vi "Core_Chem_User_Interface_v3.2.vi"() -> ()   [LabVIEW 2014]
uses:
  <vilib>/dex/Stream Element Allocation Mode.ctl
  C:/Program Files (x86)/National Instruments/LabVIEW 2014/examples/Data Communication/Network Streams/Simple Network Streams/support/Network Stream Command.ctl
  <vilib>/Platform/TimedLoop/XDataNode/timing_clust.ctl
  <vilib>/Platform/TimedLoop/XDataNode/nitl_modes.ctl
  <vilib>/Platform/TimedLoop/XDataNode/wakeup.ctl
  <vilib>/Utility/tcp.llb/UDP Multicast Read-Only Open.vi
  <vilib>/platform/TimedLoop/XDataNode/XDataNode.xnode
  <vilib>/Platform/TimedLoop/XDataNode/XDNodeRunTimeDep.lvlib
  <vilib>/FTP/NI_FTP.lvlib
panel:
  out "Create folder error out 3":errorcluster
  out "Network disconnected":bool
  out "cRIO connection status":bool
  out "Network Check error out":errorcluster
  out "SO2 Zeroing (Inflight)\nTime Remain (sec)":u32
  in  "eV6 User set time \n(Inflight) (sec)":i32=120
  in  "SO2 Inflight \nZeroing":bool
  out "Create folder error out 2":errorcluster
  out "Create folder error out":errorcluster
  in  "Confirm Flight Number":bool
  out "PRTAFT_UDP_In":string
  out "TWBOZO01":string
  out "CABOZO01":string
  out "TEIOZO01":string
  out "CHTSOO01":string
  out "CHFGGA01":string
  out "AL52CO01":string
  in  "Flight Number":string
  in  "Tab Control":T1(tab)
  out "FGGA preflight Des 17":string="Preflight - Start minimum 2 hours before take-off\n\n1. Ensure no bags/jackets are stowed on seat backs and behind seats in front of core chemistry rack at all times.\n\n2. Remove inlet covers if applicable.\n\n3. Connect Lilliput mini TFT/LCD VGA cable to FGGA VIDEO (back panel) and PS2 Keyboard/Mouse cables to FGGA Connectors (back panel). TFT/LCD screen kept in WAS/GAS rack Zargers Box. Keyboard/Mouse kept bottom of chemistry rack. (DO NOT disconnect PS2 cable). Connect TFT/LCD AC/DC PSU to 6026-8-98 Amphenol (SSP9) and make 230 Vac CB.\n\n4. Ensure all circuit breakers are pushed in, except 230Vac and 28Vdc, UPS switch off (down) and AL5002 CO Plasma Lamp switch off (down), WoW key to normal (horizontal).\n\n5. Wait for ALL network switches on the aircraft to be up and running before start-up. On the Flight Manager's Interface on the Flight Manager laptop, check SSP icons status (top row) should be all green.  \n\n6. Check AboutTime has synchronised laptop clock to aircraft timeservers (Filiberto/Gaston).\n\nClick the PowerUp Tab."
  out "FGGA preflight Des 16":string="PowerUp\n\n1.\tSSP9 forward face\tMake 3 CBs\n\n2.\tPWRDIST \t\tMake 230Vac CB \n                     Switch UPS On \t[UP]\n                     Make 28Vdc CB\n                     Check 28VDC OK Green Light comes on\n\n3.\tCore Chemistry e-Log\nComplete Core Chemistry e-Log in WordPad (Bnnn_CoreChemLog_v2.2), save on Flight Manager's laptop (192.168.101.180/      flt_folders/Bnnn); Fill in header with date, flight number and your name/initials.\n\n4. Wait for MFM flow rate to display non zero value.\n\n5.\tSAMPUMP\t\t\n - Switch WoW override key (vertical) to check pump starts, and MFM flowrate increase (>20 LPM) on the right hand plot. \n - Switch off WoW override\t\t\t\t [NORM, key horizontal]\n\nClick the 2B Ozone tab if operated, otherwise, click the UDP tab.\n\n\n"
  out "MFM":dbl(graph)
  in  "Ambient = OFF\nCabin = ON":bool
  out "FGGA preflight Des 15":string="2B Ozone Preflight\n\n1.\tSelect either Ambient or Cabin Air mode (default should be OFF for Ambient air mode).\n\n2. Check flowrate is greater than 2000 sccm on the right hand plot.\n\nClick the UDP tab."
  out "2B Ozone concentration":dbl(graph)
  out "2B Ozone flow rate":dbl(graph)
  out "2BOzone Event error out":errorcluster
  out "2BOzone command sender error out":errorcluster
  out "FGGA preflight Des 20":string="4. Check derived parameters in DECADES (192.168.101.110 & 192.168.101.108). 574 Ozone TEi49C; 588 CO AL5002; 611 SO2 TEi43i; 903 - 905 FGGA; 910 / 920 Ozone 2B."
  out "FGGA preflight Des 14":string="UDP Preflight\n1. Check all UDP packets are updating.  Unix time increasing by 1 sec (3rd parameter).\n2. Check flight number is correct.\n3. Confirm flight number and check it appears in the UDP packet (6th parameter). "
  in  "name":string="239.1.4.6"
  in  "Port":u16=50001
  out "FGGA":string
  out "CO":string
  out "TEi49 Ozone":string
  out "2B Cabin Ozone":string
  out "2B Ambient Ozone":string
  out "SO2":string
  in  "Ozone Zeroing Abort":bool
  out "Ozone Zeroing\nTime Remain (sec)":u32
  in  "Ozone Zeroing":bool
  out "TEI49 Sample Flow B":dbl(graph)
  out "TEi49 Concentration":dbl(graph)
  out "TEI49 Sample Flow A":dbl(graph)
  out "FGGA preflight Des 13":string="TEi49 Ozone PRE-FLIGHT - LAST ACTIONS BEFORE SEAT-BELTING DOWN (PRIOR TO ENGINES START)\n\n1. Ozone monitor zeroing\t\t[10 min minimum]\n\n\n2. Check TEi49 zero value and note down value in e-Log. \n"
  out "FGGA preflight Des 12":string="TEi49 Ozone Preflight\n\n1. Check nominal sample flowrate on both channels is ~0.7 LPM."
  out "Ozone Event error out":errorcluster
  out "Ozone command sender error out":errorcluster
  in  "Ozone UDP Time Offset":i32=1
  in  "eV8 span\n(sec)":i32=120
  in  "eV9 span\nflush (sec)":i32=60
  in  "SO2 Span Calibration":bool
  in  "eV9 zero\nflush (sec)":i32=15
  in  "SO2 Zero Calibration":bool
  in  "eV8 zero\n(sec)":i32=30
  in  "SO2 Calibration Abort":bool
  out "SO2 react pressure":dbl(graph)
  in  "Prepare SO2 Zero Gas":bool
  in  "Prepare SO2 Span Gas":bool
  in  "Auto Zeroing \ninterval (sec)":i32=600
  out "Next Auto Zero\nStarts in (sec)":u32
  out "Auto Zero\nIndicator":string="Auto Zero Inactive; Manual Zero Allow"
  out "SO2 Resume Zeroing\nCount down timer (sec)":u32
  in  "SO2 Pause\nAuto Zeroing":bool
  out "TEi43i Concentration scaled / raw":cluster{dbl, dbl}(graph)
  in  "SO2 Auto Zeroing":bool
  out "mean zero\ncal status":bool
  out "SO2 Sensitivity":dbl format="%.2g"
  out "SO2 Zero":dbl format="%.2g"
  in  "eV9 Flush User\nset time (sec)":i32=15
  in  "MFC_3 User Set Value":dbl=2.0
  in  "MFC_2 User Set Value":dbl=2.5
  in  "eV6 User\nset time (sec)":i32=600
  out "SO2 Flush\nTime Remain (sec)":u32
  out "TEI43i MFC3 Sample Flow":dbl(graph)
  out "TEI43C Sample Flow":dbl(graph)
  out "TEI43i MFC2 Cal Flow":dbl(graph)
  out "SO2 Zero CAL\nTime Remain (sec)":u32
  out "SO2 Zero CAL Flush\nTime Remain (sec)":u32
  in  "SO2 Zero CAL":bool
  out "FGGA preflight Des 11":string="TEi43 SO2 Inflight Zero Calibration"
  in  "SO2 GND Zeroing":bool
  out "SO2 Zeroing\nTime Remain (sec)":u32
  out "FGGA preflight Des 10":string="TEi43 SO2 PRE-FLIGHT - LAST ACTIONS BEFORE SEAT-BELTING DOWN (PRIOR TO ENGINES START)\n\n1. SO2 monitors zeroing\t\t[10 min minimum]\n\n2. Check TEi43i or TEi43C zero value and note down value in e-Log.\n\n3. Enable SO2 auto zeroing (if required) and check zeroing interval. "
  in  "SO2 Flush":bool
  out "FGGA preflight Des 9":string="TEi43 SO2 Preflight\n\n1. Check nominal sample flowrate is (2.0 LPM / 1.5 LPM) on the (TEi43i / TEi43c) right hand plot.\n\nSPAN GAS\n1. Connect SO2 Calibration gas to caldeck, then.\n\n2. Press SO2 flush button, MFC2 cal flow should increase to 2.5 SLPM.\nMonitor MFC2 flow rate to make sure the reading decreases from 2.5 SLPM to 0.0 SLPM.\nCheck pressure content and delivery gauges also reads zero.\nIf pressure content & delivery gauges do NOT read zero, press SO2 flush button again until they do.\n\n3. Back out V2, Quickly open and close cylinder valve 1, Set delivery pressure to 3 bar on V2. \n\n4. Repeat step 2) to 3) three times.\n\n5. Open cylinder valve 1, system is ready. Note down content pressure in elog.\n\n6. Press SO2 Span Calibration button to start Span calibration. \n\nZERO AIR\n1. Connect BTCA Zero Air gas to caldeck, then.\n\n2. Set ev9 flush user time to 60 secs and press SO2 Flush button.\n\n3. Press SO2 Zero Calibration button to start Zero Air calibration."
  in  "eV9 flush User\nset time (sec)":i32=30
  in  "eV8 User\nset time (sec)":i32=60
  out "SO2 Event error out":errorcluster
  out "SO2 command sender \nerror out":errorcluster
  in  "SO2 UDP Time Offset":i32=1
  in  "CO Monitor Troubleshooting":bool
  out "Lamp Temperature":dbl(graph)
  out "CO CAL Status":bool
  in  "CO CAL":bool
  out "FGGA preflight Des 8":string="CO Preflight and Inflight Calibrations\nHold down the CAL button for 2 secs then release, CAL status should then lit up.\nCheck CO LED lit up at front instrument. If not, refer to\nInflight calibration performed on 45 minutes interval or more frequently if lamp temperature > 35.5 degC."
  in  "Prepare Gases":bool
  out "FGGA preflight Des 7":string="AL5002 CO Preflight Checks\n\n1.\n\n2. Start CO Vacuum. NB: If there is problem with the software control, use manual override switch [up] on CALDECK front panel\n\n3. CO Checks - charts on the right hand side\n    Lamp Flow Controller ~ 40 ml/min\n    Monochromator Flow Controller ~ 30 ml/min\n    Fluorescence Cell Pressure ~ 7.5 Torr\n\nIf Lamp/Mono flows are low, manual valves (V1 -> V5) may still be shut, or pressure adjusting valves (ALREG1 & 2) have not been set > 2 bar\n\nIf Cell pressure is 10 Torr (max range), check that COPUMP is running and eV7 is opened (CO Vacuum eV7 is ON).\n\n4. Switch Plasma Lamp at the front panel UP\n\nDetector count rate (on 'Raw Signal' or F2 instrument touchscreen) should increase to >=10000 Hz within a minute.  Recycle plasma lamp switch (off/on) if no significant increase in count rate after 10 mins.  CO concentration should increase (100s ppb). \n     \n\n"
  in  "CO Vaccum (eV7)":bool
  out "Raw Signal":dbl(graph)
  out "CO Concentration":dbl(graph)
  out "Fluorescence Cell Pressure":dbl(graph)
  out "Monochromator Flow":dbl(graph)
  out "Lamp Flow Controller":dbl(graph)
  in  "CO UDP Time Offset":i32=1
  out "CO2 Pressure\nDelivery (PSIA)":dbl(slide) scale=0.0..100.0
  out "Std\nContent (barG)":dbl(slide) scale=0.0..220.0
  out "N2\nContent (barG)":dbl(slide) scale=0.0..220.0
  out "CO2\nContent (barG)":dbl(slide) scale=0.0..170.0
  out "CO Event error out":errorcluster
  out "CO command sender error out":errorcluster
  out "CO Zero":T2(array[cluster])
  out "CO Sensitivity":T3(array[cluster])
  in  "NEW\nFGGA Restart":bool
  in  "FGGA Calibration Abort":bool
  out "Ring Down Time RDA & RDB":cluster{dbl, dbl}(graph)
  in  "Line Lock Setting Change":bool
  out "Cell temperature":dbl(graph)
  out "Cell pressure":dbl(graph)
  in  "Manual FGGA Pump":bool
  out "CO2":dbl(graph)
  out "CH4":dbl(graph)
  out "H2O":dbl(graph)
  out "WoW Flag":string="0"
  in  "FGGA pump\nsync to WoW":bool
  out "CH4 Dry":dbl(graph)
  out "CO2 Dry":dbl(graph)
  out "MFC1 Cal Flow":dbl(graph)
  out "Flush Target Tank\nTime Remain (sec)":u32
  out "Flush Low Tank\nTime Remain (sec)":u32
  out "Flush High Tank\nTime Remain (sec)":u32
  in  "Flush Target Tank":bool
  in  "Flush Low Tank":bool
  in  "Flush High Tank":bool
  in  "OLD\nFGGA Restart":bool
  out "FGGA preflight Des 6":string="FGGA Instrument Controls"
  in  "High Cal":bool
  out "High Cal\nFlush Time Remain (sec)":u32
  out "High Cal\nCal Time Remain (sec)":u32
  in  "Low Cal":bool
  in  "Target Cal":bool
  in  "Span Cal - \nHigh Cal, CO Cal, Low Cal":bool
  out "Low Cal\nFlush Time Remain (sec)":u32
  out "Low Cal\nCal Time Remain (sec)":u32
  out "Target Cal\nFlush Time Remain (sec)":u32
  out "Target Cal\nCal Time Remain (sec)":u32
  in  "MFC_1 User Set Value":dbl=2.0
  out "FGGA preflight Des 5":string="FGGA Inflight Calibrations"
  out "FGGA preflight Des 4":string="FGGA Ground Preflight Checks\n\n1. Switch FGGA pump ON\n\n2. Check cavity pressure ~50 Torr\n\n3. Switch FGGA pump OFF\n\n4. Enable FGGA pump sync to WoW\n\n5.. Check Time Synchronisation\n\n6. Check CO2 & CH4 values\n\nIf CO2 & CH4 values are -1 ppm, follow the \nchange linelock settings procedure.\n\n\n\n\n\nLAST ACTION BEFORE SEAT-BELTING \nDOWN (PRIOR TO ENGINES START)\n\n1. Disconnect Monitor & stow away. Leave Keyboard & Mouse connected. Place keyboard at the bottom\nof the rack.\n\n"
  out "FGGA preflight Des 3":string="FGGA CAL Gas Purge\n\nFor each cylinder in gas stowage, check that,\n\n1. V1 Closed\n    V3 Closed\n    V4 Make sure arrow positioned downwards (i.e. flow points to gas line)\n\n2. V3 Open (turn anti-clockwise)\n\n3. Use the button on the right according to the operating cylinder to flush the line. Monitor the MFC flow rate to make sure the reading decreases from 3 to zero. (ie fully flushed). Pressure content & delivery gauges should also read zero.\n\n4. V3 Close (turn clockwise)\n\n5. V1 Open / Close quickly\n         Check delivery pressure gauge is ~ 40 PSI \n         (Use V2 to increase if necessary)\n\n6. Repeat steps 2) to 5) three times\n\n7. V3 Close (turn clockwise)\n\n8. V1 Open, check V2 ~ 40 PSIG\n\n9. V3 Open - System is ready"
  out "FGGA command sender error out":errorcluster
  out "FGGA Event Error out":errorcluster
  in  "FGGA UDP Time Offset":i32=1
  in  "NEW FGGA Shutdown":bool
  in  "Transfer NEW FGGA Files":bool
  in  "OLD FGGA Shutdown":bool
  in  "Postflight Procedures":bool
  in  "FTP ASCII Files to Local":bool
  in  "Transfer OLD FGGA Files":bool
  out "FGGA preflight Des 18":string="Postflight\n\n1. Perform SO2 Span Gas Calibration (if necessary). \n\n2. Press the FTP ASCII File to Local button to transfer ASCII files to flight folder.\n\n\n3. Press the Transfer FGGA Files button to transfer FGGA files to flight folder. \n\n\n4. Shutdown FGGA.\n\n\n5. View Postflight Procedures."
  out "File List":string[](array[string])
  out "FGGA File Transfer Error out":errorcluster
  out "Move to FM Error out":errorcluster
  out "FGGA File Transfer Error out 2":errorcluster
  out "USB Disk Space Used %":dbl(slide) scale=0.0..100.0
  out "PTP Sync":bool
  out "CPU Total %":dbl(graph)
  out "PRTAFT_DLU":string
  in  "Pause Auto Zero Count \nDown set time (sec)":i32=600
  out "Calibration gas cylinder \nconcentration (ppb)":dbl format="%.4g"
  in  "Save Calibration gas\ncylinder concentration to file":bool
  in  "Calibration gas cylinder \nconcentration (ppb)":dbl=500.0 format="%.4g"
  in  "Simulate MOCCA Conc":dbl
  in  "MOCCA window \ndelay time (sec)":i32=30
  in  "MOCCA Limit":i32=800
  in  "SO2 Inflight MOCCA Alarm\n(default = OFF)":bool
  in  "Offset Mean Zero Calculation (default = ON)\nOFF = User input\nOn = Mean zero calculated with ev8":bool=TRUE
  out "FGGA preflight Des 19":string="This tab controls ONLY for advanced operators."
  in  "Inst_alm_thresh":i32=220
  in  "3hr_alm_thresh":i32=80
  in  "Simulate Inst Conc":i32
  in  "Simulate 3hr Average Conc":dbl
  in  "Simulate 2B Conc":bool
  in  "Ozone eV6":bool
  in  "Simulate Conc":bool
  in  "8hr TWA Limit":i32=490
  in  "10mins STEL Limit":i32=800
  in  "SO2 Sensitivity":dbl=1.1
  in  "SO2 Zero":dbl
  in  "Simulate TWA Conc":dbl
  in  "Simulate STEL Conc":dbl
  in  "MFC_3\nSLPM Value":dbl=2.0
  in  "MFC_2\nSLPM Value":dbl
  in  "SO2 eV6":bool
  in  "eV8":bool
  in  "eV9":bool
  in  "eV4":bool
  in  "eV3":bool
  in  "MFC_1\nSLPM Value":dbl
  in  "eV2":bool
  in  "eV1":bool
  in  "cRIO File IO Stop\n(USB Flash Drive Unmount)":bool
  # "Unix time"
  # "Flight Number"
  # "concentration (scaled)\npmt_volt\nlamp_volt\nlamp_intens\ninternal_temper\nreact_temper\nreact_press\nflow\nflags\nten_min_so2\neight_hr_so2\nten_min_so2_alm\neight_hr_so2_alm\nMFC_2absolute_pres\nMFC_2temperature\nMFC_2volumetic_flow\nMFC_2mass_flow\nMFC_2set_point\nMFC_3_absolute_pres\nMFC_3_temperature\nMFC_3volumetic_flow\nMFC_3mass_flow\nMFC_3set_point\nV6\nV8\nV9\nMFC2_Set_Value\nMFC3_Set_Value\nconcentration (raw)\nmean calculation status\noffset\nsensitivity\nev8_user_set_time\nauto_zeroing_control\nev8_zero_interval\nMOCCA_inflight_alarm\nMOCCA_time_window_delay\nMOCCA_SO2_limit\n10 min STEL limit\n8 hour TWA limit\nSO2 cal gas cylin conc\nsimulate_SO2_conc_control\nMOCCA_SO2_sim_value\nMOCCA_SO2_alarm"
  # "Unix time"
  # "Unix time"
  # "Unix time"
  # "Unix time"
  # "Flight Number"
  # "Flight Number"
  # "Flight Number"
  # "Flight Number"
  # "conc\ntemp\npress\nflow\nthreehr_oz\nInst_alarm\nthreehr_alarm"
  # "ch4\nco2\nh2o\npress_torr\ntemp_c\nfit_flag\nrda_usec\nrdb_usec\nch4_dry\nco2_dry\nMFC_1_absolute_pres\nMFC_1_temperature\nMFC_1volumetic_flow\nMFC_1mass_flow\nMFC_1set_point\nV1\nV2\nV3\nV4\nrestart_FGGA\nFGGA_Pump\nCAL_MFC_1Set_Value"
  # "conc\ntemp\npress\nflow"
  # "conc\nbenchtemp\npress\ncellAint\ncellBint\nFlowA\nFlowB\nlamptemp\nflag\nV6"
  # "conc\ncounts\nsens\nzero\nlampflow\nlamptemp\nmonoflow\nmonotemp\nmonopress\ncellpress\ncalpress\ntemppmt\ncalconc\nerr\ncal_counter\nerr_counter\nCO_vacuum_status\nIn_Cal\nALEG1_press_delivery\nALREG1_press_content\nALREG2_press_content\nALREG3_press_content"
  # "TEi43c"
  # "TEi43i"
  # "SO2 Inflight ZERO CAL SETTINGS"
  # "FGGA"
  # "2B Ozone"
  # "TEi49C  - Ozone"
  # "TEi43 - SO2"
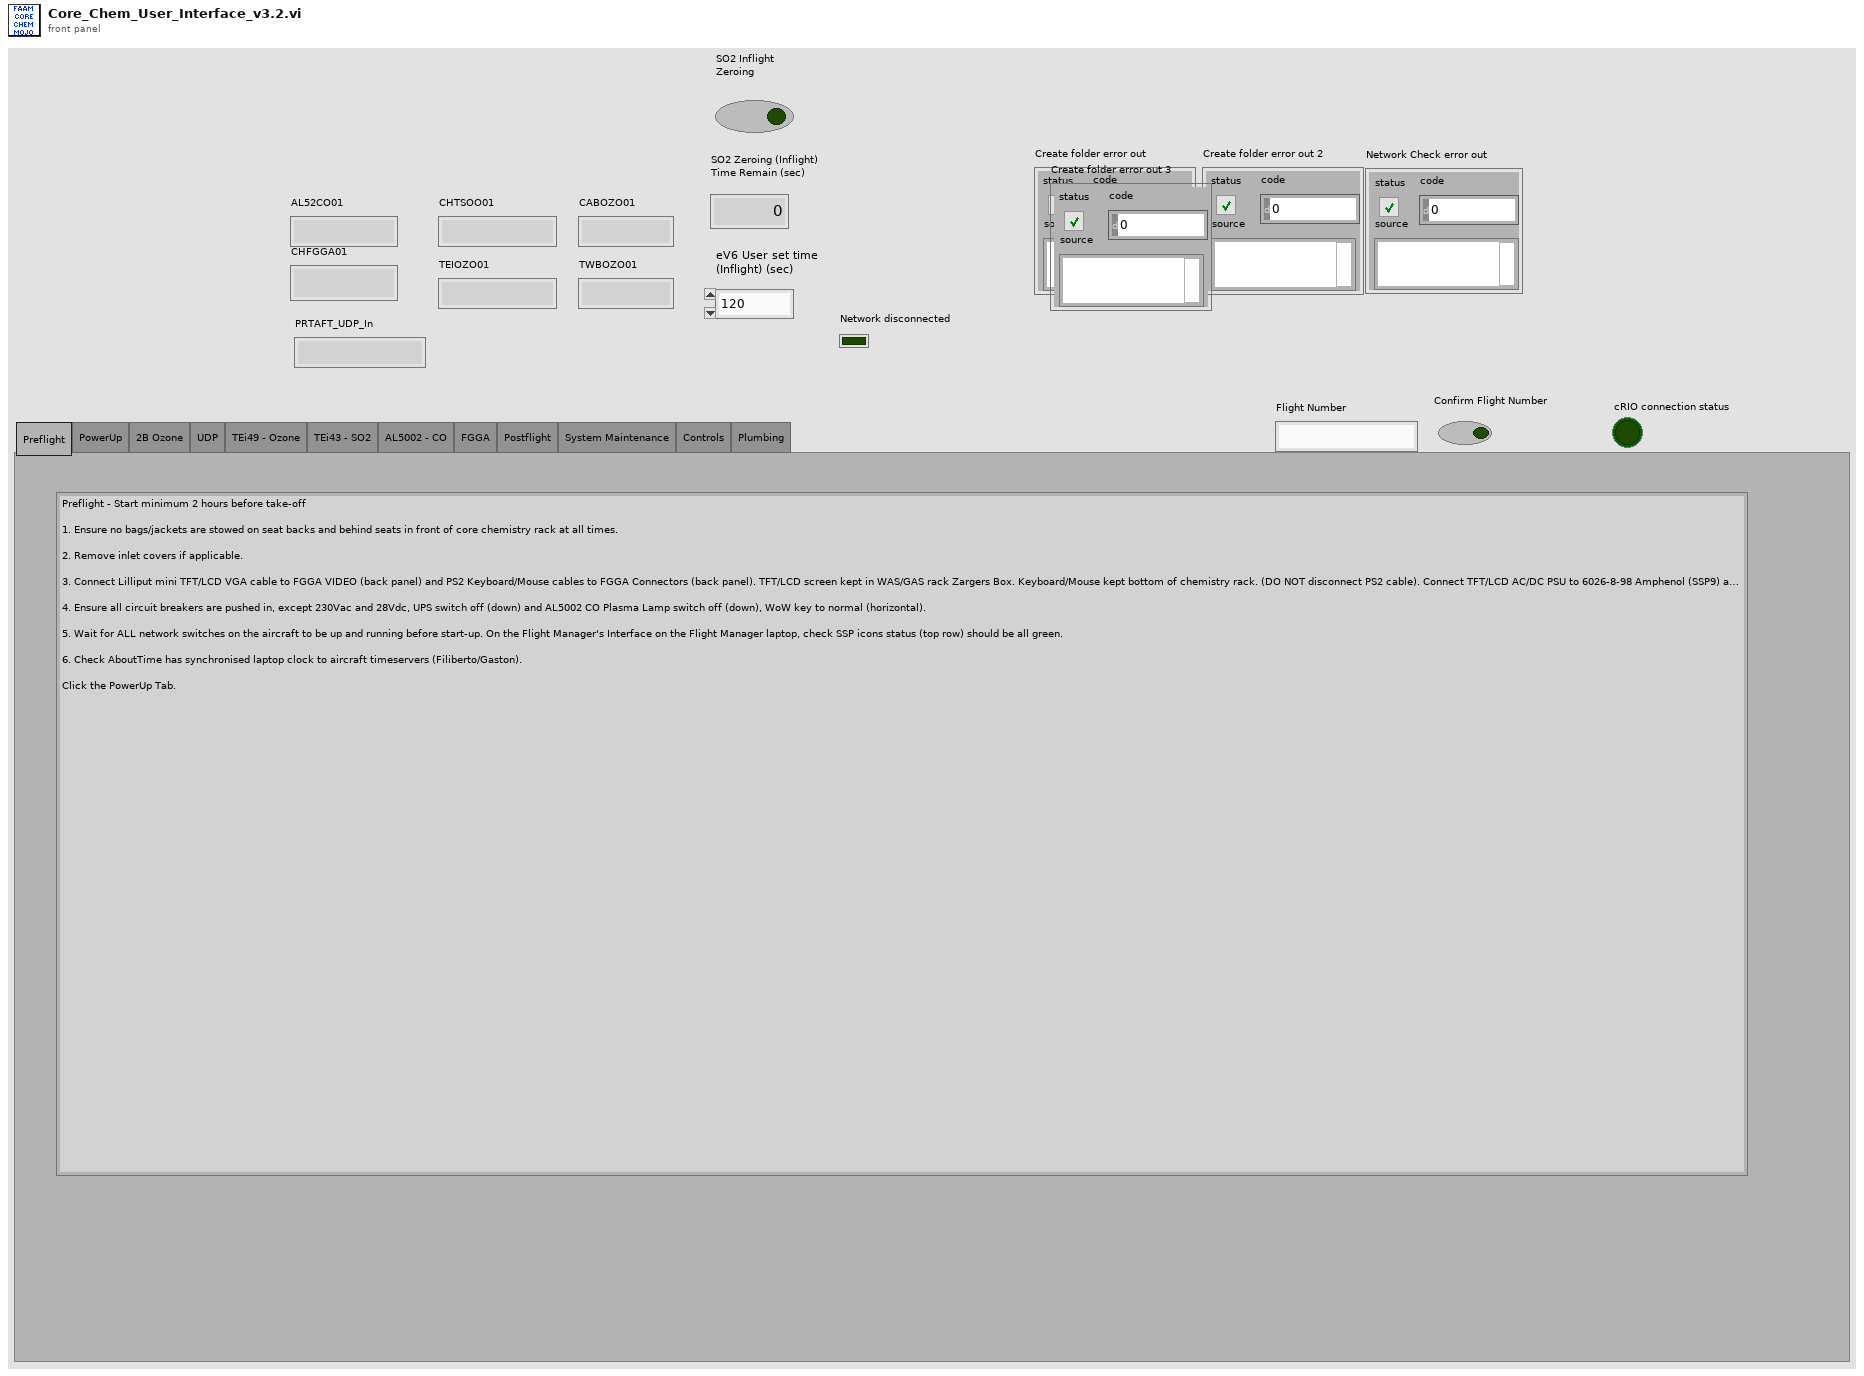
[diagram p1: front panel]
types:
  T1 = enum32{"Preflight", "PowerUp", "2B Ozone", "UDP", "TEi49 - Ozone", "TEi43 - SO2", "AL5002 - CO", "FGGA", "Postflight", "System Maintenance", "Controls", "Plumbing"}
  T2 = cluster{"time stamp":timestamp, "CO Offset":dbl}[]
  T3 = cluster{"time stamp":timestamp, "CO Sensitivity":dbl}[]
  T4 = typedef "Network Stream Command.ctl" = cluster{"Message":string, "Message Data":variant}
  T5 = typedef "Stream Element Allocation Mode.ctl" = u32
  T6 = typedef "XDNodeRunTimeDep.lvlib/timing_clust.ctl" = cluster{"Expected End [f-1]":u64, "Actual End [f-1]":u64, "Finished Late? [f-1]":bool, "Expected End [i-1]":u64, "Actual End [i-1]":u64, "Finished Late? [i-1]":bool, "Expected Start [i]":u64, "Actual Start [i]":u64, "Expected Start [f]":u64, "Actual Start [f]":u64, "Source Name":string, "Structure Name":string, "Period":i64, "Deadline":i64, "Offset":i64, "Start":i64, "Priority":i32, "Timeout":i32, "Mode":T7, "Wakeup Reason":T8, "Error":errorcluster, "Source Type":string, "Secondary Source Type":string, "Global End Time":u64, "Global Start Time":u64, "Frame Duration":u64, "Iteration Duration":u64, "Assigned CPU":i32, "I/O Scan Engine Mode":u32}
  T7 = typedef "XDNodeRunTimeDep.lvlib/nitl_modes.ctl" = enum32{"No Change", "Process missed periods, maintain original phase", "Discard missed periods, maintain original phase", "Process missed periods, ignore original phase", "Discard missed periods, ignore original phase"}
  T8 = typedef "XDNodeRunTimeDep.lvlib/wakeup.ctl" = enum32{"Normal", "Aborted", "Asynchronous wakeup", "Timing source error", "Timed loop error", "Timeout"}
  T9 = typedef "NI_FTP.lvlib/FTP Session.ctl" = refnum<k5>
  T10 = typedef "NI_FTP.lvlib/FTP File Info.ctl" = cluster{"type":enum16{"unknown", "file", "dir", "link"}, "permissions":string, "owner":string, "group":string, "size":i32, "date":string, "name":string, "link name":string}
  T11 = cluster{"Message":string, "Message 2":string, "Message 3":string}
  T12 = cluster{"Message":string, "Message 2":string, "Message 3":string, "Message 4":string}
  T13 = cluster{"Message":string, "Message 3":string, "Message 4":string}
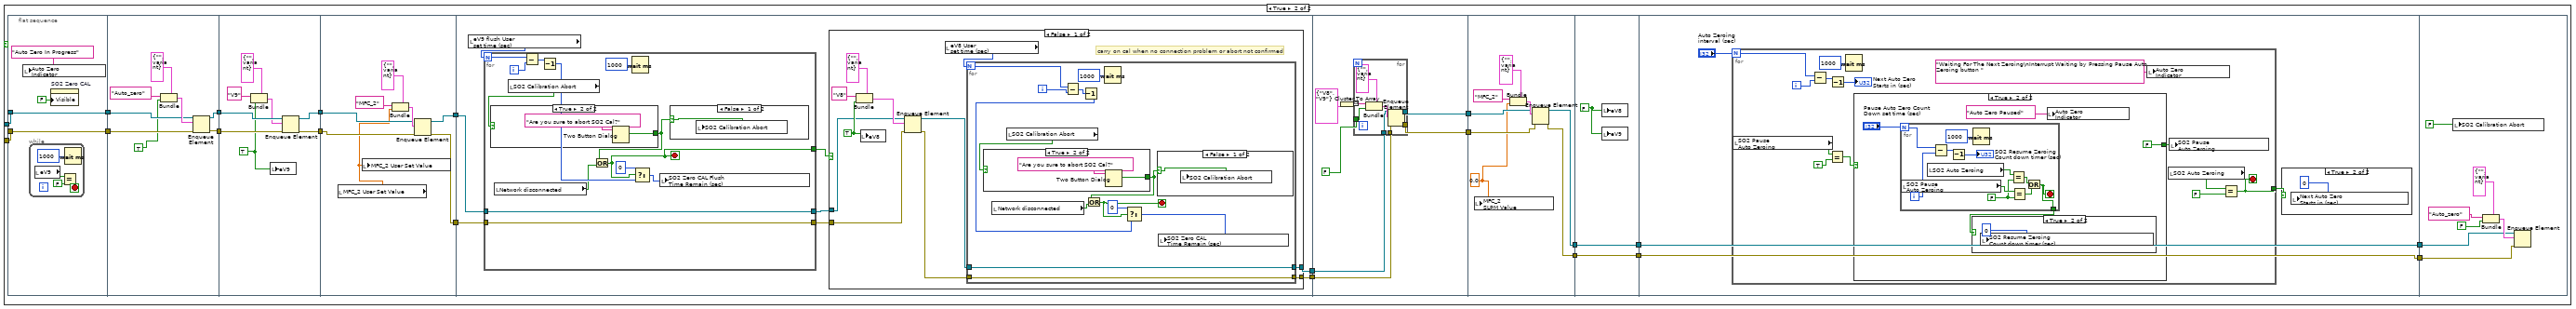
[diagram p6: hidden frame]
diagram:
  w8 = "XXXX"
  w10 = 0
  w11 = 0.0
  w17 = T4 {"Message"="", "Message Data"=variant} ("Message Cluster")
  w23 = T5 0 items=["allocate as needed", "pre-allocate"] ("element allocation mode")
  w29 = T4 {"Message"="", "Message Data"=variant} ("Message Cluster")
  w35 = T5 0 items=["allocate as needed", "pre-allocate"] ("element allocation mode")
  w40 = T4 {"Message"="", "Message Data"=variant} ("Message Cluster")
  w45 = T5 0 items=["allocate as needed", "pre-allocate"] ("element allocation mode")
  w54 = T5 0 items=["allocate as needed", "pre-allocate"] ("element allocation mode")
  w56 = T4 {"Message"="", "Message Data"=variant} ("Message Cluster")
  w63 = T5 0 items=["allocate as needed", "pre-allocate"] ("element allocation mode")
  w65 = T4 {"Message"="", "Message Data"=variant} ("Message Cluster")
  n1 = local write "cRIO File IO Stop\n(USB Flash Drive Unmount)"(FALSE ("Stop File Write")) -> ()
  n2 = local write "Flight Number"(w8) -> ()
  n3 = while {
    shift-right: [w69] -> _
    shift-left: w8 -> [w68]
    stop <- FALSE stop-if-true
    n4 = Not Equal?(x=w68, y="Flight Number") -> (x != y?=w71:bool)
    n5 = case shown="True" w71 {
      tunnel: [w74 w75] -> w69
      tunnel: "Flight Number" -> [_ w75]
      tunnel: w68 -> [w74 _]
      frame False {
      }
      frame True {
        n6 = One Button Dialog(message="Flight Number changed,\nPress flight number button to confirm") -> ()  [unwired: 1 in, 1 out]
      }
    }
    n7 = Wait (ms)(milliseconds to wait=u32 1000) -> ()  [unwired: 1 out]
  }
  n8 = while {
    stop <- FALSE stop-if-true
    # "UDP Read"
    n9 = String To IP(1:"name") -> (0:w82:u32)
    n10 = call-poly <vilib>:"UDP Multicast Open.vi"("multicast addr"=w82, "port"="Port") -> ("error out"=w80:errorcluster, "connection ID"=w79:refnum<k16>)  [unwired: 7 in, 1 out]
    n11 = Wait (ms)(milliseconds to wait=u32 1000) -> ()  [unwired: 1 out]
    n12 = case shown="No Error" w80 {
      selector: w80 -> [w86 _]
      tunnel: w79 -> [w85 _]
      frame No Error {
        w84 = ""
        n13 = while {
          tunnel: w86 -> [w132]
          tunnel: w85 -> [w131]
          shift-right: [w127] -> _
          shift-left: w84 -> [w128]
          shift-right: [w118] -> _
          shift-left: w84 -> [w120]
          shift-right: [w112] -> _
          shift-left: w84 -> [w114]
          shift-right: [w106] -> _
          shift-left: w84 -> [w107]
          shift-right: [w100] -> _
          shift-left: w84 -> [w101]
          shift-right: [w94] -> _
          shift-left: w84 -> [w95]
          shift-right: [w88] -> _
          shift-left: w84 -> [w89]
          stop <- w130 stop-if-true
          n14 = UDP Read(connection ID=w131, 8:w132) -> (data out=w87:string, error out=w130:errorcluster)  [unwired: 2 in, 3 out]
          n15 = Match Pattern(string=w87, regular expression="$TEIOZO") -> (match substring=w126:string, after substring=w125:string)  [unwired: 1 in, 2 out]
          n16 = Match Pattern(string=w87, regular expression="$TWBOZO01,") -> (match substring=w104:string, after substring=w103:string)  [unwired: 1 in, 2 out]
          n17 = Match Pattern(string=w87, regular expression="$CABOZO01,") -> (match substring=w110:string, after substring=w109:string)  [unwired: 1 in, 2 out]
          n18 = Match Pattern(string=w87, regular expression="$CHTSOO") -> (match substring=w98:string, after substring=w97:string)  [unwired: 1 in, 2 out]
          n19 = Match Pattern(string=w87, regular expression="$CHFGGA") -> (match substring=w122:string, after substring=w121:string)  [unwired: 1 in, 2 out]
          n20 = Match Pattern(string=w87, regular expression="$AL52CO01,") -> (match substring=w116:string, after substring=w115:string)  [unwired: 1 in, 2 out]
          n21 = Match Pattern(string=w87, regular expression="$PRTAFT01,") -> (match substring=w93:string, after substring=w92:string)  [unwired: 1 in, 2 out]
          n22 = Concatenate Strings(w126, w125) -> (w124:string)
          n23 = Concatenate Strings(w104, w103) -> (w102:string)
          n24 = Concatenate Strings(w110, w109) -> (w108:string)
          n25 = Concatenate Strings(w98, w97) -> (w96:string)
          n26 = Concatenate Strings(w122, w121) -> (w119:string)
          n27 = Concatenate Strings(w116, w115) -> (w113:string)
          n28 = Concatenate Strings(w93, w92) -> (w90:string)
          n29 = Replace Substring(4:w102, 5:w101) -> (1:w100:string)  [unwired: 2 in, 1 out]
          "TWBOZO01" <- w100
          n30 = Replace Substring(4:w124, 5:w128) -> (1:w127:string)  [unwired: 2 in, 1 out]
          "TEIOZO01" <- w127
          n31 = Replace Substring(4:w108, 5:w107) -> (1:w106:string)  [unwired: 2 in, 1 out]
          "CABOZO01" <- w106
          n32 = Replace Substring(4:w96, 5:w95) -> (1:w94:string)  [unwired: 2 in, 1 out]
          "CHTSOO01" <- w94
          n33 = Replace Substring(4:w113, 5:w114) -> (1:w112:string)  [unwired: 2 in, 1 out]
          "AL52CO01" <- w112
          n34 = Replace Substring(4:w119, 5:w120) -> (1:w118:string)  [unwired: 2 in, 1 out]
          "CHFGGA01" <- w118
          n35 = Replace Substring(4:w90, 5:w89) -> (1:w88:string)  [unwired: 2 in, 1 out]
          "PRTAFT_UDP_In" <- w88
        }
      }
      frame Error {
      }
    }
  }
  n36 = Obtain Queue(name (unnamed)="CO_Command", element data type=w65) -> (queue out=w16:refnum<queue>, error out=w59:errorcluster)  [unwired: 3 in, 1 out]
  n37 = Create Network Stream Writer Endpoint(6:w63, 7:10 ("writer buffer size"), 9:w65, 10:"//192.168.101.17/command/reader/CO" ("reader url"), 11:"/command/writer/CO" ("writer name")) -> (0:w62:errorcluster, 3:w61:refnum<k21>)  [unwired: 2 in]
  n38 = while {
    tunnel: w16 -> [w136]
    tunnel: w59 -> [w135]
    tunnel: [w133] -> _
    stop <- FALSE stop-if-true
    # "CO UI Event Handler Loop"
    n39 = event shown="[4] \"Confirm Flight Number\": Value Change" {
      selector: _ -> [_ _ _ _ _]
      dyn-events: _ -> [_ _ _ _ _]
      timeout: _ -> [_ _ _ _ _]
      tunnel: w136 -> [w143 w150 w154 w161 w169]
      tunnel: w135 -> [w142 w149 w153 w160 w168]
      tunnel: [w137 w144 w152 w159 w167] -> w133
      event "CO CAL": Value Change {
        n40 = event-data() -> ("NewVal"=w140:bool)  [unwired: 1 in]
        n41 = Bundle(cluster=T4 {"Message"="", "Message Data"=variant} ("Message Cluster"), "Message"="CO CAL", "Message Data"=w140) -> (w138:T4)
        n42 = Enqueue Element(queue=w143, element=w138, error in (no error)=w142) -> (error out=w137:errorcluster)  [unwired: 1 in, 2 out]
      }
      event "CO UDP Time Offset": Value Change {
        n43 = event-data() -> ("NewVal"=w147:i32)  [unwired: 1 in]
        n44 = Bundle(cluster=T4 {"Message"="", "Message Data"=variant} ("Message Cluster"), "Message"="UDP Time Offset", "Message Data"=w147) -> (w145:T4)
        n45 = Enqueue Element(queue=w150, element=w145, error in (no error)=w149) -> (error out=w144:errorcluster)  [unwired: 1 in, 2 out]
      }
      event "CO Vaccum (eV7)": Value Change {
        n46 = event-data() -> ("NewVal"=w151:bool)  [unwired: 1 in]
        n47 = Bundle(cluster=T4 {"Message"="", "Message Data"=variant} ("Message Cluster"), "Message"="CO Vacuum", "Message Data"=w151) -> (w155:T4)
        n48 = Enqueue Element(queue=w154, element=w155, error in (no error)=w153) -> (error out=w152:errorcluster)  [unwired: 1 in, 2 out]
      }
      event "cRIO File IO Stop\n(USB Flash Drive Unmount)": Value Change {
        n49 = event-data() -> ("NewVal"=w158:bool)  [unwired: 1 in]
        n50 = Bundle(cluster=T4 {"Message"="", "Message Data"=variant} ("Message Cluster"), "Message"="Stop File Write", "Message Data"=w158) -> (w162:T4)
        n51 = Enqueue Element(queue=w161, element=w162, error in (no error)=w160) -> (error out=w159:errorcluster)  [unwired: 1 in, 2 out]
      }
      event "Confirm Flight Number": Value Change {
        n52 = event-data() -> ()  [unwired: 1 in, 1 out]
        n53 = flat-sequence {
          tunnel: w168 -> [w171]
          tunnel: w169 -> [w172]
          tunnel: [w172] -> w166
          tunnel: [w171] -> w165
          tunnel: [w174] -> w167
          tunnel: w166 -> [w176]
          tunnel: w165 -> [w175]
          frame #0 {
            n54 = local write "cRIO File IO Stop\n(USB Flash Drive Unmount)"(FALSE ("cRIO File IO Stop\n(USB Flash Drive Unmount)")) -> ()
          }
          frame #1 {
            n55 = local read "Flight Number"() -> (w173:string)
            n56 = Bundle(cluster=T4 {"Message"="", "Message Data"=variant} ("Message Cluster"), "Message"="Flight Number", "Message Data"=w173) -> (w177:T4)
            n57 = Enqueue Element(queue=w176, element=w177, error in (no error)=w175) -> (error out=w174:errorcluster)  [unwired: 1 in, 2 out]
          }
        }
      }
    }
    "CO Event error out" <- w133
  }
  n58 = while {
    tunnel: w16 -> [w187]
    shift-right: [w182] -> _
    shift-left: w61 -> [w184]
    shift-right: [w180] -> w50
    shift-left: w62 -> [w186]
    tunnel: w59 -> [w181]
    stop <- w180 stop-if-true
    # "CO UI Command Sender"
    n59 = Dequeue Element(queue=w187, error in (no error)=w181) -> (element=w183:T4)  [unwired: 1 in, 3 out]
    n60 = Unbundle By Name(w183) -> ("Message"=w185:string)
    n61 = case shown="\"UDP Time Offset\"" w185 {
      tunnel: w186 -> [w188 w192 w199 w206 w213 w220]
      tunnel: w184 -> [w189 w195 w202 w209 w216 w223]
      tunnel: w183 -> [_ w194 w201 w208 w215 w222]
      tunnel: [w188 w191 w198 w205 w212 w219] -> w180
      tunnel: [w189 w190 w197 w204 w211 w218] -> w182
      frame "False", Default {
      }
      frame "CO CAL" {
        n62 = shared-variable-write(w195, w192, w194) -> (w193:refnum<k21>, w196:errorcluster)  [unwired: 1 in, 1 out]
        n63 = Flush Stream(8:w196, 11:w193) -> (0:w191:errorcluster, 3:w190:refnum<k21>)  [unwired: 2 in, 1 out]
      }
      frame "UDP Time Offset" {
        n64 = shared-variable-write(w202, w199, w201) -> (w200:refnum<k21>, w203:errorcluster)  [unwired: 1 in, 1 out]
        n65 = Flush Stream(8:w203, 11:w200) -> (0:w198:errorcluster, 3:w197:refnum<k21>)  [unwired: 2 in, 1 out]
      }
      frame "Stop File Write" {
        n66 = shared-variable-write(w209, w206, w208) -> (w207:refnum<k21>, w210:errorcluster)  [unwired: 1 in, 1 out]
        n67 = Flush Stream(8:w210, 11:w207) -> (0:w205:errorcluster, 3:w204:refnum<k21>)  [unwired: 2 in, 1 out]
      }
      frame "Flight Number" {
        n68 = shared-variable-write(w216, w213, w215) -> (w214:refnum<k21>, w217:errorcluster)  [unwired: 1 in, 1 out]
        n69 = Flush Stream(8:w217, 11:w214) -> (0:w212:errorcluster, 3:w211:refnum<k21>)  [unwired: 2 in, 1 out]
      }
      frame "CO Vacuum" {
        n70 = shared-variable-write(w223, w220, w222) -> (w221:refnum<k21>, w224:errorcluster)  [unwired: 1 in, 1 out]
        n71 = Flush Stream(8:w224, 11:w221) -> (0:w219:errorcluster, 3:w218:refnum<k21>)  [unwired: 2 in, 1 out]
      }
    }
  }
  "CO command sender error out" <- w50
  n72 = node-c288() -> (w15:T6)  [unwired: 4 in]
  n73 = Initialize Array(cluster{"time stamp":timestamp, "Y":dbl} {"time stamp"=timestamp(0 s since 1904-01-01), "Y"=0.0}, 30 ("dimension size")) -> (w12:cluster{"time stamp":timestamp, "Y":dbl}[])
  n74 = timed-loop {
    timing: w15 -> [_]
    timing-out: [_] -> w14
    stop <- _ stop-if-true
    # "PC Tasks"
    n75 = node-c288() -> ()  [unwired: 1 in, 1 out]
    n76 = event shown="[2] \"Transfer NEW FGGA Files\": Value Change" {
      selector: _ -> [_ _ _ _ _ _ _]
      dyn-events: _ -> [_ _ _ _ _ _ _]
      timeout: _ -> [_ _ _ _ _ _ _]
      event "FTP ASCII Files to Local": Value Change {
        n77 = event-data() -> ()  [unwired: 1 in, 1 out]
        n78 = flat-sequence {
          tunnel: [w233] -> w227
          tunnel: [w245] -> w232
          tunnel: [w244] -> w230
          tunnel: [w243] -> w228
          tunnel: w227 -> [w243]
          tunnel: w232 -> [w303]
          tunnel: [w303] -> w231
          tunnel: w230 -> [w299]
          tunnel: [w298] -> w229
          tunnel: w228 -> [w298]
          tunnel: w231 -> [w309]
          tunnel: w229 -> [w304]
          frame #0 {
            n79 = local read "Flight Number"() -> (w235:string)
            n80 = Concatenate Strings("Confirm Flight Number" ("message"), "\n", w235) -> (w239:string)
            n81 = Two Button Dialog(message=w239, 1:"No" ("F button name (\"Cancel\")"), 2:"Yes" ("T button name (\"OK\")")) -> (T button?=w236:bool)
            n82 = case shown="False" w236 {
              tunnel: w235 -> [_ w242]
              tunnel: [w241 w242] -> w233
              frame False {
                n83 = call "Prompt User for Flight Number2"() -> ("Flight Number BXXX"=w241:string)  [unwired: 17 in, 2 out]
              }
              frame True {
              }
            }
          }
          frame #1 {
            n84 = Get Date/Time In Seconds() -> (seconds since 1Jan1904=w249:timestamp)
            n85 = Format Date/Time String(time format string (%c)="%Y%m%d", seconds (now)=w249) -> (date/time string=w247:string)  [unwired: 1 in]
            n86 = call <vilib>:"FTP Open Session.vi"("address"="192.168.101.17") -> ("error out"=w264:errorcluster, "ftp session"=w265:T9)  [unwired: 7 in, 2 out]
            n87 = Concatenate Strings("Use Today's Date" ("message"), "\r", w247) -> (w253:string)
            n88 = call <vilib>:"FTP Logon.vi"("error in (no error)"=w264, "password"="", "user"="anonymous", "ftp session"=w265) -> ("error out"=w261:errorcluster, "ftp session out"=w260:T9)  [unwired: 4 in, 2 out]
            n89 = Two Button Dialog(message=w253, 1:"No" ("F button name (\"Cancel\")"), 2:"Yes" ("T button name (\"OK\")")) -> (T button?=w250:bool)
            n90 = case shown="False" w250 {
              tunnel: [w268 w269] -> w244
              tunnel: w247 -> [_ w269]
              frame False {
                n91 = call "Prompt User for Date"() -> ("Date"=w268:string)  [unwired: 17 in, 2 out]
              }
              frame True {
              }
            }
            n92 = call <vilib>:"FTP Directory Listing.vi"("error in (no error)"=w261, "directory path"="/U:/data", "ftp session"=w260) -> ("dir list"=w259:T10[])  [unwired: 4 in, 4 out]
            n93 = for {
              tunnel: w259 -> [w289] mode=indexing
              tunnel: [w288] -> w256 mode=indexing
              tunnel: w244 -> [w287]
              # "Extract File Name According to the Date"
              n94 = Unbundle By Name(w289) -> ("name"=w295:string, "name"=w294:string)
              n95 = Match Pattern(string=w294, regular expression="_[0-9]+") -> (match substring=w292:string)  [unwired: 1 in, 3 out]
              n96 = String Subset(string=w292, offset (0)=1) -> (substring=w290:string)  [unwired: 1 in]
              n97 = Equal?(x=w290, y=w287) -> (x = y?=w296:bool)
              n98 = case shown="False" w296 {
                tunnel: w295 -> [_ w297]
                tunnel: [_ w297] -> w288
                frame False {
                }
                frame True {
                }
              }
            }
            n99 = Array Size(array=w256) -> (size(s)=w258:i32)
            n100 = for {
              N: w258 -> [_]
              shift-right: [w276] -> w246
              shift-left: w256 -> [w277]
              shift-right: [w274] -> _
              shift-left: 0 -> [w275]
              # "Remove Empty Array"
              n101 = Index Array(array=w277, index=w275) -> (element=w279:string)
              n102 = Equal?(x=w279, y="") -> (x = y?=w278:bool)
              n103 = case shown="True" w278 {
                tunnel: w277 -> [w283 w286]
                tunnel: w275 -> [w282 w284]
                tunnel: [w283 w285] -> w276
                tunnel: [w281 w284] -> w274
                frame False {
                  n104 = Increment(x=w282) -> (x+1=w281:i32)
                }
                frame True {
                  n105 = Delete From Array(array=w286, index=w284) -> (array with subset deleted=w285:string[])  [unwired: 1 in, 1 out]
                }
              }
            }
            "File List" <- w246
            n106 = for {
              tunnel: w246 -> [w272] mode=indexing
              tunnel: [w270] -> w245 mode=indexing
              # "Specify destination path for each file"
              n107 = Concatenate Strings("C:\\temp\\", w272) -> (w271:string)
              n108 = String To Path(string=w271) -> (path=w270:path)
            }
          }
          frame #2 {
            # "FTP a list of files"
            n109 = call <vilib>:"System Exec.vi"("wait until completion? (T)"=TRUE, "working directory"=path "C:/temp", "standard input"=w299, "command line"="C:\\temp\\transfer_ascii_files.bat") -> ()  [unwired: 4 in, 4 out]
          }
          frame #3 {
            # "Move file from local PC to Flight Folder"
            n110 = Build Path(base path=path "\\\\192.168.101.180\\flt_folders" ("path"), name or relative path=w304) -> (appended path=w311:path)
            n111 = Concatenate Strings(w304, "_" ("string"), "corechem" ("string")) -> (w310:string)
            n112 = Build Path(base path=w311, name or relative path=w310) -> (appended path=w306:path)
            n113 = Create Folder(path (use dialog)=w306) -> (created path=w305:path, error out=→"Create folder error out 2":errorcluster)  [unwired: 2 in, 1 out]
            n114 = for {
              tunnel: w305 -> [w318]
              tunnel: [w317] -> w308
              tunnel: w309 -> [w315] mode=indexing
              n115 = Copy(9:TRUE ("overwrite (F)"), 10:w318, 11:w315) -> (0:w317:errorcluster)  [unwired: 2 in, 2 out]
            }
            "Move to FM Error out" <- w308
          }
          frame #4 {
            n116 = local write "FTP ASCII Files to Local"(FALSE ("FTP Files to Local")) -> ()
          }
        }
      }
      event "Transfer OLD FGGA Files": Value Change {
        n117 = event-data() -> ()  [unwired: 1 in, 6 out]
        n118 = flat-sequence {
          tunnel: [w324] -> w323
          tunnel: w323 -> [w336]
          tunnel: [w336] -> w322
          tunnel: [w335] -> w321
          tunnel: [w334] -> w320
          tunnel: w322 -> [w346]
          tunnel: w321 -> [w345]
          tunnel: w320 -> [w347]
          frame #0 {
            n119 = local read "Flight Number"() -> (w325:string)
            n120 = Concatenate Strings("Confirm Flight Number" ("message"), "\n", w325) -> (w327:string)
            n121 = Two Button Dialog(message=w327, 1:"No" ("F button name (\"Cancel\")"), 2:"Yes" ("T button name (\"OK\")")) -> (T button?=w331:bool)
            n122 = case shown="False" w331 {
              tunnel: w325 -> [_ w333]
              tunnel: [w332 w333] -> w324
              frame False {
                n123 = call "Prompt User for Flight Number"() -> ("Flight Number CXXX"=w332:string)  [unwired: 17 in, 2 out]
              }
              frame True {
              }
            }
          }
          frame #1 {
            n124 = Two Button Dialog(message="Get FGGA Files\nof Today's Date?", 1:"No" ("F button name (\"Cancel\")"), 2:"Yes" ("T button name (\"OK\")")) -> (T button?=w340:bool)
            n125 = case shown="False" w340 {
              selector: w340 -> [w342 w343]
              tunnel: [w342 w343] -> w334
              tunnel: [w341 _] -> w335
              frame False {
                n126 = call "Prompt User for Date"() -> ("Date"=w341:string)  [unwired: 17 in, 2 out]
              }
              frame True {
              }
            }
          }
          frame #2 {
            n127 = Build Path(base path=path "\\\\192.168.101.180\\flt_folders" ("path"), name or relative path=w346) -> (appended path=w351:path)
            n128 = Concatenate Strings(w346, "_" ("string"), "corechem" ("string")) -> (w350:string)
            n129 = Build Path(base path=w351, name or relative path=w350) -> (appended path=w344:path)
            n130 = Create Folder(path (use dialog)=w344) -> (error out=→"Create folder error out":errorcluster)  [unwired: 2 in, 2 out]
            n131 = call "labSSH_FGGA_Files_Transfer.vi"("Flight_num"=w346, "Get current?"=w347, "Date"=w345, "Flight Folder Path"=w344) -> ("error IO"=→"FGGA File Transfer Error out":errorcluster)  [unwired: 11 in]
          }
          frame #3 {
            n132 = local write "Transfer OLD FGGA Files"(FALSE) -> ()
          }
        }
      }
      event "Transfer NEW FGGA Files": Value Change {
        n133 = event-data() -> ()  [unwired: 1 in, 6 out]
        n134 = flat-sequence {
          tunnel: [w360] -> w359
          tunnel: w359 -> [w372]
          tunnel: [w372] -> w358
          tunnel: [w371] -> w357
          tunnel: [w370] -> w356
          tunnel: w358 -> [w382]
          tunnel: w357 -> [w381]
          tunnel: w356 -> [w383]
          frame #0 {
            n135 = local read "Flight Number"() -> (w361:string)
            n136 = Concatenate Strings("Confirm Flight Number" ("message"), "\n", w361) -> (w363:string)
            n137 = Two Button Dialog(message=w363, 1:"No" ("F button name (\"Cancel\")"), 2:"Yes" ("T button name (\"OK\")")) -> (T button?=w367:bool)
            n138 = case shown="False" w367 {
              tunnel: w361 -> [_ w369]
              tunnel: [w368 w369] -> w360
              frame False {
                n139 = call "Prompt User for Flight Number3"() -> ("Flight Number CXXX"=w368:string)  [unwired: 17 in, 2 out]
              }
              frame True {
              }
            }
          }
          frame #1 {
            n140 = Two Button Dialog(message="Get FGGA Files\nof Today's Date?", 1:"No" ("F button name (\"Cancel\")"), 2:"Yes" ("T button name (\"OK\")")) -> (T button?=w376:bool)
            n141 = case shown="False" w376 {
              selector: w376 -> [w378 w379]
              tunnel: [w378 w379] -> w370
              tunnel: [w377 _] -> w371
              frame False {
                n142 = call "Prompt User for Date2"() -> ("Date"=w377:string)  [unwired: 17 in, 2 out]
              }
              frame True {
              }
            }
          }
          frame #2 {
            n143 = Build Path(base path=path "\\\\192.168.101.180\\flt_folders" ("path"), name or relative path=w382) -> (appended path=w387:path)
            n144 = Concatenate Strings(w382, "_" ("string"), "corechem" ("string")) -> (w386:string)
            n145 = Build Path(base path=w387, name or relative path=w386) -> (appended path=w380:path)
            n146 = Create Folder(path (use dialog)=w380) -> (error out=→"Create folder error out 3":errorcluster)  [unwired: 2 in, 2 out]
            n147 = call "labSSH_new_FGGA_Files_Transfer.vi"("Flight_num"=w382, "Get current?"=w383, "Date"=w381, "Flight Folder Path"=w380) -> ("error IO"=→"FGGA File Transfer Error out 2":errorcluster)  [unwired: 11 in]
          }
          frame #3 {
            n148 = local write "Transfer NEW FGGA Files"(FALSE) -> ()
          }
        }
      }
      event "OLD\nFGGA Restart": Value Change {
        n149 = event-data() -> ()  [unwired: 1 in, 6 out]
        n150 = flat-sequence {
          frame #0 {
            n151 = Two Button Dialog(message="FGGA will be restarted,\nARE YOU SURE?") -> (T button?=w393:bool)  [unwired: 2 in]
            n152 = case shown="True" w393 {
              frame False {
              }
              frame True {
                n153 = call "labSSH_Commands.vi"("Data"="reboot", "New_FGGA=T\nOld_FGGA=F"=FALSE ("New_FGGA=T\nOld_FGGA=F")) -> ()  [unwired: 13 in, 1 out]
              }
            }
          }
          frame #1 {
            n154 = local write "OLD\nFGGA Restart"(FALSE ("FGGA Restart")) -> ()
          }
        }
      }
      event "NEW\nFGGA Restart": Value Change {
        n155 = event-data() -> ()  [unwired: 1 in, 6 out]
        n156 = flat-sequence {
          frame #0 {
            n157 = Two Button Dialog(message="FGGA will be restarted,\nARE YOU SURE?") -> (T button?=w398:bool)  [unwired: 2 in]
            n158 = case shown="True" w398 {
              frame False {
              }
              frame True {
                n159 = call "labSSH_Commands.vi"("Data"="sudo -i reboot", "New_FGGA=T\nOld_FGGA=F"=TRUE ("New_FGGA=T\nOld_FGGA=F")) -> ()  [unwired: 13 in, 1 out]
              }
            }
          }
          frame #1 {
            n160 = local write "NEW\nFGGA Restart"(FALSE ("FGGA Restart")) -> ()
          }
        }
      }
      event "OLD FGGA Shutdown": Value Change {
        n161 = event-data() -> ()  [unwired: 1 in, 6 out]
        n162 = flat-sequence {
          frame #0 {
            n163 = Two Button Dialog(message="FGGA will be shutdown,\nARE YOU SURE?") -> (T button?=w403:bool)  [unwired: 2 in]
            n164 = case shown="True" w403 {
              frame False {
              }
              frame True {
                n165 = call "labSSH_Commands.vi"("Data"="halt", "New_FGGA=T\nOld_FGGA=F"=FALSE ("New_FGGA=T\nOld_FGGA=F")) -> ()  [unwired: 13 in, 1 out]
              }
            }
          }
          frame #1 {
            n166 = local write "OLD FGGA Shutdown"(FALSE ("FGGA Restart")) -> ()
          }
        }
      }
      event "NEW FGGA Shutdown": Value Change {
        n167 = event-data() -> ()  [unwired: 1 in, 6 out]
        n168 = flat-sequence {
          frame #0 {
            n169 = Two Button Dialog(message="FGGA will be shutdown,\nARE YOU SURE?") -> (T button?=w408:bool)  [unwired: 2 in]
            n170 = case shown="True" w408 {
              frame False {
              }
              frame True {
                n171 = call "labSSH_Commands.vi"("Data"="sudo -i halt", "New_FGGA=T\nOld_FGGA=F"=TRUE ("New_FGGA=T\nOld_FGGA=F")) -> ()  [unwired: 13 in, 1 out]
              }
            }
          }
          frame #1 {
            n172 = local write "NEW FGGA Shutdown"(FALSE ("FGGA Restart")) -> ()
          }
        }
      }
    }
    n173 = node-c288() -> ()  [unwired: 1 in, 1 out]
  }
  n174 = local write "Network disconnected"(FALSE ("Network disconnect")) -> ()
  n175 = while {
    shift-right: [w533] -> _
    shift-left: w11 -> [w531]
    shift-right: [w535] -> _
    shift-left: w10 -> [w536]
    shift-right: [w534] -> _
    shift-left: w12 -> [w538]
    shift-right: [w527] -> _
    shift-left: w12 -> [w529]
    shift-right: [w524] -> _
    shift-left: w11 -> [w523]
    shift-right: [w526] -> _
    shift-left: w10 -> [w528]
    stop <- FALSE stop-if-true
    w469 = ""
    w464 = "%s" ("format string")
    w655 = "%s" ("format string")
    w660 = "%s" ("format string")
    w665 = "%s" ("format string")
    w671 = "%s" ("format string")
    w677 = "%s" ("format string")
    w681 = "%s" ("format string")
    # "UDP Data Processing"
    n176 = local read "CHFGGA01"() -> (w684:string)
    n177 = local read "TWBOZO01"() -> (w659:string)
    n178 = local read "AL52CO01"() -> (w676:string)
    n179 = local read "CABOZO01"() -> (w664:string)
    n180 = local read "TEIOZO01"() -> (w670:string)
    n181 = local read "CHTSOO01"() -> (w654:string)
    n182 = local read "Ambient = OFF\nCabin = ON"() -> (w559:bool)
    n183 = Spreadsheet String To Array(delimiter (Tab)=",", format string=w681, spreadsheet string=w684, array type (2D Dbl)=string[] []) -> (array=w631:string[])
    n184 = Spreadsheet String To Array(delimiter (Tab)=",", format string=w677, spreadsheet string=w676, array type (2D Dbl)=string[] []) -> (array=w652:string[])
    n185 = Spreadsheet String To Array(delimiter (Tab)=",", format string=w665, spreadsheet string=w664, array type (2D Dbl)=string[] []) -> (array=w556:string[])
    n186 = Spreadsheet String To Array(delimiter (Tab)=",", format string=w671, spreadsheet string=w670, array type (2D Dbl)=string[] []) -> (array=w629:string[])
    n187 = Spreadsheet String To Array(delimiter (Tab)=",", format string=w660, spreadsheet string=w659, array type (2D Dbl)=string[] []) -> (array=w555:string[])
    n188 = Spreadsheet String To Array(delimiter (Tab)=",", format string=w655, spreadsheet string=w654, array type (2D Dbl)=string[] []) -> (array=w627:string[])
    n189 = Array To Spreadsheet String(delimiter (Tab)="\r", array=w631, 3:w681) -> (spreadsheet string=→"FGGA":string)
    n190 = Array To Spreadsheet String(delimiter (Tab)="\r", array=w652, 3:w677) -> (spreadsheet string=→"CO":string)
    n191 = Array To Spreadsheet String(delimiter (Tab)="\r", array=w556, 3:w665) -> (spreadsheet string=→"2B Cabin Ozone":string)
    n192 = Array To Spreadsheet String(delimiter (Tab)="\r", array=w629, 3:w671) -> (spreadsheet string=→"TEi49 Ozone":string)
    n193 = Array To Spreadsheet String(delimiter (Tab)="\r", array=w555, 3:w660) -> (spreadsheet string=→"2B Ambient Ozone":string)
    n194 = Array To Spreadsheet String(delimiter (Tab)="\r", array=w627, 3:w655) -> (spreadsheet string=→"SO2":string)
    n195 = Select(t=w556, s=w559, f=w555) -> (s? t:f=w554:string[])
    n196 = Index Array(array=w627, index #1=6 ("index"), index #2=4 ("index"), index #3=3 ("index"), index #4=7 ("index"), index #5=8 ("index"), index #6=15 ("index"), index #7=24 ("index"), index #8=29 ("index"), index #9=36 ("index"), index #10=37 ("index"), index #11=38 ("index"), index #12=39 ("index"), index #13=48 ("index"), index #14=14 ("index")) -> (element #1=w546:string, element #2=w610:string, element #3=w605:string, element #4=w598:string, element #5=w574:string, element #6=w573:string, element #7=w487:string, element #8=w486:string, element #9=w435:string, element #10=w431:string, element #11=w427:string, element #12=w425:string, element #13=w417:string, element #14=w415:string)
    n197 = Index Array(array=w554, index #1=8 ("index"), index #2=11 ("index")) -> (element #1=w548:string, element #2=w549:string)
    n198 = Index Array(array=w629, index #1=6 ("index"), index #2=4 ("index"), index #3=3 ("index"), index #4=7 ("index"), index #5=9 ("index"), index #6=14 ("index"), index #7=15 ("index")) -> (element #1=w623:string, element #2=w611:string, element #3=w606:string, element #4=w591:string, element #5=w565:string, element #6=w564:string, element #7=w563:string)
    n199 = Scan Value(string=w548, format string="%f") -> (value=→"2B Ozone concentration":dbl)  [unwired: 1 in, 1 out]
    n200 = Scan Value(string=w549, format string="%4f") -> (value=→"2B Ozone flow rate":dbl)  [unwired: 1 in, 1 out]
    n201 = Index Array(array=w631, index #1=6 ("index"), index #2=4 ("index"), index #3=3 ("index"), index #4=7 ("index"), index #5=8 ("index"), index #6=9 ("index"), index #7=10 ("index"), index #8=17 ("index"), index #9=16 ("index"), index #10=11 ("index"), index #11=12 ("index"), index #12=21 ("index"), index #13=14 ("index"), index #14=15 ("index")) -> (element #1=w625:string, element #2=w613:string, element #3=w608:string, element #4=w593:string, element #5=w511:string, element #6=w508:string, element #7=w503:string, element #8=w501:string, element #9=w498:string, element #10=w493:string, element #11=w492:string, element #12=w479:string, element #13=w445:string, element #14=w444:string)
    n202 = Index Array(array=w652, index #1=2 ("index"), index #2=27 ("index"), index #3=28 ("index"), index #4=29 ("index"), index #5=30 ("index"), index #6=31 ("index"), index #7=6 ("index"), index #8=4 ("index"), index #9=3 ("index"), index #10=8 ("index"), index #11=14 ("index"), index #12=16 ("index"), index #13=19 ("index"), index #14=12 ("index"), index #15=13 ("index"), index #16=10 ("index"), index #17=11 ("index"), index #18=15 ("index")) -> (element #1=w521:string, element #2=w595:string, element #3=w642:string, element #4=w636:string, element #5=w634:string, element #6=w635:string, element #7=w624:string, element #8=w612:string, element #9=w607:string, element #10=w596:string, element #11=w583:string, element #12=w580:string, element #13=w579:string, element #14=w541:string, element #15=w540:string, element #16=w475:string, element #17=w456:string, element #18=w450:string)
    n203 = Scan Value(string=w417, format string="%f") -> (value=→"Calibration gas cylinder \nconcentration (ppb)":dbl)  [unwired: 1 in, 1 out]
    n204 = Scan Value(string=w487, format string="%f") -> (value=→"TEI43i MFC2 Cal Flow":dbl)  [unwired: 1 in, 1 out]
    n205 = Scan Value(string=w486, format string="%f") -> (value=→"TEI43i MFC3 Sample Flow":dbl)  [unwired: 1 in, 1 out]
    n206 = Scan Value(string=w435, format string="%f") -> (value=w421:dbl)  [unwired: 1 in, 1 out]
    n207 = Scan Value(string=w431, format string="%d", default (0 dbl)=0) -> (value=w429:i32)  [unwired: 1 out]
    n208 = Scan Value(string=w415, format string="%f") -> (value=→"SO2 react pressure":dbl)  [unwired: 1 in, 1 out]
    n209 = Scan Value(string=w425, format string="%f") -> (value=→"SO2 Sensitivity":dbl)  [unwired: 1 in, 1 out]
    n210 = Scan Value(string=w427, format string="%f") -> (value=→"SO2 Zero":dbl)  [unwired: 1 in, 1 out]
    n211 = Scan Value(string=w574, format string="%f") -> (value=w422:dbl)  [unwired: 1 in, 1 out]
    n212 = Scan Value(string=w573, format string="%f") -> (value=→"TEI43C Sample Flow":dbl)  [unwired: 1 in, 1 out]
    n213 = Not Equal To 0?(x=w429) -> (x != 0?=→"mean zero\ncal status":bool)
    n214 = Decimal String To Number(string=w521) -> (number=w519:i32)  [unwired: 2 in, 1 out]
    n215 = call "Find_Data_SubVI.vi"("FGGA"=w625, "CO"=w624, "Ozone"=w623, "SO2"=w546) -> ("Output Value"=→"CPU Total %":dbl)  [unwired: 11 in]
    n216 = call "Find_Data_SubVI.vi"("FGGA"=w613, "CO"=w612, "Ozone"=w611, "SO2"=w610) -> ("Output Value"=→"MFM":dbl)  [unwired: 11 in]
    n217 = call "Find_Data_SubVI.vi"("FGGA"=w608, "CO"=w607, "Ozone"=w606, "SO2"=w605) -> ("Output Value"=w604:dbl)  [unwired: 11 in]
    n218 = call "Find_Data_SubVI.vi"("FGGA"=w593, "CO"=w596, "Ozone"=w591, "SO2"=w598) -> ("Output Value"=→"USB Disk Space Used %":dbl)  [unwired: 11 in]
    n219 = Not Equal To 0?(x=w604) -> (x != 0?=→"PTP Sync":bool)
    n220 = Add(x=w519, y=u32 2082844800) -> (x+y=w518:u32)
    n221 = Scan Value(string=w479, format string="%f") -> (value=→"MFC1 Cal Flow":dbl)  [unwired: 1 in, 1 out]
    n222 = Scan Value(string=w445, format string="%f") -> (value=w443:dbl)  [unwired: 1 in, 1 out]
    n223 = Scan Value(string=w444, format string="%f") -> (value=w441:dbl)  [unwired: 1 in, 1 out]
    n224 = Scan Value(string=w492, format string="%f") -> (value=→"Cell temperature":dbl)  [unwired: 1 in, 1 out]
    n225 = Scan Value(string=w493, format string="%f") -> (value=→"Cell pressure":dbl)  [unwired: 1 in, 1 out]
    n226 = Scan Value(string=w498, format string="%f") -> (value=→"CH4 Dry":dbl)  [unwired: 1 in, 1 out]
    n227 = Scan Value(string=w501, format string="%f") -> (value=→"CO2 Dry":dbl)  [unwired: 1 in, 1 out]
    n228 = Scan Value(string=w503, format string="%f") -> (value=→"H2O":dbl)  [unwired: 1 in, 1 out]
    n229 = Scan Value(string=w508, format string="%f") -> (value=→"CO2":dbl)  [unwired: 1 in, 1 out]
    n230 = Scan Value(string=w511, format string="%f") -> (value=→"CH4":dbl)  [unwired: 1 in, 1 out]
    n231 = local read "PRTAFT_UDP_In"() -> (w462:string)
    n232 = Scan Value(string=w635, format string="%f") -> (value=→"Std\nContent (barG)":dbl)  [unwired: 1 in, 1 out]
    n233 = Scan Value(string=w595, format string="%d", default (0 dbl)=u32 0) -> (value=w649:u32)  [unwired: 1 out]
    n234 = Scan Value(string=w634, format string="%f") -> (value=→"N2\nContent (barG)":dbl)  [unwired: 1 in, 1 out]
    n235 = Scan Value(string=w636, format string="%f") -> (value=→"CO2\nContent (barG)":dbl)  [unwired: 1 in, 1 out]
    n236 = Scan Value(string=w642, format string="%f") -> (value=→"CO2 Pressure\nDelivery (PSIA)":dbl)  [unwired: 1 in, 1 out]
    n237 = Bundle(w422, w421) -> (→"TEi43i Concentration scaled / raw":cluster{dbl, dbl})  [unwired: 1 in]
    n238 = To Time Stamp(1:w518) -> (0:w522:timestamp)
    n239 = Scan Value(string=w583, format string="%f") -> (value=→"Lamp Flow Controller":dbl)  [unwired: 1 in, 1 out]
    n240 = Scan Value(string=w456, format string="%f") -> (value=→"Raw Signal":dbl)  [unwired: 1 in, 1 out]
    n241 = Scan Value(string=w450, format string="%f") -> (value=→"Lamp Temperature":dbl)  [unwired: 1 in, 1 out]
    n242 = Scan Value(string=w475, format string="%f") -> (value=→"CO Concentration":dbl)  [unwired: 1 in, 1 out]
    n243 = Scan Value(string=w580, format string="%f") -> (value=→"Monochromator Flow":dbl)  [unwired: 1 in, 1 out]
    n244 = Scan Value(string=w579, format string="%f") -> (value=→"Fluorescence Cell Pressure":dbl)  [unwired: 1 in, 1 out]
    n245 = Not Equal To 0?(x=w649) -> (x != 0?=→"CO CAL Status":bool)
    n246 = Scan Value(string=w563, format string="%f") -> (value=→"TEI49 Sample Flow B":dbl)  [unwired: 1 in, 1 out]
    n247 = Scan Value(string=w565, format string="%f") -> (value=→"TEi49 Concentration":dbl)  [unwired: 1 in, 1 out]
    n248 = Scan Value(string=w564, format string="%f") -> (value=→"TEI49 Sample Flow A":dbl)  [unwired: 1 in, 1 out]
    n249 = Scan Value(string=w541, format string="%f") -> (value=w532:dbl)  [unwired: 1 in, 1 out]
    n250 = Scan Value(string=w540, format string="%f") -> (value=w525:dbl)  [unwired: 1 in, 1 out]
    n251 = Not Equal?(x=w531, y=w532) -> (x != y?=w537:bool)
    n252 = Not Equal?(x=w523, y=w525) -> (x != y?=w530:bool)
    n253 = Spreadsheet String To Array(delimiter (Tab)=",", format string=w464, spreadsheet string=w462, array type (2D Dbl)=string[] []) -> (array=w463:string[])
    n254 = case shown="True" w537 {
      tunnel: w538 -> [w705 w714]
      tunnel: w536 -> [w706 w713]
      tunnel: [w706 w712] -> w535
      tunnel: w522 -> [_ w708]
      tunnel: w532 -> [_ w709]
      tunnel: [w705 w711] -> w534
      tunnel: [w704 w710] -> w533
      tunnel: w532 -> [_ w710]
      tunnel: w531 -> [w704 _]
      frame False {
      }
      frame True {
        n255 = Bundle(w708, w709) -> (w707:cluster{timestamp, dbl})  [unwired: 1 in]
        n256 = Replace Array Subset(array=w714, new element=w707, index=w713) -> (w711:cluster{"time stamp":timestamp, "Y":dbl}[])
        n257 = Increment(x=w713) -> (x+1=w712:i32)
      }
    }
    "CO Sensitivity" <- w534
    n258 = case shown="True" w530 {
      tunnel: w529 -> [w694 w703]
      tunnel: w528 -> [w695 w702]
      tunnel: [w695 w701] -> w526
      tunnel: w522 -> [_ w700]
      tunnel: w525 -> [_ w699]
      tunnel: [w694 w698] -> w527
      tunnel: [w693 w697] -> w524
      tunnel: w525 -> [_ w697]
      tunnel: w523 -> [w693 _]
      frame False {
      }
      frame True {
        n259 = Bundle(w700, w699) -> (w696:cluster{timestamp, dbl})  [unwired: 1 in]
        n260 = Replace Array Subset(array=w703, new element=w696, index=w702) -> (w698:cluster{"time stamp":timestamp, "Y":dbl}[])
        n261 = Increment(x=w702) -> (x+1=w701:i32)
      }
    }
    "CO Zero" <- w527
    n262 = Array To Spreadsheet String(delimiter (Tab)="\r", array=w463, 3:w464) -> (spreadsheet string=→"PRTAFT_DLU":string)
    n263 = Index Array(array=w463, index #1=5 ("index"), index #2=19 ("index")) -> (element #1=w467:string, element #2=w465:string)
    n264 = Not Equal?(x=w467, y=w469) -> (x != y?=w468:bool)
    n265 = Not Equal?(x=w465, y=w469) -> (x != y?=w466:bool)
    n266 = Bundle(w443, w441) -> (→"Ring Down Time RDA & RDB":cluster{dbl, dbl})  [unwired: 1 in]
    n267 = case shown="False" w466 {
      tunnel: ["1" w690] -> w459
      tunnel: w465 -> [_ w690]
      frame False {
      }
      frame True {
      }
    }
    n268 = case shown="False" w468 {
      tunnel: ["XXXX" w692] -> w460
      tunnel: w467 -> [_ w692]
      frame False {
      }
      frame True {
      }
    }
    n269 = Wait (ms)(milliseconds to wait=u32 1000) -> ()  [unwired: 1 out]
    n270 = local write "WoW Flag"(w459) -> ()
    n271 = local write "Flight Number"(w460) -> ()
  }
  n272 = while {
    stop <- FALSE stop-if-true
    # "Check Connection with the cRIO continuously"
    n273 = node-c288() -> (w716:T6)  [unwired: 4 in]
    n274 = TCP Open Connection(address="192.168.101.17", remote port or service name=u16 7001) -> (connection ID=w725:refnum<k5>, error out=w726:errorcluster)  [unwired: 3 in]
    n275 = timed-loop {
      tunnel: w726 -> [w741]
      tunnel: w725 -> [w738]
      tunnel: [w734] -> w718
      tunnel: [w735] -> w722
      shift-right: [w730] -> _
      shift-left: FALSE -> [w731]
      timing: w716 -> [_]
      timing-out: [_] -> w715
      stop <- w734 stop-if-true
      # "Maintain live connecton to cRIO for connection watchdog"
      n276 = node-c288() -> ()  [unwired: 1 in, 1 out]
      n277 = TCP Write(connection ID=w738, data in="1", error in (no error)=w741, 9:2000 ("timeout ms (25000)")) -> (connection ID out=w739:refnum<k5>, bytes written=w736:i32, error out=w740:errorcluster)
      n278 = Select(t=FALSE, s=w731, f=TRUE) -> (s? t:f=w730:bool)
      "cRIO connection status" <- w730
      n279 = local write "Network disconnected"(FALSE ("Network disconnect")) -> ()
      n280 = TCP Read(connection ID=w739, bytes to read=w736, error in (no error)=w740, 9:2000 ("timeout ms (25000)")) -> (connection ID out=w735:refnum<k5>, error out=w734:errorcluster)  [unwired: 1 in, 1 out]
      n281 = node-c288() -> ()  [unwired: 1 in, 1 out]
    }
    n282 = node-c288(w715) -> ()  [unwired: 1 out]
    n283 = TCP Close Connection(connection ID=w722, error in (no error)=w718) -> (error out=w717:errorcluster)  [unwired: 1 in, 1 out]
    "Network Check error out" <- w717
    n284 = Unbundle By Name(w717) -> ("status"=w719:bool)
    "Network disconnected" <- w719
    n285 = case shown="True" w719 {
      frame False {
      }
      frame True {
        n286 = One Button Dialog(message="Connection to cRIO lost\nAll Calibration(s) will be terminated") -> ()  [unwired: 1 in, 1 out]
      }
    }
  }
  n287 = while {
    stop <- FALSE stop-if-true
    # "Preflight Sub VI Descriptions"
    n288 = Wait (ms)(milliseconds to wait=u32 500) -> ()  [unwired: 1 out]
    n289 = case shown="True" "Line Lock Setting Change" {
      frame False {
      }
      frame True {
        n290 = call "FGGA Linelock Settings Procedures.vi"() -> ()  [unwired: 12 in]
      }
    }
  }
  n291 = while {
    stop <- FALSE stop-if-true
    # "Postflight Sub VI Descriptions"
    n292 = case shown="True" "Postflight Procedures" {
      frame False {
      }
      frame True {
        n293 = call "PostFlight Procedures.vi"() -> ()  [unwired: 12 in]
      }
    }
    n294 = Wait (ms)(milliseconds to wait=u32 500) -> ()  [unwired: 1 out]
  }
  n295 = while {
    stop <- FALSE stop-if-true
    # "Preflight Sub VI Descriptions"
    n296 = case shown="True" "Prepare Gases" {
      frame False {
      }
      frame True {
        n297 = call "CO Gas Preparation.vi"() -> ()  [unwired: 12 in]
      }
    }
    n298 = Wait (ms)(milliseconds to wait=u32 500) -> ()  [unwired: 1 out]
  }
  n299 = while {
    stop <- FALSE stop-if-true
    # "Preflight Sub VI Descriptions"
    n300 = case shown="True" "Prepare SO2 Span Gas" {
      frame False {
      }
      frame True {
        n301 = call "SO2 Span Gas Preparation.vi"() -> ()  [unwired: 12 in]
      }
    }
    n302 = Wait (ms)(milliseconds to wait=u32 500) -> ()  [unwired: 1 out]
  }
  n303 = while {
    stop <- FALSE stop-if-true
    # "Preflight Sub VI Descriptions"
    n304 = case shown="True" "Prepare SO2 Zero Gas" {
      frame False {
      }
      frame True {
        n305 = call "SO2 ZeroAir Gas Preparation.vi"() -> ()  [unwired: 12 in]
      }
    }
    n306 = Wait (ms)(milliseconds to wait=u32 500) -> ()  [unwired: 1 out]
  }
  n307 = Obtain Queue(name (unnamed)="FGGA_Command", element data type=w56) -> (queue out=w6:refnum<queue>, error out=w5:errorcluster)  [unwired: 3 in, 1 out]
  n308 = while {
    stop <- FALSE stop-if-true
    # "Preflight Sub VI Descriptions"
    n309 = case shown="True" "CO Monitor Troubleshooting" {
      frame False {
      }
      frame True {
        n310 = call "CO Monitor Troubleshooting.vi"() -> ()  [unwired: 12 in]
      }
    }
    n311 = Wait (ms)(milliseconds to wait=u32 500) -> ()  [unwired: 1 out]
  }
  n312 = while {
    shift-right: [w768] -> _
    shift-left: u8 1 -> [w769]
    tunnel: w6 -> [w766]
    tunnel: w5 -> [w765]
    stop <- FALSE stop-if-true
    # "FGGA pump synchronise to WoW Wait on Wheel Flag"
    n313 = Wait (ms)(milliseconds to wait=u32 1000) -> ()  [unwired: 1 out]
    n314 = case shown="True" "FGGA pump\nsync to WoW" {
      tunnel: [w772 w777] -> w768
      tunnel: w769 -> [w772 w776]
      tunnel: w766 -> [_ w775]
      tunnel: w765 -> [_ w774]
      frame False {
      }
      frame True {
        n315 = local read "WoW Flag"() -> (w773:string)
        n316 = Scan Value(string=w773, format string="%d", default (0 dbl)=u8 0) -> (value=w777:u8)  [unwired: 1 out]
        n317 = Not Equal?(x=w777, y=w776) -> (x != y?=w780:bool)
        n318 = case shown="True" w780 {
          tunnel: w777 -> [_ w783]
          tunnel: w775 -> [_ w782]
          tunnel: w774 -> [_ w781]
          frame False {
          }
          frame True {
            n319 = Equal?(x=w783, y=u8 0) -> (x = y?=w788:bool)
            n320 = case shown="True" w788 {
              selector: w788 -> [w790 w791]
              tunnel: [w790 w791] -> w784
              frame False {
              }
              frame True {
              }
            }
            n321 = local write "Manual FGGA Pump"(w784) -> ()
            n322 = Bundle(cluster=T4 {"Message"="", "Message Data"=variant} ("Message Cluster"), "Message"="FGGA_pump", "Message Data"=w784) -> (w785:T4)
            n323 = Enqueue Element(queue=w782, element=w785, error in (no error)=w781) -> ()  [unwired: 1 in, 3 out]
          }
        }
      }
    }
  }
  n324 = while {
    tunnel: w6 -> [w793]
    tunnel: w5 -> [w792]
    tunnel: [w795] -> _
    tunnel: w16 -> [w794]
    stop <- FALSE stop-if-true
    # "FGGA UI Event Handler Loop"
    n325 = event shown="[9] \"Span Cal -  High Cal, CO Cal, Low Cal\": Value Change" {
      selector: _ -> [_ _ _ _ _ _ _ _ _ _ _ _ _ _ _ _ _]
      dyn-events: _ -> [_ _ _ _ _ _ _ _ _ _ _ _ _ _ _ _ _]
      timeout: _ -> [_ _ _ _ _ _ _ _ _ _ _ _ _ _ _ _ _]
      tunnel: w793 -> [w803 w807 w814 w821 w828 w836 w850 w857 w872 w1013 w1264 w1334 w1404 w1460 w1574 w1673 w1680]
      tunnel: w792 -> [w802 w806 w813 w820 w827 w835 w849 w856 w871 w1012 w1263 w1333 w1403 w1459 w1573 w1672 w1679]
      tunnel: [w797 w805 w812 w819 w826 w834 w848 w855 w862 w986 w1256 w1326 w1396 w1450 w1566 w1671 w1678] -> w795
      tunnel: w794 -> [_ _ _ _ _ _ _ _ _ w1000 _ _ _ _ _ _ _]
      event "eV1": Value Change {
        n326 = event-data() -> ("NewVal"=w800:bool)  [unwired: 1 in]
        n327 = Bundle(cluster=T4 {"Message"="", "Message Data"=variant} ("Message Cluster"), "Message"="V1", "Message Data"=w800) -> (w798:T4)
        n328 = Enqueue Element(queue=w803, element=w798, error in (no error)=w802) -> (error out=w797:errorcluster)  [unwired: 1 in, 2 out]
      }
      event "eV2": Value Change {
        n329 = event-data() -> ("NewVal"=w804:bool)  [unwired: 1 in]
        n330 = Bundle(cluster=T4 {"Message"="", "Message Data"=variant} ("Message Cluster"), "Message"="V2", "Message Data"=w804) -> (w808:T4)
        n331 = Enqueue Element(queue=w807, element=w808, error in (no error)=w806) -> (error out=w805:errorcluster)  [unwired: 1 in, 2 out]
      }
      event "eV3": Value Change {
        n332 = event-data() -> ("NewVal"=w811:bool)  [unwired: 1 in]
        n333 = Bundle(cluster=T4 {"Message"="", "Message Data"=variant} ("Message Cluster"), "Message"="V3", "Message Data"=w811) -> (w815:T4)
        n334 = Enqueue Element(queue=w814, element=w815, error in (no error)=w813) -> (error out=w812:errorcluster)  [unwired: 1 in, 2 out]
      }
      event "eV4": Value Change {
        n335 = event-data() -> ("NewVal"=w818:bool)  [unwired: 1 in]
        n336 = Bundle(cluster=T4 {"Message"="", "Message Data"=variant} ("Message Cluster"), "Message"="V4", "Message Data"=w818) -> (w822:T4)
        n337 = Enqueue Element(queue=w821, element=w822, error in (no error)=w820) -> (error out=w819:errorcluster)  [unwired: 1 in, 2 out]
      }
      event "Manual FGGA Pump": Value Change {
        n338 = event-data() -> ("NewVal"=w825:bool)  [unwired: 1 in]
        n339 = Bundle(cluster=T4 {"Message"="", "Message Data"=variant} ("Message Cluster"), "Message"="FGGA_pump", "Message Data"=w825) -> (w829:T4)
        n340 = Enqueue Element(queue=w828, element=w829, error in (no error)=w827) -> (error out=w826:errorcluster)  [unwired: 1 in, 2 out]
      }
      event "Confirm Flight Number": Value Change {
        n341 = event-data() -> ()  [unwired: 1 in, 6 out]
        n342 = flat-sequence {
          tunnel: w835 -> [w838]
          tunnel: w836 -> [w839]
          tunnel: [w839] -> w833
          tunnel: [w838] -> w832
          tunnel: [w841] -> w834
          tunnel: w833 -> [w843]
          tunnel: w832 -> [w842]
          frame #0 {
            n343 = local write "cRIO File IO Stop\n(USB Flash Drive Unmount)"(FALSE ("cRIO File IO Stop\n(USB Flash Drive Unmount)")) -> ()
          }
          frame #1 {
            n344 = local read "Flight Number"() -> (w840:string)
            n345 = Bundle(cluster=T4 {"Message"="", "Message Data"=variant} ("Message Cluster"), "Message"="Flight Number", "Message Data"=w840) -> (w844:T4)
            n346 = Enqueue Element(queue=w843, element=w844, error in (no error)=w842) -> (error out=w841:errorcluster)  [unwired: 1 in, 2 out]
          }
        }
      }
      event "OLD\nFGGA Restart": Value Change {
        n347 = event-data() -> ("NewVal"=w847:bool)  [unwired: 1 in]
        n348 = Bundle(cluster=T4 {"Message"="", "Message Data"=variant} ("Message Cluster"), "Message"="FGGA_restart", "Message Data"=w847) -> (w851:T4)
        n349 = Enqueue Element(queue=w850, element=w851, error in (no error)=w849) -> (error out=w848:errorcluster)  [unwired: 1 in, 2 out]
      }
      event "cRIO File IO Stop\n(USB Flash Drive Unmount)": Value Change {
        n350 = event-data() -> ("NewVal"=w854:bool)  [unwired: 1 in]
        n351 = Bundle(cluster=T4 {"Message"="", "Message Data"=variant} ("Message Cluster"), "Message"="Stop File Write", "Message Data"=w854) -> (w858:T4)
        n352 = Enqueue Element(queue=w857, element=w858, error in (no error)=w856) -> (error out=w855:errorcluster)  [unwired: 1 in, 2 out]
      }
      event "High Cal": Value Change {
        n353 = event-data() -> ()  [unwired: 1 in, 1 out]
        n354 = flat-sequence {
          tunnel: w872 -> [w877]
          tunnel: w871 -> [w876]
          tunnel: [w875] -> w870
          tunnel: [w874] -> w869
          tunnel: w870 -> [w893]
          tunnel: w869 -> [w892]
          tunnel: [w890] -> w868
          tunnel: [w889] -> w867
          tunnel: [w897] -> w866
          tunnel: [w898] -> w865
          tunnel: w867 -> [w902]
          tunnel: w868 -> [w901]
          tunnel: w866 -> [w955]
          tunnel: w865 -> [w954]
          tunnel: [w952] -> w864
          tunnel: [w951] -> w863
          tunnel: w864 -> [w969]
          tunnel: w863 -> [w968]
          tunnel: [w966] -> w861
          tunnel: [w974] -> w862
          tunnel: w861 -> [w974]
          frame #0 {
            w873 = TRUE
            n355 = Cluster To Array(cluster=T11 {"Message"="V2", "Message 2"="V3", "Message 3"="V4"}) -> (array=w878:string[])
            n356 = for {
              tunnel: w878 -> [w885] mode=indexing
              tunnel: w877 -> [w884]
              tunnel: w876 -> [w883]
              tunnel: [w882] -> w875
              tunnel: [w881] -> w874
              tunnel: w873 -> [w880]
              n357 = Bundle(cluster=T4 {"Message"="", "Message Data"=variant} ("Message Cluster"), "Message"=w885, "Message Data"=w880) -> (w887:T4)
              n358 = Enqueue Element(queue=w884, element=w887, error in (no error)=w883) -> (queue out=w882:refnum<queue>, error out=w881:errorcluster)  [unwired: 1 in, 1 out]
            }
            n359 = local write "eV2"(w873) -> ()
            n360 = local write "eV4"(w873) -> ()
            n361 = local write "eV3"(w873) -> ()
          }
          frame #1 {
            n362 = local read "MFC_1 User Set Value"() -> (w888:dbl)
            n363 = local write "MFC_1\nSLPM Value"(w888) -> ()
            n364 = Bundle(cluster=T4 {"Message"="", "Message Data"=variant} ("Message Cluster"), "Message"="MFC_1", "Message Data"=w888) -> (w891:T4)
            n365 = Enqueue Element(queue=w893, element=w891, error in (no error)=w892) -> (queue out=w890:refnum<queue>, error out=w889:errorcluster)  [unwired: 1 in, 1 out]
          }
          frame #2 {
            n366 = for {
              N: 45 -> [w945]
              tunnel: w902 -> [w935]
              tunnel: w901 -> [w936]
              tunnel: [w936] -> w900
              tunnel: [w935] -> w899
              tunnel: [w934] -> w896
              i -> [w944]
              stop <- w934 stop-if-true
              n367 = Subtract(x=w945, y=w944) -> (x-y=w943:i32)
              n368 = Decrement(x=w943) -> (x-1=w942:i32)
              n369 = local read "FGGA Calibration Abort"() -> (w939:bool)
              n370 = case shown="True" w939 {
                selector: w939 -> [w948 _]
                tunnel: [w948 w949] -> w937
                frame False {
                }
                frame True {
                  n371 = Two Button Dialog(message="Are you sure to abort FGGA High Cal?") -> (T button?=w949:bool)  [unwired: 2 in]
                }
              }
              n372 = Wait (ms)(milliseconds to wait=u32 1000) -> ()  [unwired: 1 out]
              n373 = local read "Network disconnected"() -> (w938:bool)
              n374 = Or(x=w938, y=w937) -> (x .or. y?=w934:bool)
              n375 = case shown="False" w937 {
                selector: w937 -> [w947 _]
                frame False {
                  n376 = local write "FGGA Calibration Abort"(w947) -> ()
                }
                frame True {
                }
              }
              n377 = Select(t=0, s=w934, f=w942) -> (s? t:f=→"High Cal\nFlush Time Remain (sec)":i32)
            }
            n378 = case shown="False" w896 {
              tunnel: w900 -> [w909 w933]
              tunnel: w899 -> [w908 w932]
              tunnel: [w905 w932] -> w898
              tunnel: [w904 w933] -> w897
              frame False {
                w910 = TRUE
                # "Carry on if connection to cRIO is made\nor calibration not abort"
                n379 = Bundle(cluster=T4 {"Message"="", "Message Data"=variant} ("Message Cluster"), "Message"="V1", "Message Data"=w910) -> (w911:T4)
                n380 = local write "eV1"(w910) -> ()
                n381 = Enqueue Element(queue=w909, element=w911, error in (no error)=w908) -> (queue out=w906:refnum<queue>, error out=w907:errorcluster)  [unwired: 1 in, 1 out]
                n382 = for {
                  N: 60 -> [w926]
                  tunnel: w907 -> [w916]
                  tunnel: w906 -> [w915]
                  tunnel: [w916] -> w905
                  tunnel: [w915] -> w904
                  i -> [w925]
                  stop <- w917 stop-if-true
                  n383 = local read "FGGA Calibration Abort"() -> (w920:bool)
                  n384 = Subtract(x=w926, y=w925) -> (x-y=w924:i32)
                  n385 = case shown="True" w920 {
                    selector: w920 -> [w929 _]
                    tunnel: [w929 w930] -> w918
                    frame False {
                    }
                    frame True {
                      n386 = Two Button Dialog(message="Are you sure to abort FGGA High Cal?") -> (T button?=w930:bool)  [unwired: 2 in]
                    }
                  }
                  n387 = local read "Network disconnected"() -> (w919:bool)
                  n388 = Wait (ms)(milliseconds to wait=u32 1000) -> ()  [unwired: 1 out]
                  n389 = Decrement(x=w924) -> (x-1=w921:i32)
                  n390 = Or(x=w919, y=w918) -> (x .or. y?=w917:bool)
                  n391 = case shown="False" w918 {
                    selector: w918 -> [w928 _]
                    frame False {
                      n392 = local write "FGGA Calibration Abort"(w928) -> ()
                    }
                    frame True {
                    }
                  }
                  n393 = Select(t=0, s=w917, f=w921) -> (s? t:f=→"High Cal\nCal Time Remain (sec)":i32)
                }
              }
              frame True {
              }
            }
          }
          frame #3 {
            w953 = FALSE
            n394 = Cluster To Array(cluster=T12 {"Message"="V2", "Message 2"="V3", "Message 3"="V4", "Message 4"="V1"}) -> (array=w956:string[])
            n395 = for {
              tunnel: w956 -> [w963] mode=indexing
              tunnel: [w962] -> w952
              tunnel: [w961] -> w951
              tunnel: w953 -> [w960]
              tunnel: w955 -> [w959]
              tunnel: w954 -> [w958]
              n396 = Bundle(cluster=T4 {"Message"="", "Message Data"=variant} ("Message Cluster"), "Message"=w963, "Message Data"=w960) -> (w965:T4)
              n397 = Enqueue Element(queue=w959, element=w965, error in (no error)=w958) -> (queue out=w962:refnum<queue>, error out=w961:errorcluster)  [unwired: 1 in, 1 out]
            }
            n398 = local write "eV2"(w953) -> ()
            n399 = local write "eV4"(w953) -> ()
            n400 = local write "eV3"(w953) -> ()
            n401 = local write "eV1"(w953) -> ()
          }
          frame #4 {
            w967 = 0.0 ("MFC_1\nSLPM Value")
            n402 = local write "MFC_1\nSLPM Value"(w967) -> ()
            n403 = Bundle(cluster=T4 {"Message"="", "Message Data"=variant} ("Message Cluster"), "Message"="MFC_1", "Message Data"=w967) -> (w971:T4)
            n404 = Enqueue Element(queue=w969, element=w971, error in (no error)=w968) -> (error out=w966:errorcluster)  [unwired: 1 in, 2 out]
          }
          frame #5 {
            w973 = FALSE ("High Cal")
            n405 = local write "High Cal"(w973) -> ()
            n406 = local write "FGGA Calibration Abort"(w973) -> ()
          }
        }
      }
      event "Span Cal - \nHigh Cal, CO Cal, Low Cal": Value Change {
        n407 = event-data() -> ()  [unwired: 1 in, 1 out]
        n408 = flat-sequence {
          tunnel: w1013 -> [w1019]
          tunnel: w1012 -> [w1018]
          tunnel: [w1017] -> w1011
          tunnel: [w1016] -> w1010
          tunnel: w1011 -> [w1035]
          tunnel: w1010 -> [w1034]
          tunnel: [w1032] -> w1008
          tunnel: [w1031] -> w1006
          tunnel: [w1041] -> w1009
          tunnel: w1008 -> [w1041]
          tunnel: [w1040] -> w1007
          tunnel: w1006 -> [w1040]
          tunnel: [w1038] -> w985
          tunnel: [w1038] -> w982
          tunnel: w1009 -> [w1059]
          tunnel: w1007 -> [w1060]
          tunnel: [w1060] -> w992
          tunnel: w1000 -> [w1061]
          tunnel: [w1061] -> w990
          tunnel: [w1059] -> w988
          tunnel: w985 -> [w1058]
          tunnel: [w1057] -> w983
          tunnel: w982 -> [w1057]
          tunnel: w992 -> [w1071]
          tunnel: [w1071] -> w991
          tunnel: w990 -> [w1070]
          tunnel: [w1070] -> w989
          tunnel: w988 -> [w1068]
          tunnel: [w1068] -> w987
          tunnel: [w1067] -> w984
          tunnel: w983 -> [w1067]
          tunnel: [w1075] -> w1005
          tunnel: [w1074] -> w1004
          tunnel: w987 -> [w1076]
          tunnel: w989 -> [w1082]
          tunnel: w991 -> [w1077]
          tunnel: w984 -> [w1073]
          tunnel: [w1073] -> w978
          tunnel: [w1072] -> w975
          tunnel: w1005 -> [w1121]
          tunnel: w1004 -> [w1120]
          tunnel: [w1118] -> w1003
          tunnel: [w1117] -> w1002
          tunnel: [w1116] -> w979
          tunnel: w978 -> [w1116]
          tunnel: [w1115] -> w976
          tunnel: w975 -> [w1115]
          tunnel: w1003 -> [w1138]
          tunnel: w1002 -> [w1137]
          tunnel: [w1135] -> w1001
          tunnel: [w1134] -> w997
          tunnel: [w1133] -> w980
          tunnel: w979 -> [w1133]
          tunnel: [w1132] -> w977
          tunnel: w976 -> [w1132]
          tunnel: w1001 -> [w1147]
          tunnel: [w1147] -> w999
          tunnel: [w1145] -> w998
          tunnel: w997 -> [w1145]
          tunnel: [w1144] -> w981
          tunnel: w980 -> [w1143]
          tunnel: w977 -> [w1142]
          tunnel: [w1152] -> w996
          tunnel: [w1151] -> w995
          tunnel: w999 -> [w1149]
          tunnel: w998 -> [w1150]
          tunnel: w981 -> [w1148]
          tunnel: w996 -> [w1234]
          tunnel: w995 -> [w1233]
          tunnel: [w1231] -> w994
          tunnel: [w1230] -> w993
          tunnel: w994 -> [w1249]
          tunnel: w993 -> [w1248]
          tunnel: [w1246] -> w986
          frame #0 {
            w1015 = TRUE
            n409 = Cluster To Array(cluster=T11 {"Message"="V2", "Message 2"="V3", "Message 3"="V4"}) -> (array=w1020:string[])
            n410 = for {
              tunnel: w1020 -> [w1027] mode=indexing
              tunnel: w1019 -> [w1026]
              tunnel: w1018 -> [w1025]
              tunnel: [w1024] -> w1017
              tunnel: [w1023] -> w1016
              tunnel: w1015 -> [w1022]
              n411 = Bundle(cluster=T4 {"Message"="", "Message Data"=variant} ("Message Cluster"), "Message"=w1027, "Message Data"=w1022) -> (w1029:T4)
              n412 = Enqueue Element(queue=w1026, element=w1029, error in (no error)=w1025) -> (queue out=w1024:refnum<queue>, error out=w1023:errorcluster)  [unwired: 1 in, 1 out]
            }
            n413 = local write "High Cal"(TRUE ("High Cal")) -> ()
            n414 = local write "eV2"(w1015) -> ()
            n415 = local write "eV4"(w1015) -> ()
            n416 = local write "eV3"(w1015) -> ()
          }
          frame #1 {
            n417 = local read "MFC_1 User Set Value"() -> (w1030:dbl)
            n418 = local write "MFC_1\nSLPM Value"(w1030) -> ()
            n419 = Bundle(cluster=T4 {"Message"="", "Message Data"=variant} ("Message Cluster"), "Message"="MFC_1", "Message Data"=w1030) -> (w1033:T4)
            n420 = Enqueue Element(queue=w1035, element=w1033, error in (no error)=w1034) -> (queue out=w1032:refnum<queue>, error out=w1031:errorcluster)  [unwired: 1 in, 1 out]
          }
          frame #2 {
            n421 = for {
              N: 45 -> [w1051]
              tunnel: [w1043] -> w1038
              i -> [w1050]
              stop <- w1043 stop-if-true
              n422 = local read "FGGA Calibration Abort"() -> (w1044:bool)
              n423 = case shown="True" w1044 {
                selector: w1044 -> [w1054 _]
                tunnel: [w1054 w1055] -> w1042
                frame False {
                }
                frame True {
                  n424 = Two Button Dialog(message="Are you sure to abort FGGA Span Cal?") -> (T button?=w1055:bool)  [unwired: 2 in]
                }
              }
              n425 = local read "Network disconnected"() -> (w1045:bool)
              n426 = Subtract(x=w1051, y=w1050) -> (x-y=w1049:i32)
              n427 = Decrement(x=w1049) -> (x-1=w1047:i32)
              n428 = Wait (ms)(milliseconds to wait=u32 1000) -> ()  [unwired: 1 out]
              n429 = Or(x=w1045, y=w1042) -> (x .or. y?=w1043:bool)
              n430 = case shown="False" w1042 {
                selector: w1042 -> [w1053 _]
                frame False {
                  n431 = local write "FGGA Calibration Abort"(w1053) -> ()
                }
                frame True {
                }
              }
              n432 = Select(t=0, s=w1043, f=w1047) -> (s? t:f=w1046:i32)
              n433 = local write "High Cal\nFlush Time Remain (sec)"(w1046) -> ()
            }
          }
          frame #3 {
            n434 = case shown="False" w1058 {
              tunnel: w1061 -> [w1062 _]
              frame False {
                # "CO Cal if no network\ndisconnect or abort cal"
                n435 = Bundle(cluster=T4 {"Message"="", "Message Data"=variant} ("Message Cluster"), "Message"="CO CAL", "Message Data"=TRUE) -> (w1064:T4)
                n436 = Enqueue Element(queue=w1062, element=w1064) -> ()  [unwired: 2 in, 3 out]
              }
              frame True {
              }
            }
          }
          frame #4 {
            # "To Ensure\nCO CAL\nis certain"
            n437 = Wait (ms)(milliseconds to wait=u32 1000) -> ()  [unwired: 1 out]
          }
          frame #5 {
            n438 = Bundle(cluster=T4 {"Message"="", "Message Data"=variant} ("Message Cluster"), "Message"="CO CAL", "Message Data"=FALSE) -> (w1078:T4)
            n439 = Enqueue Element(queue=w1082, element=w1078) -> ()  [unwired: 2 in, 3 out]
            n440 = case shown="False" w1073 {
              selector: w1073 -> [_ w1112]
              tunnel: w1077 -> [w1089 w1113]
              tunnel: w1076 -> [w1088 w1114]
              tunnel: [w1085 w1114] -> w1075
              tunnel: [w1084 w1113] -> w1074
              tunnel: [w1083 w1112] -> w1072
              frame False {
                w1093 = TRUE
                # "Carry on if connection to cRIO is made\nor calibration not abort"
                n441 = Bundle(cluster=T4 {"Message"="", "Message Data"=variant} ("Message Cluster"), "Message"="V1", "Message Data"=w1093) -> (w1092:T4)
                n442 = local write "eV1"(w1093) -> ()
                n443 = Enqueue Element(queue=w1088, element=w1092, error in (no error)=w1089) -> (queue out=w1087:refnum<queue>, error out=w1086:errorcluster)  [unwired: 1 in, 1 out]
                n444 = for {
                  N: 60 -> [w1106]
                  tunnel: w1087 -> [w1097]
                  tunnel: w1086 -> [w1096]
                  tunnel: [w1097] -> w1085
                  tunnel: [w1096] -> w1084
                  tunnel: [w1095] -> w1083
                  i -> [w1105]
                  stop <- w1095 stop-if-true
                  n445 = local read "FGGA Calibration Abort"() -> (w1100:bool)
                  n446 = case shown="True" w1100 {
                    selector: w1100 -> [w1109 _]
                    tunnel: [w1109 w1110] -> w1098
                    frame False {
                    }
                    frame True {
                      n447 = Two Button Dialog(message="Are you sure to abort FGGA Span Cal?") -> (T button?=w1110:bool)  [unwired: 2 in]
                    }
                  }
                  n448 = Subtract(x=w1106, y=w1105) -> (x-y=w1104:i32)
                  n449 = Decrement(x=w1104) -> (x-1=w1102:i32)
                  n450 = Wait (ms)(milliseconds to wait=u32 1000) -> ()  [unwired: 1 out]
                  n451 = local read "Network disconnected"() -> (w1099:bool)
                  n452 = Or(x=w1099, y=w1098) -> (x .or. y?=w1095:bool)
                  n453 = Select(t=0, s=w1095, f=w1102) -> (s? t:f=w1101:i32)
                  n454 = local write "High Cal\nCal Time Remain (sec)"(w1101) -> ()
                  n455 = case shown="False" w1098 {
                    selector: w1098 -> [w1108 _]
                    frame False {
                      n456 = local write "FGGA Calibration Abort"(w1108) -> ()
                    }
                    frame True {
                    }
                  }
                }
              }
              frame True {
              }
            }
          }
          frame #6 {
            w1119 = FALSE
            n457 = Cluster To Array(cluster=T12 {"Message"="V2", "Message 2"="V3", "Message 3"="V4", "Message 4"="V1"}) -> (array=w1122:string[])
            n458 = for {
              tunnel: w1122 -> [w1129] mode=indexing
              tunnel: [w1128] -> w1118
              tunnel: [w1127] -> w1117
              tunnel: w1119 -> [w1126]
              tunnel: w1121 -> [w1125]
              tunnel: w1120 -> [w1124]
              n459 = Bundle(cluster=T4 {"Message"="", "Message Data"=variant} ("Message Cluster"), "Message"=w1129, "Message Data"=w1126) -> (w1131:T4)
              n460 = Enqueue Element(queue=w1125, element=w1131, error in (no error)=w1124) -> (queue out=w1128:refnum<queue>, error out=w1127:errorcluster)  [unwired: 1 in, 1 out]
            }
            n461 = local write "eV2"(w1119) -> ()
            n462 = local write "eV4"(w1119) -> ()
            n463 = local write "eV3"(w1119) -> ()
            n464 = local write "eV1"(w1119) -> ()
          }
          frame #7 {
            w1136 = 0.0 ("MFC_1\nSLPM Value")
            n465 = local write "MFC_1\nSLPM Value"(w1136) -> ()
            n466 = Bundle(cluster=T4 {"Message"="", "Message Data"=variant} ("Message Cluster"), "Message"="MFC_1", "Message Data"=w1136) -> (w1140:T4)
            n467 = Enqueue Element(queue=w1138, element=w1140, error in (no error)=w1137) -> (queue out=w1134:refnum<queue>, error out=w1135:errorcluster)  [unwired: 1 in, 1 out]
          }
          frame #8 {
            n468 = local write "High Cal"(FALSE ("High Cal")) -> ()
            n469 = Or(x=w1143, y=w1142) -> (x .or. y?=w1144:bool)
          }
          frame #9 {
            n470 = case shown="False" w1148 {
              tunnel: [w1155 w1229] -> w1152
              tunnel: [w1154 w1228] -> w1151
              tunnel: w1150 -> [w1164 w1229]
              tunnel: w1149 -> [w1162 w1228]
              frame False {
                w1160 = TRUE
                n471 = Cluster To Array(cluster=cluster{"Message":string, "Message 3":string} {"Message"="V2", "Message 3"="V4"}) -> (array=w1165:string[])
                n472 = for {
                  tunnel: w1165 -> [w1208] mode=indexing
                  tunnel: w1164 -> [w1207]
                  tunnel: [w1206] -> w1166
                  tunnel: [w1205] -> w1168
                  tunnel: w1160 -> [w1204]
                  tunnel: w1162 -> [w1203]
                  n473 = Bundle(cluster=T4 {"Message"="", "Message Data"=variant} ("Message Cluster"), "Message"=w1208, "Message Data"=w1204) -> (w1210:T4)
                  n474 = Enqueue Element(queue=w1207, element=w1210, error in (no error)=w1203) -> (queue out=w1206:refnum<queue>, error out=w1205:errorcluster)  [unwired: 1 in, 1 out]
                }
                n475 = local write "eV4"(w1160) -> ()
                n476 = local write "eV2"(w1160) -> ()
                n477 = local write "Low Cal"(TRUE ("Low Cal")) -> ()
                n478 = local read "MFC_1 User Set Value"() -> (w1169:dbl)
                n479 = local write "MFC_1\nSLPM Value"(w1169) -> ()
                n480 = Bundle(cluster=T4 {"Message"="", "Message Data"=variant} ("Message Cluster"), "Message"="MFC_1", "Message Data"=w1169) -> (w1170:T4)
                n481 = Enqueue Element(queue=w1166, element=w1170, error in (no error)=w1168) -> (queue out=w1159:refnum<queue>, error out=w1157:errorcluster)  [unwired: 1 in, 1 out]
                n482 = for {
                  N: 45 -> [w1222]
                  tunnel: [w1213] -> w1158
                  tunnel: w1159 -> [w1213]
                  tunnel: [w1212] -> w1156
                  tunnel: w1157 -> [w1212]
                  tunnel: [w1211] -> w1153
                  i -> [w1221]
                  stop <- w1211 stop-if-true
                  n483 = local read "FGGA Calibration Abort"() -> (w1216:bool)
                  n484 = case shown="True" w1216 {
                    selector: w1216 -> [w1225 _]
                    tunnel: [w1225 w1226] -> w1214
                    frame False {
                    }
                    frame True {
                      n485 = Two Button Dialog(message="Are you sure to abort FGGA Span Cal?") -> (T button?=w1226:bool)  [unwired: 2 in]
                    }
                  }
                  n486 = Subtract(x=w1222, y=w1221) -> (x-y=w1220:i32)
                  n487 = Decrement(x=w1220) -> (x-1=w1217:i32)
                  n488 = Wait (ms)(milliseconds to wait=u32 1000) -> ()  [unwired: 1 out]
                  n489 = local read "Network disconnected"() -> (w1215:bool)
                  n490 = Or(x=w1215, y=w1214) -> (x .or. y?=w1211:bool)
                  n491 = Select(t=0, s=w1211, f=w1217) -> (s? t:f=w1218:i32)
                  n492 = local write "Low Cal\nFlush Time Remain (sec)"(w1218) -> ()
                  n493 = case shown="False" w1214 {
                    selector: w1214 -> [w1224 _]
                    frame False {
                      n494 = local write "FGGA Calibration Abort"(w1224) -> ()
                    }
                    frame True {
                    }
                  }
                }
                n495 = case shown="False" w1153 {
                  tunnel: w1158 -> [w1178 w1202]
                  tunnel: w1156 -> [w1177 w1201]
                  tunnel: [w1175 w1202] -> w1155
                  tunnel: [w1173 w1201] -> w1154
                  frame False {
                    w1179 = TRUE
                    n496 = local write "eV1"(w1179) -> ()
                    n497 = Bundle(cluster=T4 {"Message"="", "Message Data"=variant} ("Message Cluster"), "Message"="V1", "Message Data"=w1179) -> (w1181:T4)
                    n498 = Enqueue Element(queue=w1178, element=w1181, error in (no error)=w1177) -> (queue out=w1176:refnum<queue>, error out=w1174:errorcluster)  [unwired: 1 in, 1 out]
                    n499 = for {
                      N: 60 -> [w1195]
                      tunnel: [w1185] -> w1175
                      tunnel: w1176 -> [w1185]
                      tunnel: w1174 -> [w1184]
                      tunnel: [w1184] -> w1173
                      i -> [w1194]
                      stop <- w1186 stop-if-true
                      n500 = local read "FGGA Calibration Abort"() -> (w1189:bool)
                      n501 = case shown="True" w1189 {
                        selector: w1189 -> [w1198 _]
                        tunnel: [w1198 w1199] -> w1187
                        frame False {
                        }
                        frame True {
                          n502 = Two Button Dialog(message="Are you sure to abort FGGA Span Cal?") -> (T button?=w1199:bool)  [unwired: 2 in]
                        }
                      }
                      n503 = Wait (ms)(milliseconds to wait=u32 1000) -> ()  [unwired: 1 out]
                      n504 = local read "Network disconnected"() -> (w1188:bool)
                      n505 = Subtract(x=w1195, y=w1194) -> (x-y=w1193:i32)
                      n506 = Decrement(x=w1193) -> (x-1=w1190:i32)
                      n507 = Or(x=w1188, y=w1187) -> (x .or. y?=w1186:bool)
                      n508 = Select(t=0, s=w1186, f=w1190) -> (s? t:f=w1191:i32)
                      n509 = local write "Low Cal\nCal Time Remain (sec)"(w1191) -> ()
                      n510 = case shown="False" w1187 {
                        selector: w1187 -> [w1197 _]
                        frame False {
                          n511 = local write "FGGA Calibration Abort"(w1197) -> ()
                        }
                        frame True {
                        }
                      }
                    }
                  }
                  frame True {
                    # "Ignore Cal if connection problem or abort button pressed"
                  }
                }
              }
              frame True {
                # "Ignore Cal if connection problem or abort button pressed"
              }
            }
          }
          frame #10 {
            w1232 = FALSE
            n512 = Cluster To Array(cluster=T13 {"Message"="V2", "Message 3"="V4", "Message 4"="V1"}) -> (array=w1235:string[])
            n513 = local write "eV1"(w1232) -> ()
            n514 = local write "eV2"(w1232) -> ()
            n515 = local write "eV4"(w1232) -> ()
            n516 = for {
              tunnel: w1235 -> [w1242] mode=indexing
              tunnel: [w1241] -> w1231
              tunnel: [w1240] -> w1230
              tunnel: w1232 -> [w1239]
              tunnel: w1234 -> [w1238]
              tunnel: w1233 -> [w1237]
              n517 = Bundle(cluster=T4 {"Message"="", "Message Data"=variant} ("Message Cluster"), "Message"=w1242, "Message Data"=w1239) -> (w1244:T4)
              n518 = Enqueue Element(queue=w1238, element=w1244, error in (no error)=w1237) -> (queue out=w1241:refnum<queue>, error out=w1240:errorcluster)  [unwired: 1 in, 1 out]
            }
          }
          frame #11 {
            w1245 = FALSE
            w1247 = 0.0 ("MFC_1\nSLPM Value")
            n519 = local write "MFC_1\nSLPM Value"(w1247) -> ()
            n520 = local write "Span Cal - \nHigh Cal, CO Cal, Low Cal"(w1245) -> ()
            n521 = local write "FGGA Calibration Abort"(w1245) -> ()
            n522 = local write "Low Cal"(w1245) -> ()
            n523 = Bundle(cluster=T4 {"Message"="", "Message Data"=variant} ("Message Cluster"), "Message"="MFC_1", "Message Data"=w1247) -> (w1251:T4)
            n524 = Enqueue Element(queue=w1249, element=w1251, error in (no error)=w1248) -> (error out=w1246:errorcluster)  [unwired: 1 in, 2 out]
          }
        }
      }
      event "Flush High Tank": Value Change {
        n525 = event-data() -> ()  [unwired: 1 in, 6 out]
        n526 = flat-sequence {
          tunnel: w1264 -> [w1269]
          tunnel: w1263 -> [w1268]
          tunnel: [w1267] -> w1262
          tunnel: [w1266] -> w1261
          tunnel: w1262 -> [w1285]
          tunnel: w1261 -> [w1284]
          tunnel: [w1282] -> w1260
          tunnel: [w1281] -> w1259
          tunnel: w1260 -> [w1288]
          tunnel: w1259 -> [w1289]
          tunnel: [w1289] -> w1254
          tunnel: [w1288] -> w1253
          tunnel: [w1302] -> w1258
          tunnel: [w1301] -> w1257
          tunnel: w1254 -> [w1300]
          tunnel: w1253 -> [w1299]
          tunnel: w1258 -> [w1317]
          tunnel: w1257 -> [w1316]
          tunnel: [w1314] -> w1255
          tunnel: [w1322] -> w1256
          tunnel: w1255 -> [w1322]
          frame #0 {
            w1265 = TRUE
            n527 = Cluster To Array(cluster=T11 {"Message"="V2", "Message 2"="V3", "Message 3"="V4"}) -> (array=w1270:string[])
            n528 = for {
              tunnel: w1270 -> [w1277] mode=indexing
              tunnel: w1269 -> [w1276]
              tunnel: w1268 -> [w1275]
              tunnel: [w1274] -> w1267
              tunnel: [w1273] -> w1266
              tunnel: w1265 -> [w1272]
              n529 = Bundle(cluster=T4 {"Message"="", "Message Data"=variant} ("Message Cluster"), "Message"=w1277, "Message Data"=w1272) -> (w1279:T4)
              n530 = Enqueue Element(queue=w1276, element=w1279, error in (no error)=w1275) -> (queue out=w1274:refnum<queue>, error out=w1273:errorcluster)  [unwired: 1 in, 1 out]
            }
            n531 = local write "eV2"(w1265) -> ()
            n532 = local write "eV4"(w1265) -> ()
            n533 = local write "eV3"(w1265) -> ()
          }
          frame #1 {
            n534 = local read "MFC_1 User Set Value"() -> (w1280:dbl)
            n535 = local write "MFC_1\nSLPM Value"(w1280) -> ()
            n536 = Bundle(cluster=T4 {"Message"="", "Message Data"=variant} ("Message Cluster"), "Message"="MFC_1", "Message Data"=w1280) -> (w1283:T4)
            n537 = Enqueue Element(queue=w1285, element=w1283, error in (no error)=w1284) -> (queue out=w1282:refnum<queue>, error out=w1281:errorcluster)  [unwired: 1 in, 1 out]
          }
          frame #2 {
            n538 = for {
              N: 15 -> [w1297]
              i -> [w1296]
              stop <- w1292 stop-if-true
              n539 = Subtract(x=w1297, y=w1296) -> (x-y=w1295:i32)
              n540 = Decrement(x=w1295) -> (x-1=w1293:i32)
              n541 = local read "Network disconnected"() -> (w1292:bool)
              n542 = Wait (ms)(milliseconds to wait=u32 1000) -> ()  [unwired: 1 out]
              n543 = Select(t=0, s=w1292, f=w1293) -> (s? t:f=→"Flush High Tank\nTime Remain (sec)":i32)
            }
          }
          frame #3 {
            w1303 = FALSE
            n544 = Cluster To Array(cluster=T11 {"Message"="V2", "Message 2"="V3", "Message 3"="V4"}) -> (array=w1304:string[])
            n545 = for {
              tunnel: w1304 -> [w1311] mode=indexing
              tunnel: [w1310] -> w1302
              tunnel: [w1309] -> w1301
              tunnel: w1303 -> [w1308]
              tunnel: w1299 -> [w1307]
              tunnel: w1300 -> [w1306]
              n546 = Bundle(cluster=T4 {"Message"="", "Message Data"=variant} ("Message Cluster"), "Message"=w1311, "Message Data"=w1308) -> (w1313:T4)
              n547 = Enqueue Element(queue=w1307, element=w1313, error in (no error)=w1306) -> (queue out=w1310:refnum<queue>, error out=w1309:errorcluster)  [unwired: 1 in, 1 out]
            }
            n548 = local write "eV2"(w1303) -> ()
            n549 = local write "eV4"(w1303) -> ()
            n550 = local write "eV3"(w1303) -> ()
          }
          frame #4 {
            w1315 = 0.0 ("MFC_1\nSLPM Value")
            n551 = local write "MFC_1\nSLPM Value"(w1315) -> ()
            n552 = Bundle(cluster=T4 {"Message"="", "Message Data"=variant} ("Message Cluster"), "Message"="MFC_1", "Message Data"=w1315) -> (w1319:T4)
            n553 = Enqueue Element(queue=w1317, element=w1319, error in (no error)=w1316) -> (error out=w1314:errorcluster)  [unwired: 1 in, 2 out]
          }
          frame #5 {
            n554 = local write "Flush High Tank"(FALSE ("High Cal")) -> ()
          }
        }
      }
      event "Flush Low Tank": Value Change {
        n555 = event-data() -> ()  [unwired: 1 in, 1 out]
        n556 = flat-sequence {
          tunnel: w1334 -> [w1339]
          tunnel: w1333 -> [w1338]
          tunnel: [w1337] -> w1332
          tunnel: [w1336] -> w1331
          tunnel: w1332 -> [w1355]
          tunnel: w1331 -> [w1354]
          tunnel: [w1352] -> w1330
          tunnel: [w1351] -> w1329
          tunnel: w1330 -> [w1358]
          tunnel: w1329 -> [w1359]
          tunnel: [w1359] -> w1324
          tunnel: [w1358] -> w1323
          tunnel: [w1372] -> w1328
          tunnel: [w1371] -> w1327
          tunnel: w1324 -> [w1370]
          tunnel: w1323 -> [w1369]
          tunnel: w1328 -> [w1387]
          tunnel: w1327 -> [w1386]
          tunnel: [w1384] -> w1325
          tunnel: [w1392] -> w1326
          tunnel: w1325 -> [w1392]
          frame #0 {
            w1335 = TRUE
            n557 = Cluster To Array(cluster=cluster{"Message":string, "Message 3":string} {"Message"="V2", "Message 3"="V4"}) -> (array=w1340:string[])
            n558 = for {
              tunnel: w1340 -> [w1347] mode=indexing
              tunnel: w1339 -> [w1346]
              tunnel: w1338 -> [w1345]
              tunnel: [w1344] -> w1337
              tunnel: [w1343] -> w1336
              tunnel: w1335 -> [w1342]
              n559 = Bundle(cluster=T4 {"Message"="", "Message Data"=variant} ("Message Cluster"), "Message"=w1347, "Message Data"=w1342) -> (w1349:T4)
              n560 = Enqueue Element(queue=w1346, element=w1349, error in (no error)=w1345) -> (queue out=w1344:refnum<queue>, error out=w1343:errorcluster)  [unwired: 1 in, 1 out]
            }
            n561 = local write "eV2"(w1335) -> ()
            n562 = local write "eV4"(w1335) -> ()
          }
          frame #1 {
            n563 = local read "MFC_1 User Set Value"() -> (w1350:dbl)
            n564 = local write "MFC_1\nSLPM Value"(w1350) -> ()
            n565 = Bundle(cluster=T4 {"Message"="", "Message Data"=variant} ("Message Cluster"), "Message"="MFC_1", "Message Data"=w1350) -> (w1353:T4)
            n566 = Enqueue Element(queue=w1355, element=w1353, error in (no error)=w1354) -> (queue out=w1352:refnum<queue>, error out=w1351:errorcluster)  [unwired: 1 in, 1 out]
          }
          frame #2 {
            n567 = for {
              N: 15 -> [w1367]
              i -> [w1366]
              stop <- w1361 stop-if-true
              n568 = Subtract(x=w1367, y=w1366) -> (x-y=w1365:i32)
              n569 = Decrement(x=w1365) -> (x-1=w1362:i32)
              n570 = local read "Network disconnected"() -> (w1361:bool)
              n571 = Wait (ms)(milliseconds to wait=u32 1000) -> ()  [unwired: 1 out]
              n572 = Select(t=0, s=w1361, f=w1362) -> (s? t:f=→"Flush Low Tank\nTime Remain (sec)":i32)
            }
          }
          frame #3 {
            w1373 = FALSE
            n573 = Cluster To Array(cluster=cluster{"Message":string, "Message 3":string} {"Message"="V2", "Message 3"="V4"}) -> (array=w1374:string[])
            n574 = for {
              tunnel: w1374 -> [w1381] mode=indexing
              tunnel: [w1380] -> w1372
              tunnel: [w1379] -> w1371
              tunnel: w1373 -> [w1378]
              tunnel: w1369 -> [w1377]
              tunnel: w1370 -> [w1376]
              n575 = Bundle(cluster=T4 {"Message"="", "Message Data"=variant} ("Message Cluster"), "Message"=w1381, "Message Data"=w1378) -> (w1383:T4)
              n576 = Enqueue Element(queue=w1377, element=w1383, error in (no error)=w1376) -> (queue out=w1380:refnum<queue>, error out=w1379:errorcluster)  [unwired: 1 in, 1 out]
            }
            n577 = local write "eV2"(w1373) -> ()
            n578 = local write "eV4"(w1373) -> ()
          }
          frame #4 {
            w1385 = 0.0 ("MFC_1\nSLPM Value")
            n579 = local write "MFC_1\nSLPM Value"(w1385) -> ()
            n580 = Bundle(cluster=T4 {"Message"="", "Message Data"=variant} ("Message Cluster"), "Message"="MFC_1", "Message Data"=w1385) -> (w1389:T4)
            n581 = Enqueue Element(queue=w1387, element=w1389, error in (no error)=w1386) -> (error out=w1384:errorcluster)  [unwired: 1 in, 2 out]
          }
          frame #5 {
            n582 = local write "Flush Low Tank"(FALSE ("High Cal")) -> ()
          }
        }
      }
      event "Flush Target Tank": Value Change {
        n583 = event-data() -> ()  [unwired: 1 in, 1 out]
        n584 = flat-sequence {
          tunnel: w1404 -> [w1412]
          tunnel: w1403 -> [w1411]
          tunnel: [w1410] -> w1402
          tunnel: [w1409] -> w1401
          tunnel: w1402 -> [w1418]
          tunnel: w1401 -> [w1417]
          tunnel: [w1415] -> w1400
          tunnel: [w1414] -> w1399
          tunnel: w1400 -> [w1421]
          tunnel: w1399 -> [w1422]
          tunnel: [w1422] -> w1394
          tunnel: [w1421] -> w1393
          tunnel: [w1438] -> w1398
          tunnel: [w1437] -> w1397
          tunnel: w1394 -> [w1436]
          tunnel: w1393 -> [w1435]
          tunnel: w1398 -> [w1443]
          tunnel: w1397 -> [w1442]
          tunnel: [w1440] -> w1395
          tunnel: [w1448] -> w1396
          tunnel: w1395 -> [w1448]
          frame #0 {
            w1408 = TRUE
            n585 = local write "eV4"(w1408) -> ()
            n586 = Bundle(cluster=T4 {"Message"="", "Message Data"=variant} ("Message Cluster"), "Message"="V4" ("Message 3"), "Message Data"=w1408) -> (w1407:T4)
            n587 = Enqueue Element(queue=w1412, element=w1407, error in (no error)=w1411) -> (queue out=w1410:refnum<queue>, error out=w1409:errorcluster)  [unwired: 1 in, 1 out]
          }
          frame #1 {
            n588 = local read "MFC_1 User Set Value"() -> (w1413:dbl)
            n589 = local write "MFC_1\nSLPM Value"(w1413) -> ()
            n590 = Bundle(cluster=T4 {"Message"="", "Message Data"=variant} ("Message Cluster"), "Message"="MFC_1", "Message Data"=w1413) -> (w1416:T4)
            n591 = Enqueue Element(queue=w1418, element=w1416, error in (no error)=w1417) -> (queue out=w1415:refnum<queue>, error out=w1414:errorcluster)  [unwired: 1 in, 1 out]
          }
          frame #2 {
            n592 = for {
              N: 15 -> [w1430]
              i -> [w1429]
              stop <- w1425 stop-if-true
              n593 = Subtract(x=w1430, y=w1429) -> (x-y=w1428:i32)
              n594 = Decrement(x=w1428) -> (x-1=w1426:i32)
              n595 = Wait (ms)(milliseconds to wait=u32 1000) -> ()  [unwired: 1 out]
              n596 = local read "Network disconnected"() -> (w1425:bool)
              n597 = Select(t=0, s=w1425, f=w1426) -> (s? t:f=→"Flush Target Tank\nTime Remain (sec)":i32)
            }
          }
          frame #3 {
            w1439 = FALSE
            n598 = Bundle(cluster=T4 {"Message"="", "Message Data"=variant} ("Message Cluster"), "Message"="V4" ("Message 3"), "Message Data"=w1439) -> (w1434:T4)
            n599 = local write "eV4"(w1439) -> ()
            n600 = Enqueue Element(queue=w1435, element=w1434, error in (no error)=w1436) -> (queue out=w1438:refnum<queue>, error out=w1437:errorcluster)  [unwired: 1 in, 1 out]
          }
          frame #4 {
            w1441 = 0.0 ("MFC_1\nSLPM Value")
            n601 = local write "MFC_1\nSLPM Value"(w1441) -> ()
            n602 = Bundle(cluster=T4 {"Message"="", "Message Data"=variant} ("Message Cluster"), "Message"="MFC_1", "Message Data"=w1441) -> (w1445:T4)
            n603 = Enqueue Element(queue=w1443, element=w1445, error in (no error)=w1442) -> (error out=w1440:errorcluster)  [unwired: 1 in, 2 out]
          }
          frame #5 {
            n604 = local write "Flush Target Tank"(FALSE ("High Cal")) -> ()
          }
        }
      }
      event "Low Cal": Value Change {
        n605 = event-data() -> ()  [unwired: 1 in, 1 out]
        n606 = flat-sequence {
          tunnel: w1460 -> [w1465]
          tunnel: w1459 -> [w1464]
          tunnel: [w1463] -> w1458
          tunnel: [w1462] -> w1457
          tunnel: w1458 -> [w1481]
          tunnel: w1457 -> [w1480]
          tunnel: [w1478] -> w1456
          tunnel: [w1477] -> w1455
          tunnel: [w1486] -> w1454
          tunnel: [w1485] -> w1453
          tunnel: w1455 -> [w1489]
          tunnel: w1456 -> [w1490]
          tunnel: w1454 -> [w1543]
          tunnel: w1453 -> [w1542]
          tunnel: [w1540] -> w1452
          tunnel: [w1539] -> w1451
          tunnel: w1452 -> [w1557]
          tunnel: w1451 -> [w1556]
          tunnel: [w1554] -> w1449
          tunnel: [w1562] -> w1450
          tunnel: w1449 -> [w1562]
          frame #0 {
            w1461 = TRUE
            n607 = Cluster To Array(cluster=cluster{"Message":string, "Message 3":string} {"Message"="V2", "Message 3"="V4"}) -> (array=w1466:string[])
            n608 = for {
              tunnel: w1466 -> [w1473] mode=indexing
              tunnel: w1465 -> [w1472]
              tunnel: w1464 -> [w1471]
              tunnel: [w1470] -> w1463
              tunnel: [w1469] -> w1462
              tunnel: w1461 -> [w1468]
              n609 = Bundle(cluster=T4 {"Message"="", "Message Data"=variant} ("Message Cluster"), "Message"=w1473, "Message Data"=w1468) -> (w1475:T4)
              n610 = Enqueue Element(queue=w1472, element=w1475, error in (no error)=w1471) -> (queue out=w1470:refnum<queue>, error out=w1469:errorcluster)  [unwired: 1 in, 1 out]
            }
            n611 = local write "eV2"(w1461) -> ()
            n612 = local write "eV4"(w1461) -> ()
          }
          frame #1 {
            n613 = local read "MFC_1 User Set Value"() -> (w1476:dbl)
            n614 = local write "MFC_1\nSLPM Value"(w1476) -> ()
            n615 = Bundle(cluster=T4 {"Message"="", "Message Data"=variant} ("Message Cluster"), "Message"="MFC_1", "Message Data"=w1476) -> (w1479:T4)
            n616 = Enqueue Element(queue=w1481, element=w1479, error in (no error)=w1480) -> (queue out=w1478:refnum<queue>, error out=w1477:errorcluster)  [unwired: 1 in, 1 out]
          }
          frame #2 {
            n617 = for {
              N: 45 -> [w1533]
              tunnel: w1490 -> [w1524]
              tunnel: w1489 -> [w1523]
              tunnel: [w1524] -> w1488
              tunnel: [w1523] -> w1487
              tunnel: [w1522] -> w1484
              i -> [w1532]
              stop <- w1522 stop-if-true
              n618 = local read "FGGA Calibration Abort"() -> (w1527:bool)
              n619 = case shown="True" w1527 {
                selector: w1527 -> [w1536 _]
                tunnel: [w1536 w1537] -> w1525
                frame False {
                }
                frame True {
                  n620 = Two Button Dialog(message="Are you sure to abort FGGA Low Cal?") -> (T button?=w1537:bool)  [unwired: 2 in]
                }
              }
              n621 = local read "Network disconnected"() -> (w1526:bool)
              n622 = Subtract(x=w1533, y=w1532) -> (x-y=w1531:i32)
              n623 = Decrement(x=w1531) -> (x-1=w1529:i32)
              n624 = Wait (ms)(milliseconds to wait=u32 1000) -> ()  [unwired: 1 out]
              n625 = Or(x=w1526, y=w1525) -> (x .or. y?=w1522:bool)
              n626 = case shown="False" w1525 {
                selector: w1525 -> [w1535 _]
                frame False {
                  n627 = local write "FGGA Calibration Abort"(w1535) -> ()
                }
                frame True {
                }
              }
              n628 = Select(t=0, s=w1522, f=w1529) -> (s? t:f=→"Low Cal\nFlush Time Remain (sec)":i32)
            }
            n629 = case shown="False" w1484 {
              tunnel: w1488 -> [w1497 w1521]
              tunnel: w1487 -> [w1496 w1520]
              tunnel: [w1494 w1521] -> w1486
              tunnel: [w1492 w1520] -> w1485
              frame False {
                w1498 = TRUE
                # "Carry on if connection to cRIO is made\nor calibration not abort"
                n630 = Bundle(cluster=T4 {"Message"="", "Message Data"=variant} ("Message Cluster"), "Message"="V1", "Message Data"=w1498) -> (w1499:T4)
                n631 = local write "eV1"(w1498) -> ()
                n632 = Enqueue Element(queue=w1497, element=w1499, error in (no error)=w1496) -> (queue out=w1495:refnum<queue>, error out=w1493:errorcluster)  [unwired: 1 in, 1 out]
                n633 = for {
                  N: 60 -> [w1514]
                  tunnel: w1495 -> [w1504]
                  tunnel: [w1504] -> w1494
                  tunnel: w1493 -> [w1503]
                  tunnel: [w1503] -> w1492
                  i -> [w1513]
                  stop <- w1505 stop-if-true
                  n634 = Subtract(x=w1514, y=w1513) -> (x-y=w1512:i32)
                  n635 = local read "FGGA Calibration Abort"() -> (w1507:bool)
                  n636 = case shown="True" w1507 {
                    selector: w1507 -> [w1517 _]
                    tunnel: [w1517 w1518] -> w1506
                    frame False {
                    }
                    frame True {
                      n637 = Two Button Dialog(message="Are you sure to abort FGGA Low Cal?") -> (T button?=w1518:bool)  [unwired: 2 in]
                    }
                  }
                  n638 = Decrement(x=w1512) -> (x-1=w1509:i32)
                  n639 = local read "Network disconnected"() -> (w1508:bool)
                  n640 = Wait (ms)(milliseconds to wait=u32 1000) -> ()  [unwired: 1 out]
                  n641 = Or(x=w1508, y=w1506) -> (x .or. y?=w1505:bool)
                  n642 = case shown="False" w1506 {
                    selector: w1506 -> [w1516 _]
                    frame False {
                      n643 = local write "FGGA Calibration Abort"(w1516) -> ()
                    }
                    frame True {
                    }
                  }
                  n644 = Select(t=0, s=w1505, f=w1509) -> (s? t:f=→"Low Cal\nCal Time Remain (sec)":i32)
                }
              }
              frame True {
              }
            }
          }
          frame #3 {
            w1541 = FALSE
            n645 = Cluster To Array(cluster=T13 {"Message"="V2", "Message 3"="V4", "Message 4"="V1"}) -> (array=w1544:string[])
            n646 = for {
              tunnel: w1544 -> [w1551] mode=indexing
              tunnel: [w1550] -> w1540
              tunnel: [w1549] -> w1539
              tunnel: w1541 -> [w1548]
              tunnel: w1543 -> [w1547]
              tunnel: w1542 -> [w1546]
              n647 = Bundle(cluster=T4 {"Message"="", "Message Data"=variant} ("Message Cluster"), "Message"=w1551, "Message Data"=w1548) -> (w1553:T4)
              n648 = Enqueue Element(queue=w1547, element=w1553, error in (no error)=w1546) -> (queue out=w1550:refnum<queue>, error out=w1549:errorcluster)  [unwired: 1 in, 1 out]
            }
            n649 = local write "eV2"(w1541) -> ()
            n650 = local write "eV4"(w1541) -> ()
            n651 = local write "eV1"(w1541) -> ()
          }
          frame #4 {
            w1555 = 0.0 ("MFC_1\nSLPM Value")
            n652 = local write "MFC_1\nSLPM Value"(w1555) -> ()
            n653 = Bundle(cluster=T4 {"Message"="", "Message Data"=variant} ("Message Cluster"), "Message"="MFC_1", "Message Data"=w1555) -> (w1559:T4)
            n654 = Enqueue Element(queue=w1557, element=w1559, error in (no error)=w1556) -> (error out=w1554:errorcluster)  [unwired: 1 in, 2 out]
          }
          frame #5 {
            w1561 = FALSE ("High Cal")
            n655 = local write "Low Cal"(w1561) -> ()
            n656 = local write "FGGA Calibration Abort"(w1561) -> ()
          }
        }
      }
      event "Target Cal": Value Change {
        n657 = event-data() -> ()  [unwired: 1 in, 1 out]
        n658 = flat-sequence {
          tunnel: w1574 -> [w1582]
          tunnel: w1573 -> [w1581]
          tunnel: [w1580] -> w1572
          tunnel: [w1579] -> w1571
          tunnel: w1572 -> [w1588]
          tunnel: w1571 -> [w1587]
          tunnel: [w1585] -> w1570
          tunnel: [w1584] -> w1569
          tunnel: w1569 -> [w1595]
          tunnel: w1570 -> [w1596]
          tunnel: [w1593] -> w1564
          tunnel: [w1592] -> w1563
          tunnel: [w1648] -> w1568
          tunnel: [w1649] -> w1567
          tunnel: w1564 -> [w1647]
          tunnel: w1563 -> [w1646]
          tunnel: w1568 -> [w1664]
          tunnel: w1567 -> [w1663]
          tunnel: [w1661] -> w1565
          tunnel: [w1669] -> w1566
          tunnel: w1565 -> [w1669]
          frame #0 {
            w1578 = TRUE
            n659 = local write "eV4"(w1578) -> ()
            n660 = Bundle(cluster=T4 {"Message"="", "Message Data"=variant} ("Message Cluster"), "Message"="V4" ("Message 3"), "Message Data"=w1578) -> (w1577:T4)
            n661 = Enqueue Element(queue=w1582, element=w1577, error in (no error)=w1581) -> (queue out=w1580:refnum<queue>, error out=w1579:errorcluster)  [unwired: 1 in, 1 out]
          }
          frame #1 {
            n662 = local read "MFC_1 User Set Value"() -> (w1583:dbl)
            n663 = local write "MFC_1\nSLPM Value"(w1583) -> ()
            n664 = Bundle(cluster=T4 {"Message"="", "Message Data"=variant} ("Message Cluster"), "Message"="MFC_1", "Message Data"=w1583) -> (w1586:T4)
            n665 = Enqueue Element(queue=w1588, element=w1586, error in (no error)=w1587) -> (queue out=w1585:refnum<queue>, error out=w1584:errorcluster)  [unwired: 1 in, 1 out]
          }
          frame #2 {
            n666 = for {
              N: 45 -> [w1640]
              tunnel: [w1631] -> w1597
              tunnel: w1596 -> [w1631]
              tunnel: [w1630] -> w1594
              tunnel: w1595 -> [w1630]
              tunnel: [w1629] -> w1591
              i -> [w1639]
              stop <- w1629 stop-if-true
              n667 = Subtract(x=w1640, y=w1639) -> (x-y=w1638:i32)
              n668 = Decrement(x=w1638) -> (x-1=w1635:i32)
              n669 = local read "FGGA Calibration Abort"() -> (w1634:bool)
              n670 = local read "Network disconnected"() -> (w1633:bool)
              n671 = case shown="True" w1634 {
                selector: w1634 -> [w1643 _]
                tunnel: [w1643 w1644] -> w1632
                frame False {
                }
                frame True {
                  n672 = Two Button Dialog(message="Are you sure to abort FGGA Target Cal?") -> (T button?=w1644:bool)  [unwired: 2 in]
                }
              }
              n673 = Wait (ms)(milliseconds to wait=u32 1000) -> ()  [unwired: 1 out]
              n674 = Or(x=w1633, y=w1632) -> (x .or. y?=w1629:bool)
              n675 = case shown="False" w1632 {
                selector: w1632 -> [w1642 _]
                frame False {
                  n676 = local write "FGGA Calibration Abort"(w1642) -> ()
                }
                frame True {
                }
              }
              n677 = Select(t=0, s=w1629, f=w1635) -> (s? t:f=→"Target Cal\nFlush Time Remain (sec)":i32)
            }
            n678 = case shown="False" w1591 {
              tunnel: w1597 -> [w1604 w1628]
              tunnel: w1594 -> [w1603 w1627]
              tunnel: [w1600 w1628] -> w1593
              tunnel: [w1599 w1627] -> w1592
              frame False {
                w1605 = TRUE
                # "Carry on if connection to cRIO is made\nor calibration not abort"
                n679 = Bundle(cluster=T4 {"Message"="", "Message Data"=variant} ("Message Cluster"), "Message"="V1", "Message Data"=w1605) -> (w1606:T4)
                n680 = local write "eV1"(w1605) -> ()
                n681 = Enqueue Element(queue=w1604, element=w1606, error in (no error)=w1603) -> (queue out=w1602:refnum<queue>, error out=w1601:errorcluster)  [unwired: 1 in, 1 out]
                n682 = for {
                  N: 60 -> [w1621]
                  tunnel: w1602 -> [w1611]
                  tunnel: w1601 -> [w1610]
                  tunnel: [w1611] -> w1600
                  tunnel: [w1610] -> w1599
                  i -> [w1620]
                  stop <- w1612 stop-if-true
                  n683 = Subtract(x=w1621, y=w1620) -> (x-y=w1619:i32)
                  n684 = Decrement(x=w1619) -> (x-1=w1617:i32)
                  n685 = local read "FGGA Calibration Abort"() -> (w1615:bool)
                  n686 = case shown="True" w1615 {
                    selector: w1615 -> [w1624 _]
                    tunnel: [w1624 w1625] -> w1613
                    frame False {
                    }
                    frame True {
                      n687 = Two Button Dialog(message="Are you sure to abort FGGA Target Cal?") -> (T button?=w1625:bool)  [unwired: 2 in]
                    }
                  }
                  n688 = Wait (ms)(milliseconds to wait=u32 1000) -> ()  [unwired: 1 out]
                  n689 = local read "Network disconnected"() -> (w1614:bool)
                  n690 = Or(x=w1614, y=w1613) -> (x .or. y?=w1612:bool)
                  n691 = case shown="False" w1613 {
                    selector: w1613 -> [w1623 _]
                    frame False {
                      n692 = local write "FGGA Calibration Abort"(w1623) -> ()
                    }
                    frame True {
                    }
                  }
                  n693 = Select(t=0, s=w1612, f=w1617) -> (s? t:f=→"Target Cal\nCal Time Remain (sec)":i32)
                }
              }
              frame True {
              }
            }
          }
          frame #3 {
            w1652 = FALSE
            n694 = Cluster To Array(cluster=cluster{"Message 3":string, "Message":string} {"Message 3"="V4", "Message"="V1"}) -> (array=w1650:string[])
            n695 = for {
              tunnel: w1650 -> [w1658] mode=indexing
              tunnel: [w1657] -> w1648
              tunnel: [w1656] -> w1649
              tunnel: w1652 -> [w1655]
              tunnel: w1647 -> [w1654]
              tunnel: w1646 -> [w1653]
              n696 = Bundle(cluster=T4 {"Message"="", "Message Data"=variant} ("Message Cluster"), "Message"=w1658, "Message Data"=w1655) -> (w1660:T4)
              n697 = Enqueue Element(queue=w1654, element=w1660, error in (no error)=w1653) -> (queue out=w1657:refnum<queue>, error out=w1656:errorcluster)  [unwired: 1 in, 1 out]
            }
            n698 = local write "eV4"(w1652) -> ()
            n699 = local write "eV1"(w1652) -> ()
          }
          frame #4 {
            w1662 = 0.0 ("MFC_1\nSLPM Value")
            n700 = local write "MFC_1\nSLPM Value"(w1662) -> ()
            n701 = Bundle(cluster=T4 {"Message"="", "Message Data"=variant} ("Message Cluster"), "Message"="MFC_1", "Message Data"=w1662) -> (w1666:T4)
            n702 = Enqueue Element(queue=w1664, element=w1666, error in (no error)=w1663) -> (error out=w1661:errorcluster)  [unwired: 1 in, 2 out]
          }
          frame #5 {
            w1668 = FALSE ("High Cal")
            n703 = local write "Target Cal"(w1668) -> ()
            n704 = local write "FGGA Calibration Abort"(w1668) -> ()
          }
        }
      }
      event "MFC_1\nSLPM Value": Value Change {
        n705 = event-data() -> ()  [unwired: 1 in, 1 out]
        n706 = local read "MFC_1\nSLPM Value"() -> (w1670:dbl)
        n707 = Bundle(cluster=T4 {"Message"="", "Message Data"=variant} ("Message Cluster"), "Message"="MFC_1", "Message Data"=w1670) -> (w1674:T4)
        n708 = Enqueue Element(queue=w1673, element=w1674, error in (no error)=w1672) -> (error out=w1671:errorcluster)  [unwired: 1 in, 2 out]
      }
      event "FGGA UDP Time Offset": Value Change {
        n709 = event-data() -> ("NewVal"=w1677:i32)  [unwired: 1 in, 5 out]
        n710 = Bundle(cluster=T4 {"Message"="", "Message Data"=variant} ("Message Cluster"), "Message"="UDP Time Offset", "Message Data"=w1677) -> (w1681:T4)
        n711 = Enqueue Element(queue=w1680, element=w1681, error in (no error)=w1679) -> (error out=w1678:errorcluster)  [unwired: 1 in, 2 out]
      }
    }
    "FGGA Event Error out" <- w795
  }
  n712 = node-c288(w14) -> ()  [unwired: 1 out]
  n713 = Create Network Stream Writer Endpoint(6:w54, 7:10 ("writer buffer size"), 9:w56, 10:"//192.168.101.17/command/reader/FGGA" ("reader url"), 11:"/command/writer/FGGA" ("writer name")) -> (0:w53:errorcluster, 3:w52:refnum<k21>)  [unwired: 2 in]
  n714 = while {
    tunnel: w6 -> [w1691]
    shift-right: [w1686] -> _
    shift-left: w52 -> [w1688]
    shift-right: [w1684] -> w49
    shift-left: w53 -> [w1690]
    tunnel: w5 -> [w1685]
    stop <- w1684 stop-if-true
    # "FGGA UI Command Sender"
    n715 = Dequeue Element(queue=w1691, error in (no error)=w1685) -> (element=w1687:T4)  [unwired: 1 in, 3 out]
    n716 = Unbundle By Name(w1687) -> ("Message"=w1689:string)
    n717 = case shown="\"UDP Time Offset\"" w1689 {
      tunnel: w1690 -> [w1692 w1696 w1703 w1710 w1717 w1724 w1731 w1738 w1745 w1752 w1759]
      tunnel: w1688 -> [w1693 w1699 w1706 w1713 w1720 w1727 w1734 w1741 w1748 w1755 w1762]
      tunnel: w1687 -> [_ w1698 w1705 w1712 w1719 w1726 w1733 w1740 w1747 w1754 w1761]
      tunnel: [w1692 w1695 w1702 w1709 w1716 w1723 w1730 w1737 w1744 w1751 w1758] -> w1684
      tunnel: [w1693 w1694 w1701 w1708 w1715 w1722 w1729 w1736 w1743 w1750 w1757] -> w1686
      frame "False", Default {
      }
      frame "V1" {
        n718 = shared-variable-write(w1699, w1696, w1698) -> (w1697:refnum<k21>, w1700:errorcluster)  [unwired: 1 in, 1 out]
        n719 = Flush Stream(8:w1700, 11:w1697) -> (0:w1695:errorcluster, 3:w1694:refnum<k21>)  [unwired: 2 in, 1 out]
      }
      frame "MFC_1" {
        n720 = shared-variable-write(w1706, w1703, w1705) -> (w1704:refnum<k21>, w1707:errorcluster)  [unwired: 1 in, 1 out]
        n721 = Flush Stream(8:w1707, 11:w1704) -> (0:w1702:errorcluster, 3:w1701:refnum<k21>)  [unwired: 2 in, 1 out]
      }
      frame "UDP Time Offset" {
        n722 = shared-variable-write(w1713, w1710, w1712) -> (w1711:refnum<k21>, w1714:errorcluster)  [unwired: 1 in, 1 out]
        n723 = Flush Stream(8:w1714, 11:w1711) -> (0:w1709:errorcluster, 3:w1708:refnum<k21>)  [unwired: 2 in, 1 out]
      }
      frame "V2" {
        n724 = shared-variable-write(w1720, w1717, w1719) -> (w1718:refnum<k21>, w1721:errorcluster)  [unwired: 1 in, 1 out]
        n725 = Flush Stream(8:w1721, 11:w1718) -> (0:w1716:errorcluster, 3:w1715:refnum<k21>)  [unwired: 2 in, 1 out]
      }
      frame "V3" {
        n726 = shared-variable-write(w1727, w1724, w1726) -> (w1725:refnum<k21>, w1728:errorcluster)  [unwired: 1 in, 1 out]
        n727 = Flush Stream(8:w1728, 11:w1725) -> (0:w1723:errorcluster, 3:w1722:refnum<k21>)  [unwired: 2 in, 1 out]
      }
      frame "V4" {
        n728 = shared-variable-write(w1734, w1731, w1733) -> (w1732:refnum<k21>, w1735:errorcluster)  [unwired: 1 in, 1 out]
        n729 = Flush Stream(8:w1735, 11:w1732) -> (0:w1730:errorcluster, 3:w1729:refnum<k21>)  [unwired: 2 in, 1 out]
      }
      frame "FGGA_pump" {
        n730 = shared-variable-write(w1741, w1738, w1740) -> (w1739:refnum<k21>, w1742:errorcluster)  [unwired: 1 in, 1 out]
        n731 = Flush Stream(8:w1742, 11:w1739) -> (0:w1737:errorcluster, 3:w1736:refnum<k21>)  [unwired: 2 in, 1 out]
      }
      frame "Flight Number" {
        n732 = shared-variable-write(w1748, w1745, w1747) -> (w1746:refnum<k21>, w1749:errorcluster)  [unwired: 1 in, 1 out]
        n733 = Flush Stream(8:w1749, 11:w1746) -> (0:w1744:errorcluster, 3:w1743:refnum<k21>)  [unwired: 2 in, 1 out]
      }
      frame "FGGA_restart" {
        n734 = shared-variable-write(w1755, w1752, w1754) -> (w1753:refnum<k21>, w1756:errorcluster)  [unwired: 1 in, 1 out]
        n735 = Flush Stream(8:w1756, 11:w1753) -> (0:w1751:errorcluster, 3:w1750:refnum<k21>)  [unwired: 2 in, 1 out]
      }
      frame "Stop File Write" {
        n736 = shared-variable-write(w1762, w1759, w1761) -> (w1760:refnum<k21>, w1763:errorcluster)  [unwired: 1 in, 1 out]
        n737 = Flush Stream(8:w1763, 11:w1760) -> (0:w1758:errorcluster, 3:w1757:refnum<k21>)  [unwired: 2 in, 1 out]
      }
    }
  }
  "FGGA command sender error out" <- w49
  n738 = local write "FGGA Calibration Abort"(FALSE ("FGGA Calibration Abort")) -> ()
  n739 = Obtain Queue(name (unnamed)="SO2_Command", element data type=w40) -> (queue out=w4:refnum<queue>, error out=w3:errorcluster)  [unwired: 3 in, 1 out]
  n740 = while {
    tunnel: w4 -> [w1767]
    tunnel: w3 -> [w1766]
    tunnel: [w1764] -> _
    stop <- FALSE stop-if-true
    # "SO2 UI Event Handler Loop"
    n741 = event shown="[7] \"SO2 Zero Calibration\": Value Change" {
      selector: _ -> [_ _ _ _ _ _ _ _ _ _ _ _ _ _ _ _ _ _ _ _ _ _ _ _ _ _ _ _ _ _]
      dyn-events: _ -> [_ _ _ _ _ _ _ _ _ _ _ _ _ _ _ _ _ _ _ _ _ _ _ _ _ _ _ _ _ _]
      timeout: _ -> [_ _ _ _ _ _ _ _ _ _ _ _ _ _ _ _ _ _ _ _ _ _ _ _ _ _ _ _ _ _]
      tunnel: w1767 -> [w1774 w1786 w1833 w1844 w1887 w1922 w2033 w2181 w2307 w2313 w2324 w2327 w2335 w2341 w2348 w2354 w2360 w2370 w2374 w2381 w2388 w2395 w2402 w2409 w2416 w2423 w2430 w2437 w2445 w2459]
      tunnel: w1766 -> [w1773 w1785 w1832 w1843 w1886 w1921 w2032 w2180 w2306 w2312 w2323 w2326 w2333 w2340 w2347 w2353 w2359 w2369 w2373 w2380 w2387 w2394 w2401 w2408 w2415 w2422 w2429 w2436 w2444 w2458]
      tunnel: [w1768 w1784 _ w1842 w1885 _ _ _ _ _ w2318 w2325 w2332 _ w2346 _ _ w2364 w2372 w2379 w2386 w2393 w2400 w2407 w2414 w2421 w2428 w2435 w2443 w2457] -> w1764
      event "eV9": Value Change {
        n742 = event-data() -> ("NewVal"=w1771:bool)  [unwired: 1 in]
        n743 = Bundle(cluster=T4 {"Message"="", "Message Data"=variant} ("Message Cluster"), "Message"="V9", "Message Data"=w1771) -> (w1769:T4)
        n744 = Enqueue Element(queue=w1774, element=w1769, error in (no error)=w1773) -> (error out=w1768:errorcluster)  [unwired: 1 in, 2 out]
      }
      event "SO2 Flush": Value Change {
        n745 = event-data() -> ()  [unwired: 1 in, 1 out]
        n746 = flat-sequence {
          tunnel: w1786 -> [w1794]
          tunnel: w1785 -> [w1793]
          tunnel: [w1789] -> w1781
          tunnel: [w1787] -> w1779
          tunnel: w1781 -> [w1796]
          tunnel: [w1798] -> w1780
          tunnel: w1779 -> [w1797]
          tunnel: [w1799] -> w1778
          tunnel: w1780 -> [w1805]
          tunnel: [w1805] -> w1783
          tunnel: [w1803] -> w1782
          tunnel: w1778 -> [w1803]
          tunnel: w1783 -> [w1817]
          tunnel: [w1816] -> w1777
          tunnel: w1782 -> [w1818]
          tunnel: [w1814] -> w1775
          tunnel: w1777 -> [w1824]
          tunnel: [w1825] -> w1776
          tunnel: w1775 -> [w1823]
          tunnel: [w1830] -> w1784
          tunnel: w1776 -> [w1830]
          frame #0 {
            w1788 = TRUE ("SO2 Flush")
            n747 = Bundle(cluster=T4 {"Message"="", "Message Data"=variant} ("Message Cluster"), "Message"="V9", "Message Data"=w1788) -> (w1790:T4)
            n748 = local write "eV9"(w1788) -> ()
            n749 = Enqueue Element(queue=w1794, element=w1790, error in (no error)=w1793) -> (queue out=w1787:refnum<queue>, error out=w1789:errorcluster)  [unwired: 1 in, 1 out]
          }
          frame #1 {
            n750 = local read "MFC_2 User Set Value"() -> (w1795:dbl)
            n751 = local write "MFC_2\nSLPM Value"(w1795) -> ()
            n752 = Bundle(cluster=T4 {"Message"="", "Message Data"=variant} ("Message Cluster"), "Message"="MFC_2", "Message Data"=w1795) -> (w1800:T4)
            n753 = Enqueue Element(queue=w1797, element=w1800, error in (no error)=w1796) -> (queue out=w1799:refnum<queue>, error out=w1798:errorcluster)  [unwired: 1 in, 1 out]
          }
          frame #2 {
            n754 = for {
              N: "eV9 Flush User\nset time (sec)" -> [w1812]
              i -> [w1811]
              stop <- w1806 stop-if-true
              n755 = local read "Network disconnected"() -> (w1806:bool)
              n756 = Subtract(x=w1812, y=w1811) -> (x-y=w1810:i32)
              n757 = Decrement(x=w1810) -> (x-1=w1808:i32)
              n758 = Wait (ms)(milliseconds to wait=u32 1000) -> ()  [unwired: 1 out]
              n759 = Select(t=0, s=w1806, f=w1808) -> (s? t:f=w1807:i32)
              n760 = local write "SO2 Flush\nTime Remain (sec)"(w1807) -> ()
            }
          }
          frame #3 {
            w1815 = FALSE
            n761 = Bundle(cluster=T4 {"Message"="", "Message Data"=variant} ("Message Cluster"), "Message"="V9", "Message Data"=w1815) -> (w1819:T4)
            n762 = local write "eV9"(w1815) -> ()
            n763 = Enqueue Element(queue=w1818, element=w1819, error in (no error)=w1817) -> (queue out=w1814:refnum<queue>, error out=w1816:errorcluster)  [unwired: 1 in, 1 out]
          }
          frame #4 {
            w1822 = 0.0 ("MFC_2\nSLPM Value")
            n764 = local write "MFC_2\nSLPM Value"(w1822) -> ()
            n765 = Bundle(cluster=T4 {"Message"="", "Message Data"=variant} ("Message Cluster"), "Message"="MFC_2", "Message Data"=w1822) -> (w1826:T4)
            n766 = Enqueue Element(queue=w1823, element=w1826, error in (no error)=w1824) -> (error out=w1825:errorcluster)  [unwired: 1 in, 2 out]
          }
          frame #5 {
            n767 = local write "SO2 Flush"(FALSE ("SO2 Flush")) -> ()
          }
        }
      }
      event "Auto Zeroing \ninterval (sec)": Value Change {
        n768 = event-data() -> ("NewVal"=w1831:i32)  [unwired: 1 in]
        n769 = Bundle(cluster=T4 {"Message"="", "Message Data"=variant} ("Message Cluster"), "Message"="zeroing_interval", "Message Data"=w1831) -> (w1834:T4)
        n770 = Enqueue Element(queue=w1833, element=w1834, error in (no error)=w1832) -> ()  [unwired: 1 in, 3 out]
      }
      event "SO2 GND Zeroing": Value Change {
        n771 = event-data() -> ()  [unwired: 1 in, 1 out]
        n772 = flat-sequence {
          tunnel: w1844 -> [w1852]
          tunnel: w1843 -> [w1851]
          tunnel: [w1847] -> w1841
          tunnel: [w1845] -> w1837
          tunnel: w1841 -> [w1855]
          tunnel: [w1855] -> w1840
          tunnel: [w1854] -> w1838
          tunnel: w1837 -> [w1854]
          tunnel: w1840 -> [w1873]
          tunnel: [w1872] -> w1839
          tunnel: w1838 -> [w1874]
          tunnel: [w1879] -> w1842
          tunnel: w1839 -> [w1879]
          frame #0 {
            w1846 = TRUE ("SO2 Flush")
            n773 = local write "SO2 eV6"(w1846) -> ()
            n774 = Bundle(cluster=T4 {"Message"="", "Message Data"=variant} ("Message Cluster"), "Message"="V6", "Message Data"=w1846) -> (w1848:T4)
            n775 = Enqueue Element(queue=w1852, element=w1848, error in (no error)=w1851) -> (queue out=w1845:refnum<queue>, error out=w1847:errorcluster)  [unwired: 1 in, 1 out]
          }
          frame #1 {
            # "10 Mins Count down"
            n776 = for {
              N: "eV6 User\nset time (sec)" -> [w1865]
              i -> [w1864]
              stop <- w1856 stop-if-true
              n777 = local read "SO2 Calibration Abort"() -> (w1862:bool)
              n778 = case shown="True" w1862 {
                selector: w1862 -> [w1868 _]
                tunnel: [w1868 w1869] -> w1857
                frame False {
                }
                frame True {
                  n779 = Two Button Dialog(message="Are you sure to abort SO2 Zeroing?") -> (T button?=w1869:bool)  [unwired: 2 in]
                }
              }
              n780 = Subtract(x=w1865, y=w1864) -> (x-y=w1863:i32)
              n781 = Decrement(x=w1863) -> (x-1=w1859:i32)
              n782 = Wait (ms)(milliseconds to wait=u32 1000) -> ()  [unwired: 1 out]
              n783 = local read "Network disconnected"() -> (w1860:bool)
              n784 = Or(x=w1860, y=w1857) -> (x .or. y?=w1856:bool)
              n785 = case shown="False" w1857 {
                selector: w1857 -> [w1867 _]
                frame False {
                  n786 = local write "SO2 Calibration Abort"(w1867) -> ()
                }
                frame True {
                }
              }
              n787 = Select(t=0, s=w1856, f=w1859) -> (s? t:f=w1858:i32)
              n788 = local write "SO2 Zeroing\nTime Remain (sec)"(w1858) -> ()
            }
          }
          frame #2 {
            w1871 = FALSE
            n789 = Bundle(cluster=T4 {"Message"="", "Message Data"=variant} ("Message Cluster"), "Message"="V6", "Message Data"=w1871) -> (w1875:T4)
            n790 = local write "SO2 eV6"(w1871) -> ()
            n791 = Enqueue Element(queue=w1874, element=w1875, error in (no error)=w1873) -> (error out=w1872:errorcluster)  [unwired: 1 in, 2 out]
          }
          frame #3 {
            n792 = local write "SO2 GND Zeroing"(FALSE ("SO2 Flush")) -> ()
          }
        }
      }
      event "SO2 Inflight \nZeroing": Value Change {
        n793 = event-data() -> ()  [unwired: 1 in, 1 out]
        n794 = flat-sequence {
          tunnel: w1887 -> [w1895]
          tunnel: w1886 -> [w1894]
          tunnel: [w1890] -> w1884
          tunnel: [w1888] -> w1880
          tunnel: w1884 -> [w1898]
          tunnel: [w1898] -> w1883
          tunnel: [w1897] -> w1881
          tunnel: w1880 -> [w1897]
          tunnel: w1883 -> [w1906]
          tunnel: [w1905] -> w1882
          tunnel: w1881 -> [w1907]
          tunnel: [w1912] -> w1885
          tunnel: w1882 -> [w1912]
          frame #0 {
            w1889 = TRUE ("SO2 Flush")
            n795 = local write "SO2 eV6"(w1889) -> ()
            n796 = Bundle(cluster=T4 {"Message"="", "Message Data"=variant} ("Message Cluster"), "Message"="V6", "Message Data"=w1889) -> (w1891:T4)
            n797 = Enqueue Element(queue=w1895, element=w1891, error in (no error)=w1894) -> (queue out=w1888:refnum<queue>, error out=w1890:errorcluster)  [unwired: 1 in, 1 out]
          }
          frame #1 {
            n798 = for {
              N: "eV6 User set time \n(Inflight) (sec)" -> [w1902]
              i -> [w1901]
              n799 = Subtract(x=w1902, y=w1901) -> (x-y=w1900:i32)
              n800 = Decrement(x=w1900) -> (x-1=w1899:i32)
              n801 = local write "SO2 Zeroing (Inflight)\nTime Remain (sec)"(w1899) -> ()
              n802 = Wait (ms)(milliseconds to wait=u32 1000) -> ()  [unwired: 1 out]
            }
          }
          frame #2 {
            w1904 = FALSE
            n803 = Bundle(cluster=T4 {"Message"="", "Message Data"=variant} ("Message Cluster"), "Message"="V6", "Message Data"=w1904) -> (w1908:T4)
            n804 = local write "SO2 eV6"(w1904) -> ()
            n805 = Enqueue Element(queue=w1907, element=w1908, error in (no error)=w1906) -> (error out=w1905:errorcluster)  [unwired: 1 in, 2 out]
          }
          frame #3 {
            n806 = local write "SO2 Inflight \nZeroing"(FALSE ("SO2 Flush")) -> ()
          }
        }
      }
      event "SO2 Zero CAL": Value Change {
        n807 = event-data() -> ()  [unwired: 1 in, 1 out]
        n808 = flat-sequence {
          tunnel: [w1925] -> w1920
          tunnel: [w1924] -> w1918
          tunnel: w1922 -> [w1930]
          tunnel: w1921 -> [w1929]
          tunnel: w1920 -> [w1934]
          tunnel: [w1933] -> w1919
          tunnel: w1918 -> [w1935]
          tunnel: [w1931] -> w1917
          tunnel: [w1941] -> w1916
          tunnel: [w1940] -> w1915
          tunnel: w1917 -> [w1945]
          tunnel: w1919 -> [w1943]
          tunnel: w1916 -> [w1997]
          tunnel: w1915 -> [w1996]
          tunnel: [w1995] -> w1914
          tunnel: [w1994] -> w1913
          tunnel: w1914 -> [w2011]
          tunnel: w1913 -> [w2010]
          frame #0 {
            w1923 = TRUE ("SO2 Flush")
            n809 = Bundle(cluster=T4 {"Message"="", "Message Data"=variant} ("Message Cluster"), "Message"="V9", "Message Data"=w1923) -> (w1926:T4)
            n810 = local write "eV9"(w1923) -> ()
            n811 = Enqueue Element(queue=w1930, element=w1926, error in (no error)=w1929) -> (queue out=w1924:refnum<queue>, error out=w1925:errorcluster)  [unwired: 1 in, 1 out]
          }
          frame #1 {
            n812 = local read "MFC_2 User Set Value"() -> (w1932:dbl)
            n813 = local write "MFC_2\nSLPM Value"(w1932) -> ()
            n814 = Bundle(cluster=T4 {"Message"="", "Message Data"=variant} ("Message Cluster"), "Message"="MFC_2", "Message Data"=w1932) -> (w1936:T4)
            n815 = Enqueue Element(queue=w1935, element=w1936, error in (no error)=w1934) -> (queue out=w1931:refnum<queue>, error out=w1933:errorcluster)  [unwired: 1 in, 1 out]
          }
          frame #2 {
            n816 = for {
              N: "eV9 flush User\nset time (sec)" -> [w1988]
              tunnel: [w1979] -> w1944
              tunnel: w1945 -> [w1979]
              tunnel: [w1978] -> w1942
              tunnel: w1943 -> [w1978]
              tunnel: [w1977] -> w1939
              i -> [w1987]
              stop <- w1977 stop-if-true
              n817 = local read "SO2 Calibration Abort"() -> (w1984:bool)
              n818 = case shown="True" w1984 {
                selector: w1984 -> [w1991 _]
                tunnel: [w1991 w1992] -> w1982
                frame False {
                }
                frame True {
                  n819 = Two Button Dialog(message="Are you sure to abort SO2 Cal?") -> (T button?=w1992:bool)  [unwired: 2 in]
                }
              }
              n820 = Subtract(x=w1988, y=w1987) -> (x-y=w1986:i32)
              n821 = Decrement(x=w1986) -> (x-1=w1980:i32)
              n822 = Wait (ms)(milliseconds to wait=u32 1000) -> ()  [unwired: 1 out]
              n823 = local read "Network disconnected"() -> (w1983:bool)
              n824 = Or(x=w1983, y=w1982) -> (x .or. y?=w1977:bool)
              n825 = Select(t=0, s=w1977, f=w1980) -> (s? t:f=w1981:i32)
              n826 = local write "SO2 Zero CAL Flush\nTime Remain (sec)"(w1981) -> ()
              n827 = case shown="False" w1982 {
                selector: w1982 -> [w1990 _]
                frame False {
                  n828 = local write "SO2 Calibration Abort"(w1990) -> ()
                }
                frame True {
                }
              }
            }
            n829 = case shown="False" w1939 {
              tunnel: w1944 -> [w1952 w1976]
              tunnel: w1942 -> [w1951 w1975]
              tunnel: [w1949 w1976] -> w1941
              tunnel: [w1947 w1975] -> w1940
              frame False {
                w1953 = TRUE ("SO2 Flush")
                # "carry on cal when no connection problem or abort not confirmed"
                n830 = Bundle(cluster=T4 {"Message"="", "Message Data"=variant} ("Message Cluster"), "Message"="V8", "Message Data"=w1953) -> (w1954:T4)
                n831 = local write "eV8"(w1953) -> ()
                n832 = Enqueue Element(queue=w1952, element=w1954, error in (no error)=w1951) -> (queue out=w1950:refnum<queue>, error out=w1948:errorcluster)  [unwired: 1 in, 1 out]
                n833 = for {
                  N: "eV8 User\nset time (sec)" -> [w1969]
                  tunnel: [w1959] -> w1949
                  tunnel: w1950 -> [w1959]
                  tunnel: [w1958] -> w1947
                  tunnel: w1948 -> [w1958]
                  i -> [w1968]
                  stop <- w1960 stop-if-true
                  n834 = local read "SO2 Calibration Abort"() -> (w1966:bool)
                  n835 = case shown="True" w1966 {
                    selector: w1966 -> [w1972 _]
                    tunnel: [w1972 w1973] -> w1963
                    frame False {
                    }
                    frame True {
                      n836 = Two Button Dialog(message="Are you sure to abort SO2 Cal?") -> (T button?=w1973:bool)  [unwired: 2 in]
                    }
                  }
                  n837 = Subtract(x=w1969, y=w1968) -> (x-y=w1967:i32)
                  n838 = local read "Network disconnected"() -> (w1964:bool)
                  n839 = Decrement(x=w1967) -> (x-1=w1962:i32)
                  n840 = Or(x=w1964, y=w1963) -> (x .or. y?=w1960:bool)
                  n841 = Select(t=0, s=w1960, f=w1962) -> (s? t:f=w1961:i32)
                  n842 = case shown="False" w1963 {
                    selector: w1963 -> [w1971 _]
                    frame False {
                      n843 = local write "SO2 Calibration Abort"(w1971) -> ()
                    }
                    frame True {
                    }
                  }
                  n844 = local write "SO2 Zero CAL\nTime Remain (sec)"(w1961) -> ()
                  n845 = Wait (ms)(milliseconds to wait=u32 1000) -> ()  [unwired: 1 out]
                }
              }
              frame True {
                # "Ignore the rest of the cal when there is connection problem or abort confirmed"
              }
            }
          }
          frame #3 {
            n846 = Cluster To Array(cluster=cluster{"Message":string, "Message 2":string} {"Message"="V8", "Message 2"="V9"}) -> (array=w1999:string[])
            n847 = for {
              tunnel: w1999 -> [w2006] mode=indexing
              tunnel: FALSE ("SO2 Flush") -> [w2005]
              tunnel: w1997 -> [w2004]
              tunnel: w1996 -> [w2003]
              tunnel: [w2002] -> w1995
              tunnel: [w2001] -> w1994
              n848 = Bundle(cluster=T4 {"Message"="", "Message Data"=variant} ("Message Cluster"), "Message"=w2006, "Message Data"=w2005) -> (w2007:T4)
              n849 = Enqueue Element(queue=w2004, element=w2007, error in (no error)=w2003) -> (queue out=w2002:refnum<queue>, error out=w2001:errorcluster)  [unwired: 1 in, 1 out]
            }
          }
          frame #4 {
            w2009 = 0.0 ("MFC_2\nSLPM Value")
            n850 = local write "MFC_2\nSLPM Value"(w2009) -> ()
            n851 = Bundle(cluster=T4 {"Message"="", "Message Data"=variant} ("Message Cluster"), "Message"="MFC_2", "Message Data"=w2009) -> (w2012:T4)
            n852 = Enqueue Element(queue=w2011, element=w2012, error in (no error)=w2010) -> ()  [unwired: 1 in, 3 out]
          }
          frame #5 {
            w2015 = FALSE ("SO2 Flush")
            n853 = local write "eV9"(w2015) -> ()
            n854 = local write "eV8"(w2015) -> ()
            n855 = local write "SO2 Zero CAL"(w2015) -> ()
            n856 = local write "SO2 Calibration Abort"(w2015) -> ()
          }
        }
      }
      event "SO2 Span Calibration": Value Change {
        n857 = event-data() -> ()  [unwired: 1 in, 1 out]
        n858 = flat-sequence {
          tunnel: w2032 -> [w2037]
          tunnel: w2033 -> [w2038]
          tunnel: [w2035] -> w2021
          tunnel: [w2036] -> w2020
          tunnel: [w2045] -> w2019
          tunnel: [w2043] -> w2017
          tunnel: w2021 -> [w2046]
          tunnel: w2020 -> [w2047]
          tunnel: w2019 -> [w2054]
          tunnel: [w2053] -> w2018
          tunnel: w2017 -> [w2052]
          tunnel: [w2051] -> w2016
          tunnel: [w2068] -> w2031
          tunnel: [w2067] -> w2029
          tunnel: w2018 -> [w2072]
          tunnel: w2016 -> [w2065]
          tunnel: w2031 -> [w2076]
          tunnel: [w2075] -> w2030
          tunnel: w2029 -> [w2077]
          tunnel: [w2073] -> w2028
          tunnel: [w2084] -> w2027
          tunnel: [w2083] -> w2026
          tunnel: w2028 -> [w2088]
          tunnel: w2030 -> [w2086]
          tunnel: w2027 -> [w2139]
          tunnel: w2026 -> [w2138]
          tunnel: [w2137] -> w2025
          tunnel: [w2136] -> w2024
          tunnel: w2025 -> [w2155]
          tunnel: w2024 -> [w2154]
          tunnel: [w2152] -> w2023
          tunnel: [w2151] -> w2022
          tunnel: w2023 -> [w2160]
          tunnel: w2022 -> [w2159]
          frame #0 {
            n859 = local write "SO2 Auto Zeroing"(FALSE ("SO2 Auto Zeroing")) -> ()
            n860 = Bundle(cluster=T4 {"Message"="", "Message Data"=variant} ("Message Cluster"), "Message"="Auto_zero", "Message Data"=FALSE) -> (w2040:T4)
            n861 = Enqueue Element(queue=w2038, element=w2040, error in (no error)=w2037) -> (queue out=w2035:refnum<queue>, error out=w2036:errorcluster)  [unwired: 1 in, 1 out]
          }
          frame #1 {
            n862 = Bundle(cluster=T4 {"Message"="", "Message Data"=variant} ("Message Cluster"), "Message"="mean_cal_status", "Message Data"=FALSE) -> (w2048:T4)
            n863 = Enqueue Element(queue=w2046, element=w2048, error in (no error)=w2047) -> (queue out=w2043:refnum<queue>, error out=w2045:errorcluster)  [unwired: 1 in, 1 out]
          }
          frame #2 {
            n864 = node-c288() -> (w2056:T6)  [unwired: 4 in]
            n865 = timed-loop {
              timing: w2056 -> [_]
              timing-out: [_] -> w2055
              tunnel: [w2058] -> w2053
              tunnel: w2054 -> [w2058]
              tunnel: w2052 -> [w2057]
              tunnel: [w2057] -> w2051
              stop <- w2059 stop-if-true
              n866 = node-c288() -> ()  [unwired: 1 in, 1 out]
              n867 = node-c288() -> ()  [unwired: 1 in, 1 out]
              n868 = One Button Dialog(message="Is Span Gas connected to CALDECK?") -> (true=w2059:bool)  [unwired: 1 in]
            }
            n869 = node-c288(w2055) -> ()  [unwired: 1 out]
          }
          frame #3 {
            w2066 = TRUE ("SO2 Flush")
            n870 = Bundle(cluster=T4 {"Message"="", "Message Data"=variant} ("Message Cluster"), "Message"="V9", "Message Data"=w2066) -> (w2069:T4)
            n871 = local write "eV9"(w2066) -> ()
            n872 = Enqueue Element(queue=w2065, element=w2069, error in (no error)=w2072) -> (queue out=w2067:refnum<queue>, error out=w2068:errorcluster)  [unwired: 1 in, 1 out]
          }
          frame #4 {
            n873 = local read "MFC_2 User Set Value"() -> (w2074:dbl)
            n874 = local write "MFC_2\nSLPM Value"(w2074) -> ()
            n875 = Bundle(cluster=T4 {"Message"="", "Message Data"=variant} ("Message Cluster"), "Message"="MFC_2", "Message Data"=w2074) -> (w2078:T4)
            n876 = Enqueue Element(queue=w2077, element=w2078, error in (no error)=w2076) -> (queue out=w2073:refnum<queue>, error out=w2075:errorcluster)  [unwired: 1 in, 1 out]
          }
          frame #5 {
            n877 = for {
              N: "eV9 span\nflush (sec)" -> [w2130]
              tunnel: [w2121] -> w2087
              tunnel: w2088 -> [w2121]
              tunnel: [w2120] -> w2085
              tunnel: w2086 -> [w2120]
              tunnel: [w2119] -> w2082
              i -> [w2129]
              stop <- w2119 stop-if-true
              n878 = local read "SO2 Calibration Abort"() -> (w2126:bool)
              n879 = case shown="True" w2126 {
                selector: w2126 -> [w2133 _]
                tunnel: [w2133 w2134] -> w2124
                frame False {
                }
                frame True {
                  n880 = Two Button Dialog(message="Are you sure to abort SO2 Cal?") -> (T button?=w2134:bool)  [unwired: 2 in]
                }
              }
              n881 = Subtract(x=w2130, y=w2129) -> (x-y=w2128:i32)
              n882 = Decrement(x=w2128) -> (x-1=w2122:i32)
              n883 = Wait (ms)(milliseconds to wait=u32 1000) -> ()  [unwired: 1 out]
              n884 = local read "Network disconnected"() -> (w2125:bool)
              n885 = Or(x=w2125, y=w2124) -> (x .or. y?=w2119:bool)
              n886 = Select(t=0, s=w2119, f=w2122) -> (s? t:f=w2123:i32)
              n887 = local write "SO2 Zero CAL Flush\nTime Remain (sec)"(w2123) -> ()
              n888 = case shown="False" w2124 {
                selector: w2124 -> [w2132 _]
                frame False {
                  n889 = local write "SO2 Calibration Abort"(w2132) -> ()
                }
                frame True {
                }
              }
            }
            n890 = case shown="False" w2082 {
              tunnel: w2087 -> [w2095 w2118]
              tunnel: w2085 -> [w2094 w2117]
              tunnel: [w2092 w2118] -> w2084
              tunnel: [w2090 w2117] -> w2083
              frame False {
                w2096 = TRUE ("SO2 Flush")
                # "carry on cal when no connection problem or abort not confirmed"
                n891 = Bundle(cluster=T4 {"Message"="", "Message Data"=variant} ("Message Cluster"), "Message"="V8", "Message Data"=w2096) -> (w2097:T4)
                n892 = local write "eV8"(w2096) -> ()
                n893 = Enqueue Element(queue=w2095, element=w2097, error in (no error)=w2094) -> (queue out=w2093:refnum<queue>, error out=w2091:errorcluster)  [unwired: 1 in, 1 out]
                n894 = for {
                  N: "eV8 span\n(sec)" -> [w2111]
                  tunnel: [w2101] -> w2092
                  tunnel: w2093 -> [w2101]
                  tunnel: [w2100] -> w2090
                  tunnel: w2091 -> [w2100]
                  i -> [w2110]
                  stop <- w2102 stop-if-true
                  n895 = local read "SO2 Calibration Abort"() -> (w2108:bool)
                  n896 = case shown="True" w2108 {
                    selector: w2108 -> [w2114 _]
                    tunnel: [w2114 w2115] -> w2105
                    frame False {
                    }
                    frame True {
                      n897 = Two Button Dialog(message="Are you sure to abort SO2 Cal?") -> (T button?=w2115:bool)  [unwired: 2 in]
                    }
                  }
                  n898 = Subtract(x=w2111, y=w2110) -> (x-y=w2109:i32)
                  n899 = local read "Network disconnected"() -> (w2106:bool)
                  n900 = Decrement(x=w2109) -> (x-1=w2104:i32)
                  n901 = Or(x=w2106, y=w2105) -> (x .or. y?=w2102:bool)
                  n902 = Select(t=0, s=w2102, f=w2104) -> (s? t:f=w2103:i32)
                  n903 = case shown="False" w2105 {
                    selector: w2105 -> [w2113 _]
                    frame False {
                      n904 = local write "SO2 Calibration Abort"(w2113) -> ()
                    }
                    frame True {
                    }
                  }
                  n905 = local write "SO2 Zero CAL\nTime Remain (sec)"(w2103) -> ()
                  n906 = Wait (ms)(milliseconds to wait=u32 1000) -> ()  [unwired: 1 out]
                }
              }
              frame True {
                # "Ignore the rest of the cal when there is connection problem or abort confirmed"
              }
            }
          }
          frame #6 {
            n907 = Cluster To Array(cluster=cluster{"Message":string, "Message 2":string} {"Message"="V8", "Message 2"="V9"}) -> (array=w2141:string[])
            n908 = for {
              tunnel: w2141 -> [w2148] mode=indexing
              tunnel: FALSE ("SO2 Flush") -> [w2147]
              tunnel: w2139 -> [w2146]
              tunnel: w2138 -> [w2145]
              tunnel: [w2144] -> w2137
              tunnel: [w2143] -> w2136
              n909 = Bundle(cluster=T4 {"Message"="", "Message Data"=variant} ("Message Cluster"), "Message"=w2148, "Message Data"=w2147) -> (w2149:T4)
              n910 = Enqueue Element(queue=w2146, element=w2149, error in (no error)=w2145) -> (queue out=w2144:refnum<queue>, error out=w2143:errorcluster)  [unwired: 1 in, 1 out]
            }
          }
          frame #7 {
            w2153 = 0.0 ("MFC_2\nSLPM Value")
            n911 = local write "MFC_2\nSLPM Value"(w2153) -> ()
            n912 = Bundle(cluster=T4 {"Message"="", "Message Data"=variant} ("Message Cluster"), "Message"="MFC_2", "Message Data"=w2153) -> (w2156:T4)
            n913 = Enqueue Element(queue=w2155, element=w2156, error in (no error)=w2154) -> (queue out=w2152:refnum<queue>, error out=w2151:errorcluster)  [unwired: 1 in, 1 out]
          }
          frame #8 {
            n914 = Bundle(cluster=T4 {"Message"="", "Message Data"=variant} ("Message Cluster"), "Message"="mean_cal_status", "Message Data"=TRUE) -> (w2162:T4)
            n915 = Enqueue Element(queue=w2160, element=w2162, error in (no error)=w2159) -> ()  [unwired: 1 in, 3 out]
          }
          frame #9 {
            w2165 = FALSE ("SO2 Flush")
            n916 = local write "eV8"(w2165) -> ()
            n917 = local write "eV9"(w2165) -> ()
            n918 = local write "SO2 Span Calibration"(w2165) -> ()
            n919 = local write "SO2 Calibration Abort"(w2165) -> ()
          }
        }
      }
      event "SO2 Zero Calibration": Value Change {
        n920 = event-data() -> ()  [unwired: 1 in, 1 out]
        n921 = flat-sequence {
          tunnel: w2180 -> [w2186]
          tunnel: w2181 -> [w2187]
          tunnel: [w2184] -> w2171
          tunnel: [w2185] -> w2170
          tunnel: [w2193] -> w2169
          tunnel: [w2191] -> w2167
          tunnel: w2171 -> [w2194]
          tunnel: w2170 -> [w2195]
          tunnel: w2169 -> [w2201]
          tunnel: [w2200] -> w2168
          tunnel: w2167 -> [w2202]
          tunnel: [w2199] -> w2166
          tunnel: [w2216] -> w2179
          tunnel: [w2215] -> w2177
          tunnel: w2168 -> [w2220]
          tunnel: w2166 -> [w2213]
          tunnel: w2179 -> [w2224]
          tunnel: [w2223] -> w2178
          tunnel: w2177 -> [w2225]
          tunnel: [w2221] -> w2176
          tunnel: [w2232] -> w2175
          tunnel: [w2231] -> w2174
          tunnel: w2176 -> [w2236]
          tunnel: w2178 -> [w2234]
          tunnel: w2175 -> [w2287]
          tunnel: w2174 -> [w2286]
          tunnel: [w2285] -> w2173
          tunnel: [w2284] -> w2172
          tunnel: w2173 -> [w2301]
          tunnel: w2172 -> [w2300]
          frame #0 {
            n922 = local write "SO2 Auto Zeroing"(FALSE) -> ()
            n923 = Bundle(cluster=T4 {"Message"="", "Message Data"=variant} ("Message Cluster"), "Message"="Auto_zero", "Message Data"=FALSE) -> (w2190:T4)
            n924 = Enqueue Element(queue=w2187, element=w2190, error in (no error)=w2186) -> (queue out=w2184:refnum<queue>, error out=w2185:errorcluster)  [unwired: 1 in, 1 out]
          }
          frame #1 {
            n925 = Bundle(cluster=T4 {"Message"="", "Message Data"=variant} ("Message Cluster"), "Message"="mean_cal_status", "Message Data"=TRUE) -> (w2196:T4)
            n926 = Enqueue Element(queue=w2194, element=w2196, error in (no error)=w2195) -> (queue out=w2191:refnum<queue>, error out=w2193:errorcluster)  [unwired: 1 in, 1 out]
          }
          frame #2 {
            n927 = node-c288() -> (w2204:T6)  [unwired: 4 in]
            n928 = timed-loop {
              timing: w2204 -> [_]
              timing-out: [_] -> w2203
              tunnel: [w2206] -> w2200
              tunnel: w2201 -> [w2206]
              tunnel: w2202 -> [w2205]
              tunnel: [w2205] -> w2199
              stop <- w2207 stop-if-true
              n929 = node-c288() -> ()  [unwired: 1 in, 1 out]
              n930 = node-c288() -> ()  [unwired: 1 in, 1 out]
              n931 = One Button Dialog(message="Is Zero Gas connected to CALDECK?") -> (true=w2207:bool)  [unwired: 1 in]
            }
            n932 = node-c288(w2203) -> ()  [unwired: 1 out]
          }
          frame #3 {
            w2214 = TRUE ("SO2 Flush")
            n933 = Bundle(cluster=T4 {"Message"="", "Message Data"=variant} ("Message Cluster"), "Message"="V9", "Message Data"=w2214) -> (w2217:T4)
            n934 = local write "eV9"(w2214) -> ()
            n935 = Enqueue Element(queue=w2213, element=w2217, error in (no error)=w2220) -> (queue out=w2215:refnum<queue>, error out=w2216:errorcluster)  [unwired: 1 in, 1 out]
          }
          frame #4 {
            n936 = local read "MFC_2 User Set Value"() -> (w2222:dbl)
            n937 = local write "MFC_2\nSLPM Value"(w2222) -> ()
            n938 = Bundle(cluster=T4 {"Message"="", "Message Data"=variant} ("Message Cluster"), "Message"="MFC_2", "Message Data"=w2222) -> (w2226:T4)
            n939 = Enqueue Element(queue=w2225, element=w2226, error in (no error)=w2224) -> (queue out=w2221:refnum<queue>, error out=w2223:errorcluster)  [unwired: 1 in, 1 out]
          }
          frame #5 {
            n940 = for {
              N: "eV9 zero\nflush (sec)" -> [w2278]
              tunnel: [w2269] -> w2235
              tunnel: w2236 -> [w2269]
              tunnel: [w2268] -> w2233
              tunnel: w2234 -> [w2268]
              tunnel: [w2267] -> w2230
              i -> [w2277]
              stop <- w2267 stop-if-true
              n941 = local read "SO2 Calibration Abort"() -> (w2274:bool)
              n942 = case shown="True" w2274 {
                selector: w2274 -> [w2281 _]
                tunnel: [w2281 w2282] -> w2272
                frame False {
                }
                frame True {
                  n943 = Two Button Dialog(message="Are you sure to abort SO2 Cal?") -> (T button?=w2282:bool)  [unwired: 2 in]
                }
              }
              n944 = Subtract(x=w2278, y=w2277) -> (x-y=w2276:i32)
              n945 = Decrement(x=w2276) -> (x-1=w2270:i32)
              n946 = Wait (ms)(milliseconds to wait=u32 1000) -> ()  [unwired: 1 out]
              n947 = local read "Network disconnected"() -> (w2273:bool)
              n948 = Or(x=w2273, y=w2272) -> (x .or. y?=w2267:bool)
              n949 = Select(t=0, s=w2267, f=w2270) -> (s? t:f=w2271:i32)
              n950 = local write "SO2 Zero CAL Flush\nTime Remain (sec)"(w2271) -> ()
              n951 = case shown="False" w2272 {
                selector: w2272 -> [w2280 _]
                frame False {
                  n952 = local write "SO2 Calibration Abort"(w2280) -> ()
                }
                frame True {
                }
              }
            }
            n953 = case shown="False" w2230 {
              tunnel: w2235 -> [w2243 w2266]
              tunnel: w2233 -> [w2242 w2265]
              tunnel: [w2240 w2266] -> w2232
              tunnel: [w2238 w2265] -> w2231
              frame False {
                w2244 = TRUE ("SO2 Flush")
                # "carry on cal when no connection problem or abort not confirmed"
                n954 = Bundle(cluster=T4 {"Message"="", "Message Data"=variant} ("Message Cluster"), "Message"="V8", "Message Data"=w2244) -> (w2245:T4)
                n955 = local write "eV8"(w2244) -> ()
                n956 = Enqueue Element(queue=w2243, element=w2245, error in (no error)=w2242) -> (queue out=w2241:refnum<queue>, error out=w2239:errorcluster)  [unwired: 1 in, 1 out]
                n957 = for {
                  N: "eV8 zero\n(sec)" -> [w2259]
                  tunnel: [w2249] -> w2240
                  tunnel: w2241 -> [w2249]
                  tunnel: [w2248] -> w2238
                  tunnel: w2239 -> [w2248]
                  i -> [w2258]
                  stop <- w2250 stop-if-true
                  n958 = local read "SO2 Calibration Abort"() -> (w2256:bool)
                  n959 = case shown="True" w2256 {
                    selector: w2256 -> [w2262 _]
                    tunnel: [w2262 w2263] -> w2253
                    frame False {
                    }
                    frame True {
                      n960 = Two Button Dialog(message="Are you sure to abort SO2 Cal?") -> (T button?=w2263:bool)  [unwired: 2 in]
                    }
                  }
                  n961 = Subtract(x=w2259, y=w2258) -> (x-y=w2257:i32)
                  n962 = local read "Network disconnected"() -> (w2254:bool)
                  n963 = Decrement(x=w2257) -> (x-1=w2252:i32)
                  n964 = Or(x=w2254, y=w2253) -> (x .or. y?=w2250:bool)
                  n965 = Select(t=0, s=w2250, f=w2252) -> (s? t:f=w2251:i32)
                  n966 = case shown="False" w2253 {
                    selector: w2253 -> [w2261 _]
                    frame False {
                      n967 = local write "SO2 Calibration Abort"(w2261) -> ()
                    }
                    frame True {
                    }
                  }
                  n968 = local write "SO2 Zero CAL\nTime Remain (sec)"(w2251) -> ()
                  n969 = Wait (ms)(milliseconds to wait=u32 1000) -> ()  [unwired: 1 out]
                }
              }
              frame True {
                # "Ignore the rest of the cal when there is connection problem or abort confirmed"
              }
            }
          }
          frame #6 {
            n970 = Cluster To Array(cluster=cluster{"Message":string, "Message 2":string} {"Message"="V8", "Message 2"="V9"}) -> (array=w2289:string[])
            n971 = for {
              tunnel: w2289 -> [w2296] mode=indexing
              tunnel: FALSE ("SO2 Flush") -> [w2295]
              tunnel: w2287 -> [w2294]
              tunnel: w2286 -> [w2293]
              tunnel: [w2292] -> w2285
              tunnel: [w2291] -> w2284
              n972 = Bundle(cluster=T4 {"Message"="", "Message Data"=variant} ("Message Cluster"), "Message"=w2296, "Message Data"=w2295) -> (w2297:T4)
              n973 = Enqueue Element(queue=w2294, element=w2297, error in (no error)=w2293) -> (queue out=w2292:refnum<queue>, error out=w2291:errorcluster)  [unwired: 1 in, 1 out]
            }
          }
          frame #7 {
            w2299 = 0.0 ("MFC_2\nSLPM Value")
            n974 = local write "MFC_2\nSLPM Value"(w2299) -> ()
            n975 = Bundle(cluster=T4 {"Message"="", "Message Data"=variant} ("Message Cluster"), "Message"="MFC_2", "Message Data"=w2299) -> (w2302:T4)
            n976 = Enqueue Element(queue=w2301, element=w2302, error in (no error)=w2300) -> ()  [unwired: 1 in, 3 out]
          }
          frame #8 {
            w2305 = FALSE ("SO2 Flush")
            n977 = local write "eV8"(w2305) -> ()
            n978 = local write "eV9"(w2305) -> ()
            n979 = local write "SO2 Zero Calibration"(w2305) -> ()
            n980 = local write "SO2 Calibration Abort"(w2305) -> ()
          }
        }
      }
      event "eV8 User\nset time (sec)": Value Change {
        n981 = event-data() -> ("NewVal"=w2308:i32)  [unwired: 1 in]
        n982 = Bundle(cluster=T4 {"Message"="", "Message Data"=variant} ("Message Cluster"), "Message"="eV8_user_set_time", "Message Data"=w2308) -> (w2309:T4)
        n983 = Enqueue Element(queue=w2307, element=w2309, error in (no error)=w2306) -> ()  [unwired: 1 in, 3 out]
      }
      event "Offset Mean Zero Calculation (default = ON)\nOFF = User input\nOn = Mean zero calculated with ev8": Value Change {
        n984 = event-data() -> ("NewVal"=w2314:bool)  [unwired: 1 in]
        n985 = Bundle(cluster=T4 {"Message"="", "Message Data"=variant} ("Message Cluster"), "Message"="mean_cal_status", "Message Data"=w2314) -> (w2315:T4)
        n986 = Enqueue Element(queue=w2313, element=w2315, error in (no error)=w2312) -> ()  [unwired: 1 in, 3 out]
      }
      event "MFC_2\nSLPM Value": Value Change {
        n987 = event-data() -> ("NewVal"=w2321:dbl)  [unwired: 1 in]
        n988 = Bundle(cluster=T4 {"Message"="", "Message Data"=variant} ("Message Cluster"), "Message"="MFC_2", "Message Data"=w2321) -> (w2319:T4)
        n989 = Enqueue Element(queue=w2324, element=w2319, error in (no error)=w2323) -> (error out=w2318:errorcluster)  [unwired: 1 in, 2 out]
      }
      event "SO2 Inflight MOCCA Alarm\n(default = OFF)": Value Change {
        n990 = event-data() -> ("NewVal"=w2328:bool)  [unwired: 1 in]
        n991 = Bundle(cluster=T4 {"Message"="", "Message Data"=variant} ("Message Cluster"), "Message"="SO2_MOCCA_Alarm", "Message Data"=w2328) -> (w2329:T4)
        n992 = Enqueue Element(queue=w2327, element=w2329, error in (no error)=w2326) -> (error out=w2325:errorcluster)  [unwired: 1 in, 2 out]
      }
      event "MOCCA window \ndelay time (sec)": Value Change {
        n993 = event-data() -> ("NewVal"=w2334:i32)  [unwired: 1 in]
        n994 = Bundle(cluster=T4 {"Message"="", "Message Data"=variant} ("Message Cluster"), "Message"="MOCCA_window_delay_time", "Message Data"=w2334) -> (w2336:T4)
        n995 = Enqueue Element(queue=w2335, element=w2336, error in (no error)=w2333) -> (error out=w2332:errorcluster)  [unwired: 1 in, 2 out]
      }
      event "MOCCA Limit": Value Change {
        n996 = event-data() -> ("NewVal"=w2339:i32)  [unwired: 1 in]
        n997 = Bundle(cluster=T4 {"Message"="", "Message Data"=variant} ("Message Cluster"), "Message"="MOCCA_limit", "Message Data"=w2339) -> (w2342:T4)
        n998 = Enqueue Element(queue=w2341, element=w2342, error in (no error)=w2340) -> ()  [unwired: 1 in, 3 out]
      }
      event "Save Calibration gas\ncylinder concentration to file": Value Change {
        n999 = event-data() -> ("NewVal"=w2345:bool)  [unwired: 1 in]
        n1000 = Bundle(cluster=T4 {"Message"="", "Message Data"=variant} ("Message Cluster"), "Message"="calcon_save", "Message Data"=w2345) -> (w2349:T4)
        n1001 = Enqueue Element(queue=w2348, element=w2349, error in (no error)=w2347) -> (error out=w2346:errorcluster)  [unwired: 1 in, 2 out]
      }
      event "Calibration gas cylinder \nconcentration (ppb)": Value Change {
        n1002 = event-data() -> ("NewVal"=w2352:dbl)  [unwired: 1 in]
        n1003 = Bundle(cluster=T4 {"Message"="", "Message Data"=variant} ("Message Cluster"), "Message"="cal_gas_cylin_conc", "Message Data"=w2352) -> (w2355:T4)
        n1004 = Enqueue Element(queue=w2354, element=w2355, error in (no error)=w2353) -> ()  [unwired: 1 in, 3 out]
      }
      event "Simulate MOCCA Conc": Value Change {
        n1005 = event-data() -> ("NewVal"=w2358:dbl)  [unwired: 1 in]
        n1006 = Bundle(cluster=T4 {"Message"="", "Message Data"=variant} ("Message Cluster"), "Message"="sim_MOCCA_conc", "Message Data"=w2358) -> (w2361:T4)
        n1007 = Enqueue Element(queue=w2360, element=w2361, error in (no error)=w2359) -> ()  [unwired: 1 in, 3 out]
      }
      event "MFC_3\nSLPM Value": Value Change {
        n1008 = event-data() -> ("NewVal"=w2367:dbl)  [unwired: 1 in]
        n1009 = Bundle(cluster=T4 {"Message"="", "Message Data"=variant} ("Message Cluster"), "Message"="MFC_3", "Message Data"=w2367) -> (w2365:T4)
        n1010 = Enqueue Element(queue=w2370, element=w2365, error in (no error)=w2369) -> (error out=w2364:errorcluster)  [unwired: 1 in, 2 out]
      }
      event "eV8": Value Change {
        n1011 = event-data() -> ("NewVal"=w2371:bool)  [unwired: 1 in]
        n1012 = Bundle(cluster=T4 {"Message"="", "Message Data"=variant} ("Message Cluster"), "Message"="V8", "Message Data"=w2371) -> (w2375:T4)
        n1013 = Enqueue Element(queue=w2374, element=w2375, error in (no error)=w2373) -> (error out=w2372:errorcluster)  [unwired: 1 in, 2 out]
      }
      event "SO2 eV6": Value Change {
        n1014 = event-data() -> ("NewVal"=w2378:bool)  [unwired: 1 in]
        n1015 = Bundle(cluster=T4 {"Message"="", "Message Data"=variant} ("Message Cluster"), "Message"="V6", "Message Data"=w2378) -> (w2382:T4)
        n1016 = Enqueue Element(queue=w2381, element=w2382, error in (no error)=w2380) -> (error out=w2379:errorcluster)  [unwired: 1 in, 2 out]
      }
      event "Simulate Conc": Value Change {
        n1017 = event-data() -> ("NewVal"=w2385:bool)  [unwired: 1 in]
        n1018 = Bundle(cluster=T4 {"Message"="", "Message Data"=variant} ("Message Cluster"), "Message"="Simulate Conc", "Message Data"=w2385) -> (w2389:T4)
        n1019 = Enqueue Element(queue=w2388, element=w2389, error in (no error)=w2387) -> (error out=w2386:errorcluster)  [unwired: 1 in, 2 out]
      }
      event "SO2 UDP Time Offset": Value Change {
        n1020 = event-data() -> ("NewVal"=w2392:i32)  [unwired: 1 in]
        n1021 = Bundle(cluster=T4 {"Message"="", "Message Data"=variant} ("Message Cluster"), "Message"="UDP Time Offset", "Message Data"=w2392) -> (w2396:T4)
        n1022 = Enqueue Element(queue=w2395, element=w2396, error in (no error)=w2394) -> (error out=w2393:errorcluster)  [unwired: 1 in, 2 out]
      }
      event "Simulate STEL Conc": Value Change {
        n1023 = event-data() -> ("NewVal"=w2399:dbl)  [unwired: 1 in]
        n1024 = Bundle(cluster=T4 {"Message"="", "Message Data"=variant} ("Message Cluster"), "Message"="Simulate STEL Conc", "Message Data"=w2399) -> (w2403:T4)
        n1025 = Enqueue Element(queue=w2402, element=w2403, error in (no error)=w2401) -> (error out=w2400:errorcluster)  [unwired: 1 in, 2 out]
      }
      event "Simulate TWA Conc": Value Change {
        n1026 = event-data() -> ("NewVal"=w2406:dbl)  [unwired: 1 in]
        n1027 = Bundle(cluster=T4 {"Message"="", "Message Data"=variant} ("Message Cluster"), "Message"="Simulate TWA Conc", "Message Data"=w2406) -> (w2410:T4)
        n1028 = Enqueue Element(queue=w2409, element=w2410, error in (no error)=w2408) -> (error out=w2407:errorcluster)  [unwired: 1 in, 2 out]
      }
      event "10mins STEL Limit": Value Change {
        n1029 = event-data() -> ("NewVal"=w2413:i32)  [unwired: 1 in]
        n1030 = Bundle(cluster=T4 {"Message"="", "Message Data"=variant} ("Message Cluster"), "Message"="10mins STEL Limit", "Message Data"=w2413) -> (w2417:T4)
        n1031 = Enqueue Element(queue=w2416, element=w2417, error in (no error)=w2415) -> (error out=w2414:errorcluster)  [unwired: 1 in, 2 out]
      }
      event "8hr TWA Limit": Value Change {
        n1032 = event-data() -> ("NewVal"=w2420:i32)  [unwired: 1 in]
        n1033 = Bundle(cluster=T4 {"Message"="", "Message Data"=variant} ("Message Cluster"), "Message"="8hr TWA Limit", "Message Data"=w2420) -> (w2424:T4)
        n1034 = Enqueue Element(queue=w2423, element=w2424, error in (no error)=w2422) -> (error out=w2421:errorcluster)  [unwired: 1 in, 2 out]
      }
      event "SO2 Zero": Value Change {
        n1035 = event-data() -> ("NewVal"=w2427:dbl)  [unwired: 1 in]
        n1036 = Bundle(cluster=T4 {"Message"="", "Message Data"=variant} ("Message Cluster"), "Message"="Offset", "Message Data"=w2427) -> (w2431:T4)
        n1037 = Enqueue Element(queue=w2430, element=w2431, error in (no error)=w2429) -> (error out=w2428:errorcluster)  [unwired: 1 in, 2 out]
      }
      event "SO2 Sensitivity": Value Change {
        n1038 = event-data() -> ("NewVal"=w2434:dbl)  [unwired: 1 in]
        n1039 = Bundle(cluster=T4 {"Message"="", "Message Data"=variant} ("Message Cluster"), "Message"="Slope", "Message Data"=w2434) -> (w2438:T4)
        n1040 = Enqueue Element(queue=w2437, element=w2438, error in (no error)=w2436) -> (error out=w2435:errorcluster)  [unwired: 1 in, 2 out]
      }
      event "Confirm Flight Number": Value Change {
        n1041 = event-data() -> ()  [unwired: 1 in, 6 out]
        n1042 = flat-sequence {
          tunnel: w2444 -> [w2447]
          tunnel: w2445 -> [w2448]
          tunnel: [w2448] -> w2442
          tunnel: [w2447] -> w2441
          tunnel: [w2450] -> w2443
          tunnel: w2442 -> [w2452]
          tunnel: w2441 -> [w2451]
          frame #0 {
            n1043 = local write "cRIO File IO Stop\n(USB Flash Drive Unmount)"(FALSE ("cRIO File IO Stop\n(USB Flash Drive Unmount)")) -> ()
          }
          frame #1 {
            n1044 = local read "Flight Number"() -> (w2449:string)
            n1045 = Bundle(cluster=T4 {"Message"="", "Message Data"=variant} ("Message Cluster"), "Message"="Flight Number", "Message Data"=w2449) -> (w2453:T4)
            n1046 = Enqueue Element(queue=w2452, element=w2453, error in (no error)=w2451) -> (error out=w2450:errorcluster)  [unwired: 1 in, 2 out]
          }
        }
      }
      event "cRIO File IO Stop\n(USB Flash Drive Unmount)": Value Change {
        n1047 = event-data() -> ("NewVal"=w2456:bool)  [unwired: 1 in]
        n1048 = Bundle(cluster=T4 {"Message"="", "Message Data"=variant} ("Message Cluster"), "Message"="Stop File Write", "Message Data"=w2456) -> (w2460:T4)
        n1049 = Enqueue Element(queue=w2459, element=w2460, error in (no error)=w2458) -> (error out=w2457:errorcluster)  [unwired: 1 in, 2 out]
      }
    }
    "SO2 Event error out" <- w1764
  }
  n1050 = Create Network Stream Writer Endpoint(6:w45, 7:10 ("writer buffer size"), 9:w40, 10:"//192.168.101.17/command/reader/SO2" ("reader url"), 11:"/command/writer/SO2" ("writer name")) -> (0:w44:errorcluster, 3:w43:refnum<k21>)  [unwired: 2 in]
  n1051 = while {
    tunnel: w4 -> [w2467]
    tunnel: w3 -> [w2466]
    stop <- FALSE stop-if-true
    # "SO2 Auto Zero Handler Loop"
    n1052 = local read "Network disconnected"() -> (w2464:bool)
    n1053 = local read "SO2 Zero CAL"() -> (w2471:bool)
    n1054 = Equal?(x=w2471, y=FALSE) -> (x = y?=w2469:bool)
    n1055 = Equal?(x=w2464, y=FALSE) -> (x = y?=w2463:bool)
    n1056 = Compound Arithmetic op=AND("SO2 Auto Zeroing", w2469, w2463) -> (w2472:bool)
    n1057 = case shown="False" w2472 {
      tunnel: w2467 -> [_ w2491]
      tunnel: w2466 -> [_ w2490]
      frame False {
        n1058 = local write "Auto Zero\nIndicator"("Auto Zero Inactive; Manual Zero Allow" ("Auto Zero Indicator")) -> ()
        n1059 = local write "SO2 Pause\nAuto Zeroing"(FALSE ("SO2 Pause\nAuto Zeroing")) -> ()
        n1060 = property on="SO2 Zero CAL" class="Bool (strict)"("Visible"=TRUE) -> ()  [unwired: 2 in, 2 out]
      }
      frame True {
        n1061 = flat-sequence {
          tunnel: w2490 -> [w2500]
          tunnel: w2491 -> [w2501]
          tunnel: [w2501] -> w2489
          tunnel: [w2500] -> w2488
          tunnel: w2489 -> [w2510]
          tunnel: w2488 -> [w2509]
          tunnel: [w2508] -> w2487
          tunnel: [w2507] -> w2486
          tunnel: [w2516] -> w2497
          tunnel: [w2515] -> w2496
          tunnel: w2487 -> [w2520]
          tunnel: w2486 -> [w2521]
          tunnel: w2497 -> [w2525]
          tunnel: [w2524] -> w2495
          tunnel: w2496 -> [w2526]
          tunnel: [w2523] -> w2494
          tunnel: w2495 -> [w2534]
          tunnel: w2494 -> [w2536]
          tunnel: [w2532] -> w2479
          tunnel: [w2531] -> w2478
          tunnel: [w2586] -> w2493
          tunnel: [w2585] -> w2492
          tunnel: w2479 -> [w2588]
          tunnel: w2478 -> [w2587]
          tunnel: w2493 -> [w2604]
          tunnel: w2492 -> [w2603]
          tunnel: [w2601] -> w2484
          tunnel: [w2600] -> w2483
          tunnel: [w2609] -> w2485
          tunnel: w2484 -> [w2609]
          tunnel: w2483 -> [w2608]
          tunnel: [w2608] -> w2482
          tunnel: [w2614] -> w2481
          tunnel: w2482 -> [w2613]
          tunnel: w2485 -> [w2614]
          tunnel: [w2613] -> w2480
          tunnel: w2481 -> [w2648]
          tunnel: w2480 -> [w2647]
          frame #0 {
            n1062 = local write "Auto Zero\nIndicator"("Auto Zero In Progress" ("Auto Zero\nIndicator")) -> ()
            n1063 = while {
              stop <- w2502 stop-if-true
              n1064 = local read "eV9"() -> (w2504:bool)
              n1065 = Equal?(x=w2504, y=FALSE) -> (x = y?=w2502:bool)
              n1066 = Wait (ms)(milliseconds to wait=u32 1000) -> ()  [unwired: 1 out]
            }
            n1067 = property on="SO2 Zero CAL" class="Bool (strict)"("Visible"=FALSE) -> ()  [unwired: 2 in, 2 out]
          }
          frame #1 {
            n1068 = Bundle(cluster=T4 {"Message"="", "Message Data"=variant} ("Message Cluster"), "Message"="Auto_zero", "Message Data"=TRUE) -> (w2511:T4)
            n1069 = Enqueue Element(queue=w2510, element=w2511, error in (no error)=w2509) -> (queue out=w2507:refnum<queue>, error out=w2508:errorcluster)  [unwired: 1 in, 1 out]
          }
          frame #2 {
            w2514 = TRUE ("SO2 Flush")
            n1070 = Bundle(cluster=T4 {"Message"="", "Message Data"=variant} ("Message Cluster"), "Message"="V9", "Message Data"=w2514) -> (w2517:T4)
            n1071 = local write "eV9"(w2514) -> ()
            n1072 = Enqueue Element(queue=w2521, element=w2517, error in (no error)=w2520) -> (queue out=w2515:refnum<queue>, error out=w2516:errorcluster)  [unwired: 1 in, 1 out]
          }
          frame #3 {
            n1073 = local read "MFC_2 User Set Value"() -> (w2522:dbl)
            n1074 = local write "MFC_2 User Set Value"(w2522) -> ()
            n1075 = Bundle(cluster=T4 {"Message"="", "Message Data"=variant} ("Message Cluster"), "Message"="MFC_2", "Message Data"=w2522) -> (w2527:T4)
            n1076 = Enqueue Element(queue=w2526, element=w2527, error in (no error)=w2525) -> (queue out=w2523:refnum<queue>, error out=w2524:errorcluster)  [unwired: 1 in, 1 out]
          }
          frame #4 {
            n1077 = local read "eV9 flush User\nset time (sec)"() -> (w2537:i32)
            n1078 = for {
              N: w2537 -> [w2579]
              tunnel: [w2570] -> w2535
              tunnel: w2536 -> [w2570]
              tunnel: [w2569] -> w2533
              tunnel: w2534 -> [w2569]
              tunnel: [w2568] -> w2530
              i -> [w2578]
              stop <- w2568 stop-if-true
              n1079 = local read "Network disconnected"() -> (w2572:bool)
              n1080 = local read "SO2 Calibration Abort"() -> (w2573:bool)
              n1081 = case shown="True" w2573 {
                selector: w2573 -> [w2582 _]
                tunnel: [w2582 w2583] -> w2571
                frame False {
                }
                frame True {
                  n1082 = Two Button Dialog(message="Are you sure to abort SO2 Cal?") -> (T button?=w2583:bool)  [unwired: 2 in]
                }
              }
              n1083 = Subtract(x=w2579, y=w2578) -> (x-y=w2577:i32)
              n1084 = Decrement(x=w2577) -> (x-1=w2575:i32)
              n1085 = Or(x=w2571, y=w2572) -> (x .or. y?=w2568:bool)
              n1086 = Wait (ms)(milliseconds to wait=u32 1000) -> ()  [unwired: 1 out]
              n1087 = Select(t=0, s=w2568, f=w2575) -> (s? t:f=w2574:i32)
              n1088 = local write "SO2 Zero CAL Flush\nTime Remain (sec)"(w2574) -> ()
              n1089 = case shown="False" w2571 {
                selector: w2571 -> [w2581 _]
                frame False {
                  n1090 = local write "SO2 Calibration Abort"(w2581) -> ()
                }
                frame True {
                }
              }
            }
            n1091 = case shown="False" w2530 {
              tunnel: w2535 -> [w2543 w2567]
              tunnel: w2533 -> [w2542 w2566]
              tunnel: [w2541 w2567] -> w2532
              tunnel: [w2539 w2566] -> w2531
              frame False {
                w2544 = TRUE ("SO2 Flush")
                # "carry on cal when no connection problem or abort not confirmed"
                n1092 = Bundle(cluster=T4 {"Message"="", "Message Data"=variant} ("Message Cluster"), "Message"="V8", "Message Data"=w2544) -> (w2545:T4)
                n1093 = local write "eV8"(w2544) -> ()
                n1094 = Enqueue Element(queue=w2543, element=w2545, error in (no error)=w2542) -> (queue out=w2540:refnum<queue>, error out=w2538:errorcluster)  [unwired: 1 in, 1 out]
                n1095 = local read "eV8 User\nset time (sec)"() -> (w2548:i32)
                n1096 = for {
                  N: w2548 -> [w2560]
                  tunnel: w2540 -> [w2550]
                  tunnel: [w2550] -> w2541
                  tunnel: w2538 -> [w2549]
                  tunnel: [w2549] -> w2539
                  i -> [w2559]
                  stop <- w2551 stop-if-true
                  n1097 = local read "Network disconnected"() -> (w2555:bool)
                  n1098 = local read "SO2 Calibration Abort"() -> (w2557:bool)
                  n1099 = case shown="True" w2557 {
                    selector: w2557 -> [w2563 _]
                    tunnel: [w2563 w2564] -> w2552
                    frame False {
                    }
                    frame True {
                      n1100 = Two Button Dialog(message="Are you sure to abort SO2 Cal?") -> (T button?=w2564:bool)  [unwired: 2 in]
                    }
                  }
                  n1101 = Subtract(x=w2560, y=w2559) -> (x-y=w2558:i32)
                  n1102 = Decrement(x=w2558) -> (x-1=w2553:i32)
                  n1103 = Or(x=w2552, y=w2555) -> (x .or. y?=w2551:bool)
                  n1104 = Wait (ms)(milliseconds to wait=u32 1000) -> ()  [unwired: 1 out]
                  n1105 = Select(t=0, s=w2551, f=w2553) -> (s? t:f=w2554:i32)
                  n1106 = case shown="False" w2552 {
                    selector: w2552 -> [w2562 _]
                    frame False {
                      n1107 = local write "SO2 Calibration Abort"(w2562) -> ()
                    }
                    frame True {
                    }
                  }
                  n1108 = local write "SO2 Zero CAL\nTime Remain (sec)"(w2554) -> ()
                }
              }
              frame True {
                # "Ignore cal when connection problem or abort confirmed"
              }
            }
          }
          frame #5 {
            n1109 = Cluster To Array(cluster=cluster{"Message":string, "Message 2":string} {"Message"="V8", "Message 2"="V9"}) -> (array=w2590:string[])
            n1110 = for {
              tunnel: w2590 -> [w2597] mode=indexing
              tunnel: FALSE ("SO2 Flush") -> [w2596]
              tunnel: w2588 -> [w2595]
              tunnel: w2587 -> [w2594]
              tunnel: [w2593] -> w2586
              tunnel: [w2592] -> w2585
              n1111 = Bundle(cluster=T4 {"Message"="", "Message Data"=variant} ("Message Cluster"), "Message"=w2597, "Message Data"=w2596) -> (w2598:T4)
              n1112 = Enqueue Element(queue=w2595, element=w2598, error in (no error)=w2594) -> (queue out=w2593:refnum<queue>, error out=w2592:errorcluster)  [unwired: 1 in, 1 out]
            }
          }
          frame #6 {
            w2602 = 0.0 ("MFC_2\nSLPM Value")
            n1113 = local write "MFC_2\nSLPM Value"(w2602) -> ()
            n1114 = Bundle(cluster=T4 {"Message"="", "Message Data"=variant} ("Message Cluster"), "Message"="MFC_2", "Message Data"=w2602) -> (w2605:T4)
            n1115 = Enqueue Element(queue=w2604, element=w2605, error in (no error)=w2603) -> (queue out=w2601:refnum<queue>, error out=w2600:errorcluster)  [unwired: 1 in, 1 out]
          }
          frame #7 {
            w2610 = FALSE ("SO2 Flush")
            n1116 = local write "eV8"(w2610) -> ()
            n1117 = local write "eV9"(w2610) -> ()
          }
          frame #8 {
            n1118 = for {
              N: "Auto Zeroing \ninterval (sec)" -> [w2626]
              tunnel: [w2621] -> w2611
              i -> [w2625]
              stop <- w2621 stop-if-true
              n1119 = local read "SO2 Pause\nAuto Zeroing"() -> (w2619:bool)
              n1120 = Subtract(x=w2626, y=w2625) -> (x-y=w2627:i32)
              n1121 = Equal?(x=w2619, y=TRUE) -> (x = y?=w2617:bool)
              n1122 = Decrement(x=w2627) -> (x-1=→"Next Auto Zero\nStarts in (sec)":i32)
              n1123 = Wait (ms)(milliseconds to wait=u32 1000) -> ()  [unwired: 1 out]
              n1124 = case shown="True" w2617 {
                selector: w2617 -> [w2629 _]
                tunnel: [w2629 FALSE] -> w2616
                frame False {
                }
                frame True {
                  n1125 = for {
                    N: "Pause Auto Zero Count \nDown set time (sec)" -> [w2643]
                    tunnel: [w2635] -> w2631
                    i -> [w2642]
                    stop <- w2635 stop-if-true
                    w2636 = FALSE
                    n1126 = local read "SO2 Pause\nAuto Zeroing"() -> (w2638:bool)
                    n1127 = local read "SO2 Auto Zeroing"() -> (w2639:bool)
                    n1128 = Subtract(x=w2643, y=w2642) -> (x-y=w2644:i32)
                    n1129 = Decrement(x=w2644) -> (x-1=→"SO2 Resume Zeroing\nCount down timer (sec)":i32)
                    n1130 = Wait (ms)(milliseconds to wait=u32 1000) -> ()  [unwired: 1 out]
                    n1131 = Equal?(x=w2639, y=w2636) -> (x = y?=w2640:bool)
                    n1132 = Equal?(x=w2638, y=w2636) -> (x = y?=w2637:bool)
                    n1133 = Or(x=w2640, y=w2637) -> (x .or. y?=w2635:bool)
                  }
                  n1134 = case shown="True" w2631 {
                    frame False {
                    }
                    frame True {
                      n1135 = local write "SO2 Resume Zeroing\nCount down timer (sec)"(u32 0 ("SO2 Resume Zeroing\nCount down timer (sec)")) -> ()
                    }
                  }
                  n1136 = local write "Auto Zero\nIndicator"("Auto Zero Paused" ("Auto Zero\nIndicator")) -> ()
                }
              }
              n1137 = local write "Auto Zero\nIndicator"("Waiting For The Next Zeroing\nInterrupt Waiting by Pressing Pause Auto Zeroing button " ("Auto Zero\nIndicator")) -> ()
              n1138 = local read "SO2 Auto Zeroing"() -> (w2622:bool)
              n1139 = local write "SO2 Pause\nAuto Zeroing"(w2616) -> ()
              n1140 = Equal?(x=w2622, y=FALSE) -> (x = y?=w2621:bool)
            }
            n1141 = case shown="True" w2611 {
              frame False {
              }
              frame True {
                n1142 = local write "Next Auto Zero\nStarts in (sec)"(u32 0 ("Next Auto Zero\nStarts in (sec)")) -> ()
              }
            }
          }
          frame #9 {
            n1143 = local write "SO2 Calibration Abort"(FALSE) -> ()
            n1144 = Bundle(cluster=T4 {"Message"="", "Message Data"=variant} ("Message Cluster"), "Message"="Auto_zero", "Message Data"=FALSE) -> (w2651:T4)
            n1145 = Enqueue Element(queue=w2648, element=w2651, error in (no error)=w2647) -> ()  [unwired: 1 in, 3 out]
          }
        }
      }
    }
    n1146 = Wait (ms)(milliseconds to wait=u32 100) -> ()  [unwired: 1 out]
  }
  n1147 = while {
    tunnel: w4 -> [w2660]
    shift-right: [w2655] -> _
    shift-left: w43 -> [w2657]
    shift-right: [w2653] -> w41
    shift-left: w44 -> [w2659]
    tunnel: w3 -> [w2654]
    stop <- w2653 stop-if-true
    # "SO2 UI Command Sender"
    n1148 = Dequeue Element(queue=w2660, error in (no error)=w2654) -> (element=w2656:T4)  [unwired: 1 in, 3 out]
    n1149 = Unbundle By Name(w2656) -> ("Message"=w2658:string)
    n1150 = case shown="\"zeroing_interval\"" w2658 {
      tunnel: w2659 -> [w2661 w2665 w2672 w2679 w2686 w2693 w2700 w2707 w2714 w2721 w2728 w2735 w2742 w2749 w2756 w2763 w2770 w2777 w2784 w2791 w2798 w2805 w2812 w2819 w2826 w2833]
      tunnel: w2657 -> [w2662 w2668 w2675 w2682 w2689 w2696 w2703 w2710 w2717 w2724 w2731 w2738 w2745 w2752 w2759 w2766 w2773 w2780 w2787 w2794 w2801 w2808 w2815 w2822 w2829 w2836]
      tunnel: w2656 -> [_ w2667 w2674 w2681 w2688 w2695 w2702 w2709 w2716 w2723 w2730 w2737 w2744 w2751 w2758 w2765 w2772 w2779 w2786 w2793 w2800 w2807 w2814 w2821 w2828 w2835]
      tunnel: [w2661 w2664 w2671 w2678 w2685 w2692 w2699 w2706 w2713 w2720 w2727 w2734 w2741 w2748 w2755 w2762 w2769 w2776 w2783 w2790 w2797 w2804 w2811 w2818 w2825 w2832] -> w2653
      tunnel: [w2662 w2663 w2670 w2677 w2684 w2691 w2698 w2705 w2712 w2719 w2726 w2733 w2740 w2747 w2754 w2761 w2768 w2775 w2782 w2789 w2796 w2803 w2810 w2817 w2824 w2831] -> w2655
      frame "False", Default {
      }
      frame "V9" {
        n1151 = shared-variable-write(w2668, w2665, w2667) -> (w2666:refnum<k21>, w2669:errorcluster)  [unwired: 1 in, 1 out]
        n1152 = Flush Stream(8:w2669, 11:w2666) -> (0:w2664:errorcluster, 3:w2663:refnum<k21>)  [unwired: 2 in, 1 out]
      }
      frame "MFC_2" {
        n1153 = shared-variable-write(w2675, w2672, w2674) -> (w2673:refnum<k21>, w2676:errorcluster)  [unwired: 1 in, 1 out]
        n1154 = Flush Stream(8:w2676, 11:w2673) -> (0:w2671:errorcluster, 3:w2670:refnum<k21>)  [unwired: 2 in, 1 out]
      }
      frame "MFC_3" {
        n1155 = shared-variable-write(w2682, w2679, w2681) -> (w2680:refnum<k21>, w2683:errorcluster)  [unwired: 1 in, 1 out]
        n1156 = Flush Stream(8:w2683, 11:w2680) -> (0:w2678:errorcluster, 3:w2677:refnum<k21>)  [unwired: 2 in, 1 out]
      }
      frame "V6" {
        n1157 = shared-variable-write(w2689, w2686, w2688) -> (w2687:refnum<k21>, w2690:errorcluster)  [unwired: 1 in, 1 out]
        n1158 = Flush Stream(8:w2690, 11:w2687) -> (0:w2685:errorcluster, 3:w2684:refnum<k21>)  [unwired: 2 in, 1 out]
      }
      frame "Simulate Conc" {
        n1159 = shared-variable-write(w2696, w2693, w2695) -> (w2694:refnum<k21>, w2697:errorcluster)  [unwired: 1 in, 1 out]
        n1160 = Flush Stream(8:w2697, 11:w2694) -> (0:w2692:errorcluster, 3:w2691:refnum<k21>)  [unwired: 2 in, 1 out]
      }
      frame "Simulate STEL Conc" {
        n1161 = shared-variable-write(w2703, w2700, w2702) -> (w2701:refnum<k21>, w2704:errorcluster)  [unwired: 1 in, 1 out]
        n1162 = Flush Stream(8:w2704, 11:w2701) -> (0:w2699:errorcluster, 3:w2698:refnum<k21>)  [unwired: 2 in, 1 out]
      }
      frame "Simulate TWA Conc" {
        n1163 = shared-variable-write(w2710, w2707, w2709) -> (w2708:refnum<k21>, w2711:errorcluster)  [unwired: 1 in, 1 out]
        n1164 = Flush Stream(8:w2711, 11:w2708) -> (0:w2706:errorcluster, 3:w2705:refnum<k21>)  [unwired: 2 in, 1 out]
      }
      frame "10mins STEL Limit" {
        n1165 = shared-variable-write(w2717, w2714, w2716) -> (w2715:refnum<k21>, w2718:errorcluster)  [unwired: 1 in, 1 out]
        n1166 = Flush Stream(8:w2718, 11:w2715) -> (0:w2713:errorcluster, 3:w2712:refnum<k21>)  [unwired: 2 in, 1 out]
      }
      frame "8hr TWA Limit" {
        n1167 = shared-variable-write(w2724, w2721, w2723) -> (w2722:refnum<k21>, w2725:errorcluster)  [unwired: 1 in, 1 out]
        n1168 = Flush Stream(8:w2725, 11:w2722) -> (0:w2720:errorcluster, 3:w2719:refnum<k21>)  [unwired: 2 in, 1 out]
      }
      frame "Offset" {
        n1169 = shared-variable-write(w2731, w2728, w2730) -> (w2729:refnum<k21>, w2732:errorcluster)  [unwired: 1 in, 1 out]
        n1170 = Flush Stream(8:w2732, 11:w2729) -> (0:w2727:errorcluster, 3:w2726:refnum<k21>)  [unwired: 2 in, 1 out]
      }
      frame "eV8_user_set_time" {
        n1171 = shared-variable-write(w2738, w2735, w2737) -> (w2736:refnum<k21>, w2739:errorcluster)  [unwired: 1 in, 1 out]
        n1172 = Flush Stream(8:w2739, 11:w2736) -> (0:w2734:errorcluster, 3:w2733:refnum<k21>)  [unwired: 2 in, 1 out]
      }
      frame "mean_cal_status" {
        n1173 = shared-variable-write(w2745, w2742, w2744) -> (w2743:refnum<k21>, w2746:errorcluster)  [unwired: 1 in, 1 out]
        n1174 = Flush Stream(8:w2746, 11:w2743) -> (0:w2741:errorcluster, 3:w2740:refnum<k21>)  [unwired: 2 in, 1 out]
      }
      frame "SO2_MOCCA_Alarm" {
        n1175 = shared-variable-write(w2752, w2749, w2751) -> (w2750:refnum<k21>, w2753:errorcluster)  [unwired: 1 in, 1 out]
        n1176 = Flush Stream(8:w2753, 11:w2750) -> (0:w2748:errorcluster, 3:w2747:refnum<k21>)  [unwired: 2 in, 1 out]
      }
      frame "MOCCA_window_delay_time" {
        n1177 = shared-variable-write(w2759, w2756, w2758) -> (w2757:refnum<k21>, w2760:errorcluster)  [unwired: 1 in, 1 out]
        n1178 = Flush Stream(8:w2760, 11:w2757) -> (0:w2755:errorcluster, 3:w2754:refnum<k21>)  [unwired: 2 in, 1 out]
      }
      frame "MOCCA_limit" {
        n1179 = shared-variable-write(w2766, w2763, w2765) -> (w2764:refnum<k21>, w2767:errorcluster)  [unwired: 1 in, 1 out]
        n1180 = Flush Stream(8:w2767, 11:w2764) -> (0:w2762:errorcluster, 3:w2761:refnum<k21>)  [unwired: 2 in, 1 out]
      }
      frame "calcon_save" {
        n1181 = shared-variable-write(w2773, w2770, w2772) -> (w2771:refnum<k21>, w2774:errorcluster)  [unwired: 1 in, 1 out]
        n1182 = Flush Stream(8:w2774, 11:w2771) -> (0:w2769:errorcluster, 3:w2768:refnum<k21>)  [unwired: 2 in, 1 out]
      }
      frame "Auto_zero" {
        n1183 = shared-variable-write(w2780, w2777, w2779) -> (w2778:refnum<k21>, w2781:errorcluster)  [unwired: 1 in, 1 out]
        n1184 = Flush Stream(8:w2781, 11:w2778) -> (0:w2776:errorcluster, 3:w2775:refnum<k21>)  [unwired: 2 in, 1 out]
      }
      frame "zeroing_interval" {
        n1185 = shared-variable-write(w2787, w2784, w2786) -> (w2785:refnum<k21>, w2788:errorcluster)  [unwired: 1 in, 1 out]
        n1186 = Flush Stream(8:w2788, 11:w2785) -> (0:w2783:errorcluster, 3:w2782:refnum<k21>)  [unwired: 2 in, 1 out]
      }
      frame "cal_gas_cylin_conc" {
        n1187 = shared-variable-write(w2794, w2791, w2793) -> (w2792:refnum<k21>, w2795:errorcluster)  [unwired: 1 in, 1 out]
        n1188 = Flush Stream(8:w2795, 11:w2792) -> (0:w2790:errorcluster, 3:w2789:refnum<k21>)  [unwired: 2 in, 1 out]
      }
      frame "sim_MOCCA_conc" {
        n1189 = shared-variable-write(w2801, w2798, w2800) -> (w2799:refnum<k21>, w2802:errorcluster)  [unwired: 1 in, 1 out]
        n1190 = Flush Stream(8:w2802, 11:w2799) -> (0:w2797:errorcluster, 3:w2796:refnum<k21>)  [unwired: 2 in, 1 out]
      }
      frame "Slope" {
        n1191 = shared-variable-write(w2808, w2805, w2807) -> (w2806:refnum<k21>, w2809:errorcluster)  [unwired: 1 in, 1 out]
        n1192 = Flush Stream(8:w2809, 11:w2806) -> (0:w2804:errorcluster, 3:w2803:refnum<k21>)  [unwired: 2 in, 1 out]
      }
      frame "Flight Number" {
        n1193 = shared-variable-write(w2815, w2812, w2814) -> (w2813:refnum<k21>, w2816:errorcluster)  [unwired: 1 in, 1 out]
        n1194 = Flush Stream(8:w2816, 11:w2813) -> (0:w2811:errorcluster, 3:w2810:refnum<k21>)  [unwired: 2 in, 1 out]
      }
      frame "Stop File Write" {
        n1195 = shared-variable-write(w2822, w2819, w2821) -> (w2820:refnum<k21>, w2823:errorcluster)  [unwired: 1 in, 1 out]
        n1196 = Flush Stream(8:w2823, 11:w2820) -> (0:w2818:errorcluster, 3:w2817:refnum<k21>)  [unwired: 2 in, 1 out]
      }
      frame "UDP Time Offset" {
        n1197 = shared-variable-write(w2829, w2826, w2828) -> (w2827:refnum<k21>, w2830:errorcluster)  [unwired: 1 in, 1 out]
        n1198 = Flush Stream(8:w2830, 11:w2827) -> (0:w2825:errorcluster, 3:w2824:refnum<k21>)  [unwired: 2 in, 1 out]
      }
      frame "V8" {
        n1199 = shared-variable-write(w2836, w2833, w2835) -> (w2834:refnum<k21>, w2837:errorcluster)  [unwired: 1 in, 1 out]
        n1200 = Flush Stream(8:w2837, 11:w2834) -> (0:w2832:errorcluster, 3:w2831:refnum<k21>)  [unwired: 2 in, 1 out]
      }
    }
  }
  "SO2 command sender \nerror out" <- w41
  n1201 = Obtain Queue(name (unnamed)="TEi43c_Command", element data type=w29) -> (queue out=w38:refnum<queue>, error out=w31:errorcluster)  [unwired: 3 in, 1 out]
  n1202 = Create Network Stream Writer Endpoint(6:w35, 7:10 ("writer buffer size"), 9:w29, 10:"//192.168.101.17/command/reader/TEi43c" ("reader url"), 11:"/command/writer/TEi43c" ("writer name")) -> (0:w34:errorcluster, 3:w33:refnum<k21>)  [unwired: 2 in]
  n1203 = while {
    tunnel: w38 -> [w2841]
    tunnel: w31 -> [w2840]
    tunnel: [w2838] -> _
    stop <- FALSE stop-if-true
    # "TEi43c Ozone UI Event Handler Loop"
    n1204 = event shown="[0] \"Ozone Zeroing\": Value Change" {
      selector: _ -> [_ _ _ _ _]
      dyn-events: _ -> [_ _ _ _ _]
      timeout: _ -> [_ _ _ _ _]
      tunnel: w2841 -> [w2849 w2887 w2895 w2902 w2910]
      tunnel: w2840 -> [w2848 w2886 w2894 w2901 w2909]
      tunnel: [w2847 w2885 w2893 w2900 w2908] -> w2838
      event "Ozone Zeroing": Value Change {
        n1205 = event-data() -> ()  [unwired: 1 in, 6 out]
        n1206 = flat-sequence {
          tunnel: w2849 -> [w2854]
          tunnel: w2848 -> [w2853]
          tunnel: [w2852] -> w2846
          tunnel: [w2850] -> w2842
          tunnel: w2846 -> [w2860]
          tunnel: [w2860] -> w2845
          tunnel: [w2858] -> w2843
          tunnel: w2842 -> [w2858]
          tunnel: w2845 -> [w2878]
          tunnel: [w2877] -> w2844
          tunnel: w2843 -> [w2879]
          tunnel: [w2884] -> w2847
          tunnel: w2844 -> [w2884]
          frame #0 {
            w2851 = TRUE
            n1207 = local write "Ozone eV6"(w2851) -> ()
            n1208 = Bundle(cluster=T4 {"Message"="", "Message Data"=variant} ("Message Cluster"), "Message"="V6", "Message Data"=w2851) -> (w2855:T4)
            n1209 = Enqueue Element(queue=w2854, element=w2855, error in (no error)=w2853) -> (queue out=w2850:refnum<queue>, error out=w2852:errorcluster)  [unwired: 1 in, 1 out]
          }
          frame #1 {
            # "10 Mins Count down"
            n1210 = for {
              N: 600 -> [w2870]
              i -> [w2869]
              stop <- w2862 stop-if-true
              n1211 = local read "Ozone Zeroing Abort"() -> (w2864:bool)
              n1212 = Subtract(x=w2870, y=w2869) -> (x-y=w2868:i32)
              n1213 = Decrement(x=w2868) -> (x-1=w2866:i32)
              n1214 = Wait (ms)(milliseconds to wait=u32 1000) -> ()  [unwired: 1 out]
              n1215 = case shown="True" w2864 {
                selector: w2864 -> [w2873 _]
                tunnel: [w2873 w2874] -> w2861
                frame False {
                }
                frame True {
                  n1216 = Two Button Dialog(message="Are you sure to abort Ozone Zeroing?") -> (T button?=w2874:bool)  [unwired: 2 in]
                }
              }
              n1217 = local read "Network disconnected"() -> (w2863:bool)
              n1218 = Or(x=w2863, y=w2861) -> (x .or. y?=w2862:bool)
              n1219 = Select(t=0, s=w2862, f=w2866) -> (s? t:f=→"Ozone Zeroing\nTime Remain (sec)":i32)
              n1220 = case shown="False" w2861 {
                selector: w2861 -> [w2872 _]
                frame False {
                  n1221 = local write "Ozone Zeroing Abort"(w2872) -> ()
                }
                frame True {
                }
              }
            }
          }
          frame #2 {
            w2876 = FALSE
            n1222 = local write "Ozone eV6"(w2876) -> ()
            n1223 = Bundle(cluster=T4 {"Message"="", "Message Data"=variant} ("Message Cluster"), "Message"="V6", "Message Data"=w2876) -> (w2880:T4)
            n1224 = Enqueue Element(queue=w2879, element=w2880, error in (no error)=w2878) -> (error out=w2877:errorcluster)  [unwired: 1 in, 2 out]
          }
          frame #3 {
            w2883 = FALSE ("Ozone Zeroing")
            n1225 = local write "Ozone Zeroing Abort"(w2883) -> ()
            n1226 = local write "Ozone Zeroing"(w2883) -> ()
          }
        }
      }
      event "Ozone eV6": Value Change {
        n1227 = event-data() -> ("NewVal"=w2888:bool)  [unwired: 1 in]
        n1228 = Bundle(cluster=T4 {"Message"="", "Message Data"=variant} ("Message Cluster"), "Message"="V6", "Message Data"=w2888) -> (w2889:T4)
        n1229 = Enqueue Element(queue=w2887, element=w2889, error in (no error)=w2886) -> (error out=w2885:errorcluster)  [unwired: 1 in, 2 out]
      }
      event "cRIO File IO Stop\n(USB Flash Drive Unmount)": Value Change {
        n1230 = event-data() -> ("NewVal"=w2892:bool)  [unwired: 1 in]
        n1231 = Bundle(cluster=T4 {"Message"="", "Message Data"=variant} ("Message Cluster"), "Message"="Stop File Write", "Message Data"=w2892) -> (w2896:T4)
        n1232 = Enqueue Element(queue=w2895, element=w2896, error in (no error)=w2894) -> (error out=w2893:errorcluster)  [unwired: 1 in, 2 out]
      }
      event "Ozone UDP Time Offset": Value Change {
        n1233 = event-data() -> ("NewVal"=w2899:i32)  [unwired: 1 in]
        n1234 = Bundle(cluster=T4 {"Message"="", "Message Data"=variant} ("Message Cluster"), "Message"="UDP Time Offset", "Message Data"=w2899) -> (w2903:T4)
        n1235 = Enqueue Element(queue=w2902, element=w2903, error in (no error)=w2901) -> (error out=w2900:errorcluster)  [unwired: 1 in, 2 out]
      }
      event "Confirm Flight Number": Value Change {
        n1236 = event-data() -> ()  [unwired: 1 in, 5 out]
        n1237 = flat-sequence {
          tunnel: w2909 -> [w2912]
          tunnel: w2910 -> [w2913]
          tunnel: [w2913] -> w2907
          tunnel: [w2912] -> w2906
          tunnel: [w2915] -> w2908
          tunnel: w2907 -> [w2917]
          tunnel: w2906 -> [w2916]
          frame #0 {
            n1238 = local write "cRIO File IO Stop\n(USB Flash Drive Unmount)"(FALSE ("cRIO File IO Stop\n(USB Flash Drive Unmount)")) -> ()
          }
          frame #1 {
            n1239 = local read "Flight Number"() -> (w2914:string)
            n1240 = Bundle(cluster=T4 {"Message"="", "Message Data"=variant} ("Message Cluster"), "Message"="Flight Number", "Message Data"=w2914) -> (w2918:T4)
            n1241 = Enqueue Element(queue=w2917, element=w2918, error in (no error)=w2916) -> (error out=w2915:errorcluster)  [unwired: 1 in, 2 out]
          }
        }
      }
    }
    "Ozone Event error out" <- w2838
  }
  n1242 = while {
    tunnel: w38 -> [w2928]
    shift-right: [w2923] -> _
    shift-left: w33 -> [w2925]
    shift-right: [w2921] -> w30
    shift-left: w34 -> [w2927]
    tunnel: w31 -> [w2922]
    stop <- w2921 stop-if-true
    # "TEi43c Ozone UI Command Sender"
    n1243 = Dequeue Element(queue=w2928, error in (no error)=w2922) -> (element=w2924:T4)  [unwired: 1 in, 3 out]
    n1244 = Unbundle By Name(w2924) -> ("Message"=w2926:string)
    n1245 = case shown="\"UDP Time Offset\"" w2926 {
      tunnel: w2927 -> [w2929 w2933 w2940 w2947 w2954]
      tunnel: w2925 -> [w2930 w2936 w2943 w2950 w2957]
      tunnel: w2924 -> [_ w2935 w2942 w2949 w2956]
      tunnel: [w2929 w2932 w2939 w2946 w2953] -> w2921
      tunnel: [w2930 w2931 w2938 w2945 w2952] -> w2923
      frame "False", Default {
      }
      frame "V6" {
        n1246 = shared-variable-write(w2936, w2933, w2935) -> (w2934:refnum<k21>, w2937:errorcluster)  [unwired: 1 in, 1 out]
        n1247 = Flush Stream(8:w2937, 11:w2934) -> (0:w2932:errorcluster, 3:w2931:refnum<k21>)  [unwired: 2 in, 1 out]
      }
      frame "Stop File Write" {
        n1248 = shared-variable-write(w2943, w2940, w2942) -> (w2941:refnum<k21>, w2944:errorcluster)  [unwired: 1 in, 1 out]
        n1249 = Flush Stream(8:w2944, 11:w2941) -> (0:w2939:errorcluster, 3:w2938:refnum<k21>)  [unwired: 2 in, 1 out]
      }
      frame "Flight Number" {
        n1250 = shared-variable-write(w2950, w2947, w2949) -> (w2948:refnum<k21>, w2951:errorcluster)  [unwired: 1 in, 1 out]
        n1251 = Flush Stream(8:w2951, 11:w2948) -> (0:w2946:errorcluster, 3:w2945:refnum<k21>)  [unwired: 2 in, 1 out]
      }
      frame "UDP Time Offset" {
        n1252 = shared-variable-write(w2957, w2954, w2956) -> (w2955:refnum<k21>, w2958:errorcluster)  [unwired: 1 in, 1 out]
        n1253 = Flush Stream(8:w2958, 11:w2955) -> (0:w2953:errorcluster, 3:w2952:refnum<k21>)  [unwired: 2 in, 1 out]
      }
    }
  }
  "Ozone command sender error out" <- w30
  n1254 = Obtain Queue(name (unnamed)="2BOzone_Command", element data type=w17) -> (queue out=w26:refnum<queue>, error out=w19:errorcluster)  [unwired: 3 in, 1 out]
  n1255 = Create Network Stream Writer Endpoint(6:w23, 7:10 ("writer buffer size"), 9:w17, 10:"//192.168.101.17/command/reader/2BOzone" ("reader url"), 11:"/command/writer/2BOzone" ("writer name")) -> (0:w22:errorcluster, 3:w21:refnum<k21>)  [unwired: 2 in]
  n1256 = while {
    tunnel: w26 -> [w2962]
    tunnel: w19 -> [w2961]
    tunnel: [w2959] -> _
    stop <- FALSE stop-if-true
    # "2BOzone UI Event Handler Loop"
    n1257 = event shown="[2] \"Simulate Inst Conc\": Value Change" {
      selector: _ -> [_ _ _ _ _ _ _ _]
      dyn-events: _ -> [_ _ _ _ _ _ _ _]
      timeout: _ -> [_ _ _ _ _ _ _ _]
      tunnel: w2962 -> [w2966 w2973 w2980 w2987 w2994 w3001 w3008 w3016]
      tunnel: w2961 -> [w2965 w2972 w2979 w2986 w2993 w3000 w3007 w3015]
      tunnel: [w2964 w2971 w2978 w2985 w2992 w2999 w3006 w3014] -> w2959
      event "Ambient = OFF\nCabin = ON": Value Change {
        n1258 = event-data() -> ("NewVal"=w2963:bool)  [unwired: 1 in]
        n1259 = Bundle(cluster=T4 {"Message"="", "Message Data"=variant} ("Message Cluster"), "Message"="Ambient/Cabin", "Message Data"=w2963) -> (w2967:T4)
        n1260 = Enqueue Element(queue=w2966, element=w2967, error in (no error)=w2965) -> (error out=w2964:errorcluster)  [unwired: 1 in, 2 out]
      }
      event "Simulate 2B Conc": Value Change {
        n1261 = event-data() -> ("NewVal"=w2970:bool)  [unwired: 1 in]
        n1262 = Bundle(cluster=T4 {"Message"="", "Message Data"=variant} ("Message Cluster"), "Message"="Simulate_conc", "Message Data"=w2970) -> (w2974:T4)
        n1263 = Enqueue Element(queue=w2973, element=w2974, error in (no error)=w2972) -> (error out=w2971:errorcluster)  [unwired: 1 in, 2 out]
      }
      event "Simulate Inst Conc": Value Change {
        n1264 = event-data() -> ("NewVal"=w2977:i32)  [unwired: 1 in]
        n1265 = Bundle(cluster=T4 {"Message"="", "Message Data"=variant} ("Message Cluster"), "Message"="Simulate_inst_conc", "Message Data"=w2977) -> (w2981:T4)
        n1266 = Enqueue Element(queue=w2980, element=w2981, error in (no error)=w2979) -> (error out=w2978:errorcluster)  [unwired: 1 in, 2 out]
      }
      event "Inst_alm_thresh": Value Change {
        n1267 = event-data() -> ("NewVal"=w2984:i32)  [unwired: 1 in]
        n1268 = Bundle(cluster=T4 {"Message"="", "Message Data"=variant} ("Message Cluster"), "Message"="Inst_alm_thresh", "Message Data"=w2984) -> (w2988:T4)
        n1269 = Enqueue Element(queue=w2987, element=w2988, error in (no error)=w2986) -> (error out=w2985:errorcluster)  [unwired: 1 in, 2 out]
      }
      event "3hr_alm_thresh": Value Change {
        n1270 = event-data() -> ("NewVal"=w2991:i32)  [unwired: 1 in]
        n1271 = Bundle(cluster=T4 {"Message"="", "Message Data"=variant} ("Message Cluster"), "Message"="3hr_alm_thresh", "Message Data"=w2991) -> (w2995:T4)
        n1272 = Enqueue Element(queue=w2994, element=w2995, error in (no error)=w2993) -> (error out=w2992:errorcluster)  [unwired: 1 in, 2 out]
      }
      event "Simulate 3hr Average Conc": Value Change {
        n1273 = event-data() -> ("NewVal"=w2998:dbl)  [unwired: 1 in]
        n1274 = Bundle(cluster=T4 {"Message"="", "Message Data"=variant} ("Message Cluster"), "Message"="Simulate_3hr_av_conc", "Message Data"=w2998) -> (w3002:T4)
        n1275 = Enqueue Element(queue=w3001, element=w3002, error in (no error)=w3000) -> (error out=w2999:errorcluster)  [unwired: 1 in, 2 out]
      }
      event "cRIO File IO Stop\n(USB Flash Drive Unmount)": Value Change {
        n1276 = event-data() -> ("NewVal"=w3005:bool)  [unwired: 1 in]
        n1277 = Bundle(cluster=T4 {"Message"="", "Message Data"=variant} ("Message Cluster"), "Message"="Stop File Write", "Message Data"=w3005) -> (w3009:T4)
        n1278 = Enqueue Element(queue=w3008, element=w3009, error in (no error)=w3007) -> (error out=w3006:errorcluster)  [unwired: 1 in, 2 out]
      }
      event "Confirm Flight Number": Value Change {
        n1279 = event-data() -> ()  [unwired: 1 in, 5 out]
        n1280 = flat-sequence {
          tunnel: w3015 -> [w3018]
          tunnel: w3016 -> [w3019]
          tunnel: [w3019] -> w3013
          tunnel: [w3018] -> w3012
          tunnel: [w3021] -> w3014
          tunnel: w3013 -> [w3023]
          tunnel: w3012 -> [w3022]
          frame #0 {
            n1281 = local write "cRIO File IO Stop\n(USB Flash Drive Unmount)"(FALSE ("cRIO File IO Stop\n(USB Flash Drive Unmount)")) -> ()
          }
          frame #1 {
            n1282 = local read "Flight Number"() -> (w3020:string)
            n1283 = Bundle(cluster=T4 {"Message"="", "Message Data"=variant} ("Message Cluster"), "Message"="Flight Number", "Message Data"=w3020) -> (w3024:T4)
            n1284 = Enqueue Element(queue=w3023, element=w3024, error in (no error)=w3022) -> (error out=w3021:errorcluster)  [unwired: 1 in, 2 out]
          }
        }
      }
    }
    "2BOzone Event error out" <- w2959
  }
  n1285 = while {
    tunnel: w26 -> [w3034]
    shift-right: [w3029] -> _
    shift-left: w21 -> [w3031]
    shift-right: [w3027] -> w18
    shift-left: w22 -> [w3033]
    tunnel: w19 -> [w3028]
    stop <- w3027 stop-if-true
    # "2BOzone UI Command Sender"
    n1286 = Dequeue Element(queue=w3034, error in (no error)=w3028) -> (element=w3030:T4)  [unwired: 1 in, 3 out]
    n1287 = Unbundle By Name(w3030) -> ("Message"=w3032:string)
    n1288 = case shown="\"3hr_alm_thresh\"" w3032 {
      tunnel: w3033 -> [w3035 w3039 w3046 w3053 w3060 w3067 w3074 w3081 w3088]
      tunnel: w3031 -> [w3036 w3042 w3049 w3056 w3063 w3070 w3077 w3084 w3091]
      tunnel: w3030 -> [_ w3041 w3048 w3055 w3062 w3069 w3076 w3083 w3090]
      tunnel: [w3035 w3038 w3045 w3052 w3059 w3066 w3073 w3080 w3087] -> w3027
      tunnel: [w3036 w3037 w3044 w3051 w3058 w3065 w3072 w3079 w3086] -> w3029
      frame "False", Default {
      }
      frame "Ambient/Cabin" {
        n1289 = shared-variable-write(w3042, w3039, w3041) -> (w3040:refnum<k21>, w3043:errorcluster)  [unwired: 1 in, 1 out]
        n1290 = Flush Stream(8:w3043, 11:w3040) -> (0:w3038:errorcluster, 3:w3037:refnum<k21>)  [unwired: 2 in, 1 out]
      }
      frame "Simulate_conc" {
        n1291 = shared-variable-write(w3049, w3046, w3048) -> (w3047:refnum<k21>, w3050:errorcluster)  [unwired: 1 in, 1 out]
        n1292 = Flush Stream(8:w3050, 11:w3047) -> (0:w3045:errorcluster, 3:w3044:refnum<k21>)  [unwired: 2 in, 1 out]
      }
      frame "Simulate_inst_conc" {
        n1293 = shared-variable-write(w3056, w3053, w3055) -> (w3054:refnum<k21>, w3057:errorcluster)  [unwired: 1 in, 1 out]
        n1294 = Flush Stream(8:w3057, 11:w3054) -> (0:w3052:errorcluster, 3:w3051:refnum<k21>)  [unwired: 2 in, 1 out]
      }
      frame "Inst_alm_thresh" {
        n1295 = shared-variable-write(w3063, w3060, w3062) -> (w3061:refnum<k21>, w3064:errorcluster)  [unwired: 1 in, 1 out]
        n1296 = Flush Stream(8:w3064, 11:w3061) -> (0:w3059:errorcluster, 3:w3058:refnum<k21>)  [unwired: 2 in, 1 out]
      }
      frame "3hr_alm_thresh" {
        n1297 = shared-variable-write(w3070, w3067, w3069) -> (w3068:refnum<k21>, w3071:errorcluster)  [unwired: 1 in, 1 out]
        n1298 = Flush Stream(8:w3071, 11:w3068) -> (0:w3066:errorcluster, 3:w3065:refnum<k21>)  [unwired: 2 in, 1 out]
      }
      frame "Simulate_3hr_av_conc" {
        n1299 = shared-variable-write(w3077, w3074, w3076) -> (w3075:refnum<k21>, w3078:errorcluster)  [unwired: 1 in, 1 out]
        n1300 = Flush Stream(8:w3078, 11:w3075) -> (0:w3073:errorcluster, 3:w3072:refnum<k21>)  [unwired: 2 in, 1 out]
      }
      frame "Stop File Write" {
        n1301 = shared-variable-write(w3084, w3081, w3083) -> (w3082:refnum<k21>, w3085:errorcluster)  [unwired: 1 in, 1 out]
        n1302 = Flush Stream(8:w3085, 11:w3082) -> (0:w3080:errorcluster, 3:w3079:refnum<k21>)  [unwired: 2 in, 1 out]
      }
      frame "Flight Number" {
        n1303 = shared-variable-write(w3091, w3088, w3090) -> (w3089:refnum<k21>, w3092:errorcluster)  [unwired: 1 in, 1 out]
        n1304 = Flush Stream(8:w3092, 11:w3089) -> (0:w3087:errorcluster, 3:w3086:refnum<k21>)  [unwired: 2 in, 1 out]
      }
    }
  }
  "2BOzone command sender error out" <- w18
